vi "15 Puzzle Game (LabVIEW 2021).vi"() -> ()   [LabVIEW 2021]
uses:
  <vilib>/Utility/miscctls.llb/LVPositionTypeDef.ctl
panel:
  out "Moves Number":dbl caption="Elapsed Time (s)" format="%#.1f"
  out "Reset":bool
  out "Status":enum16{"Idle", "Start", "Stop"}(ring)
  out "Elapsed Time (s)":dbl format="%#.1f"
  out "Result":bool
  out "Temp Position":cluster{"Left":dbl, "Top":dbl}
  in  "Stop":bool
  in  "New Game":bool
  out "Empty":cluster{"Left":dbl, "Top":dbl}
  out "Random Array":dbl[](array[numeric])
  in  "Key 15":bool
  in  "Key 14":bool
  in  "Key 13":bool
  in  "Key 12":bool
  in  "Key 11":bool
  in  "Key 10":bool
  in  "Key 9":bool
  in  "Key 8":bool
  in  "Key 7":bool
  in  "Key 6":bool
  in  "Key 5":bool
  in  "Key 4":bool
  in  "Key 3":bool
  in  "Key 2":bool
  in  "Key 1":bool
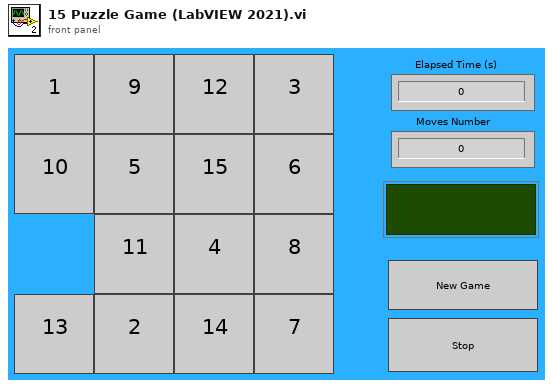
[diagram p1: front panel]
types:
  T1 = typedef "LVPositionTypeDef.ctl" = cluster{"Left":i32, "Top":i32}
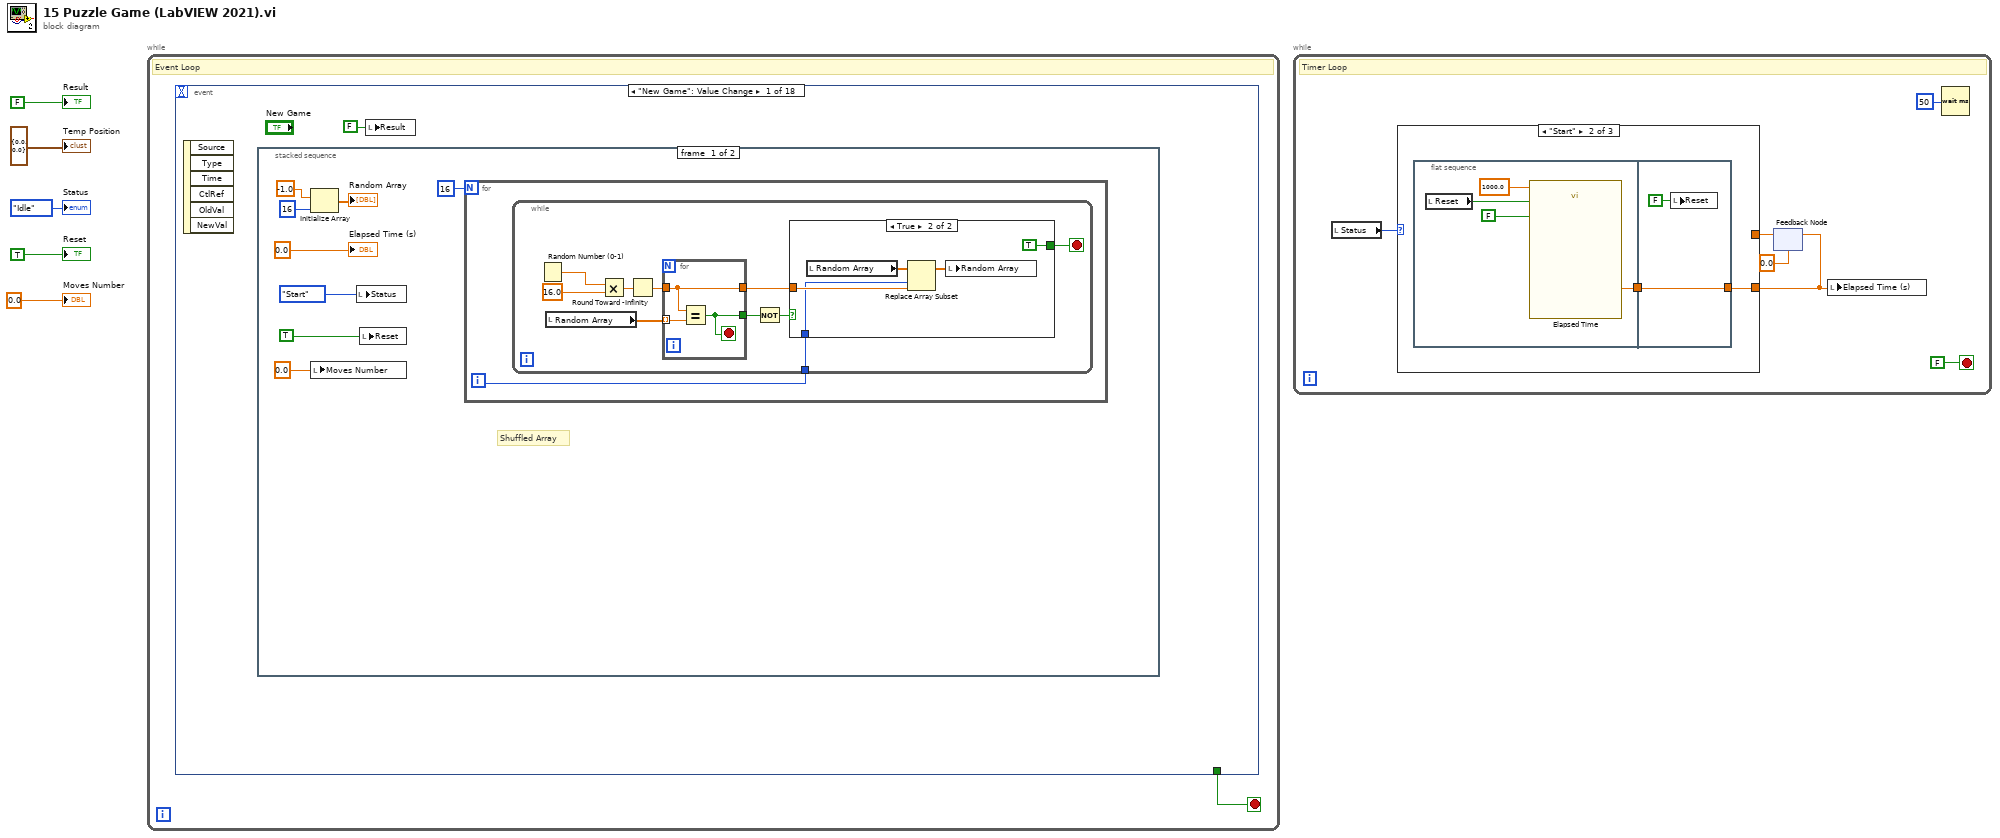
[diagram p0: block diagram]
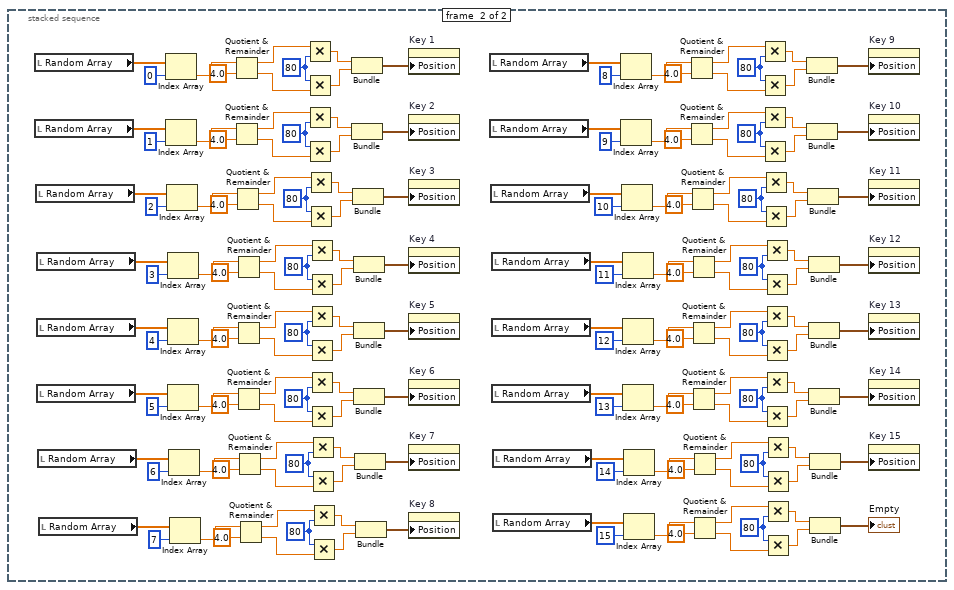
[diagram p5: hidden frame]
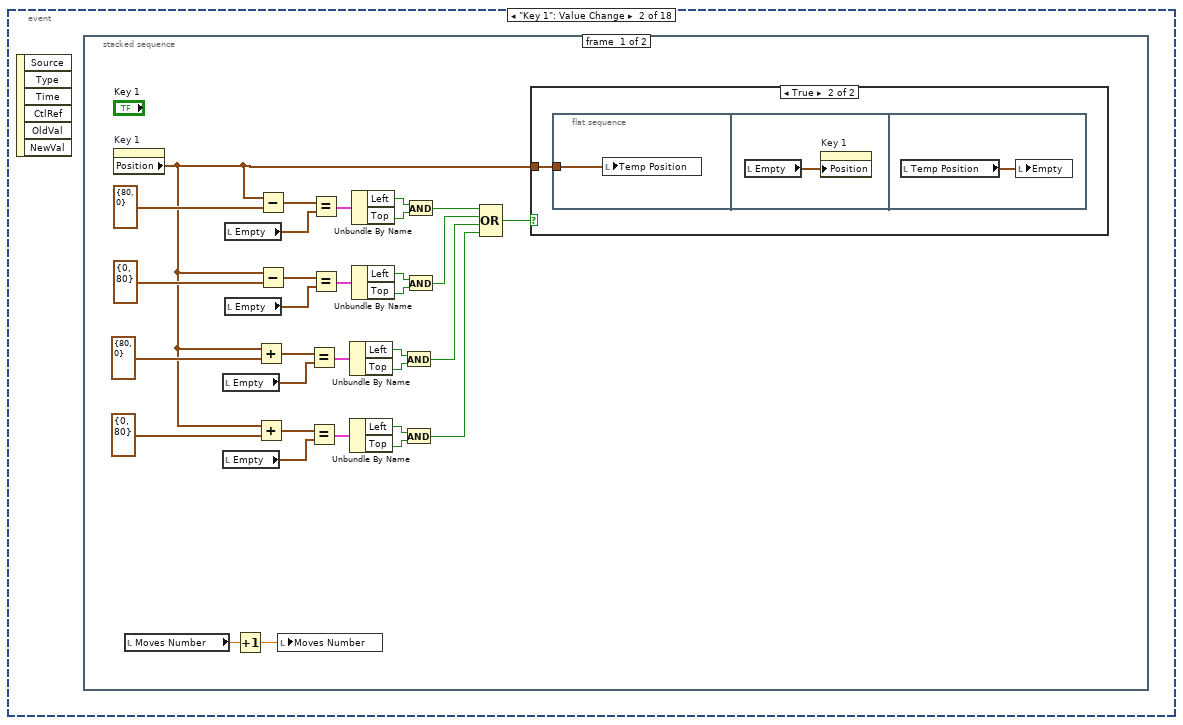
[diagram p6: hidden frame]
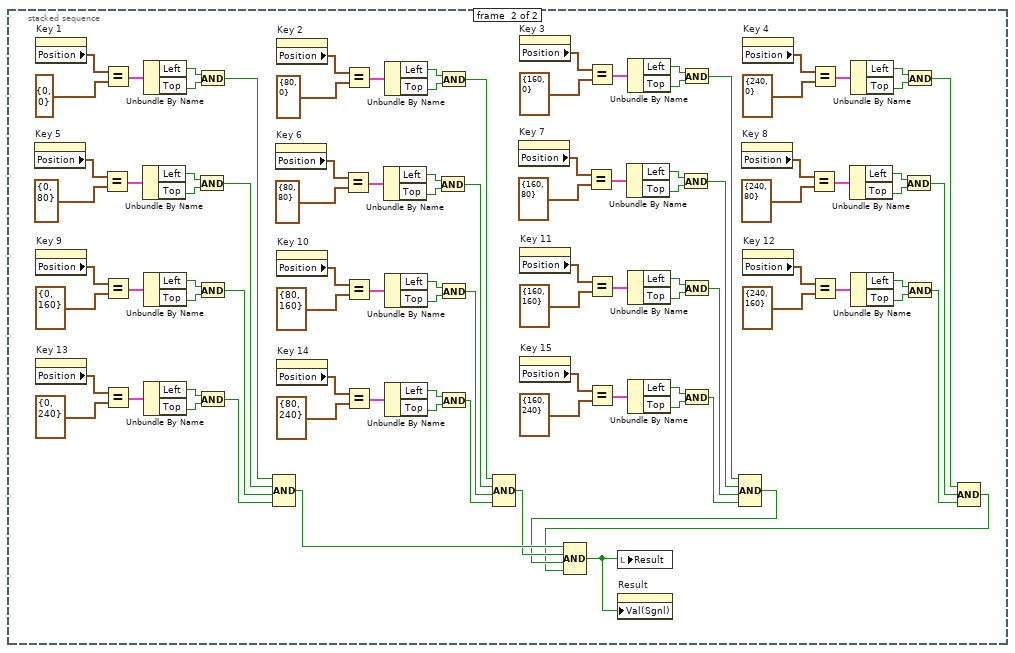
[diagram p8: hidden frame]
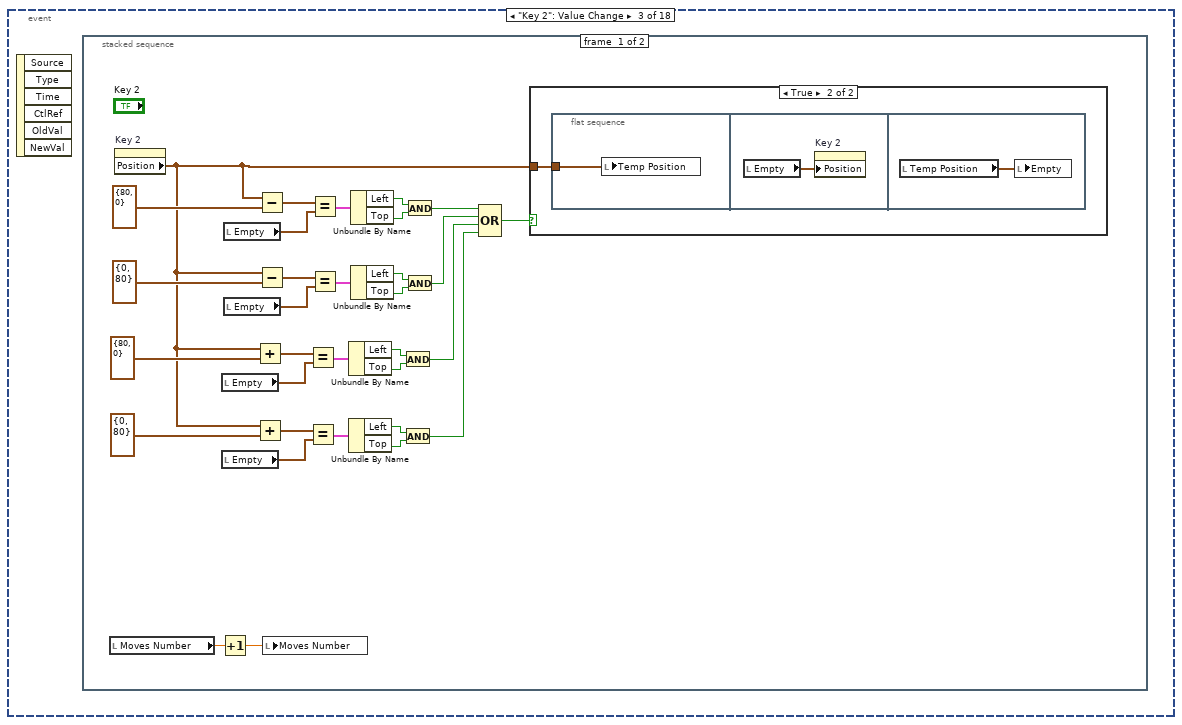
[diagram p9: hidden frame]
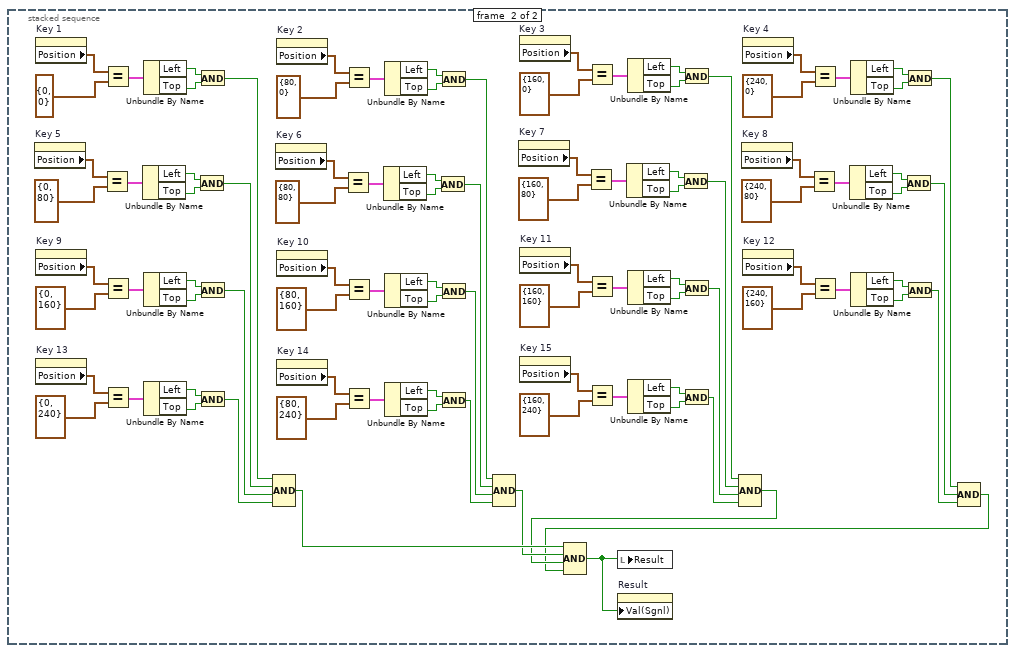
[diagram p11: hidden frame]
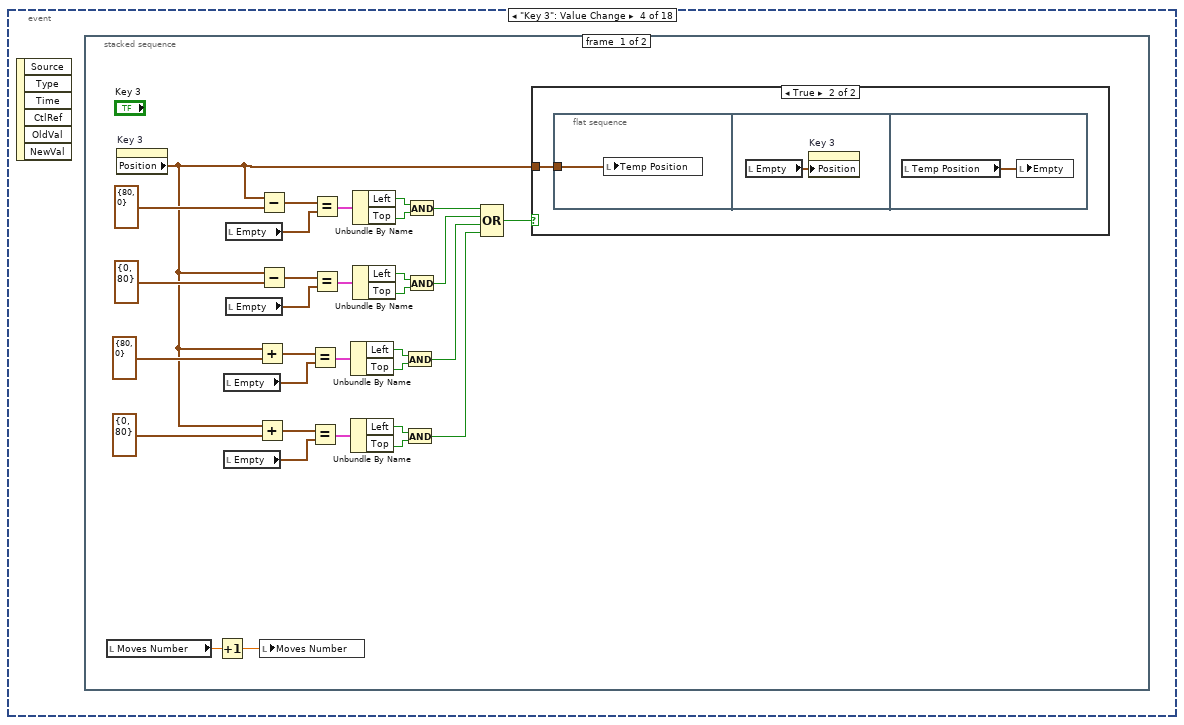
[diagram p12: hidden frame]
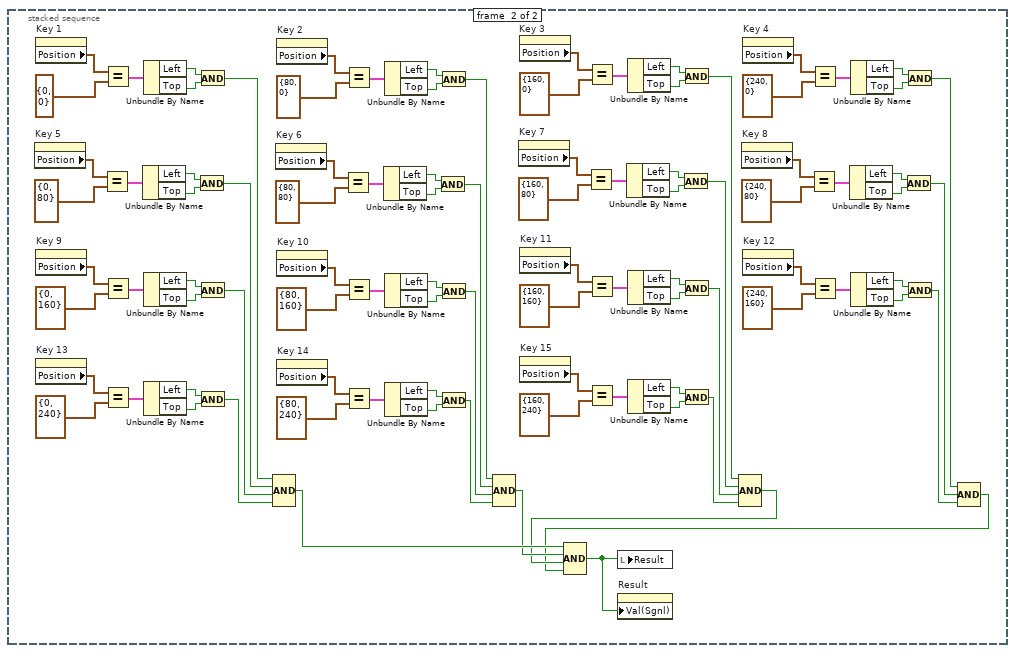
[diagram p14: hidden frame]
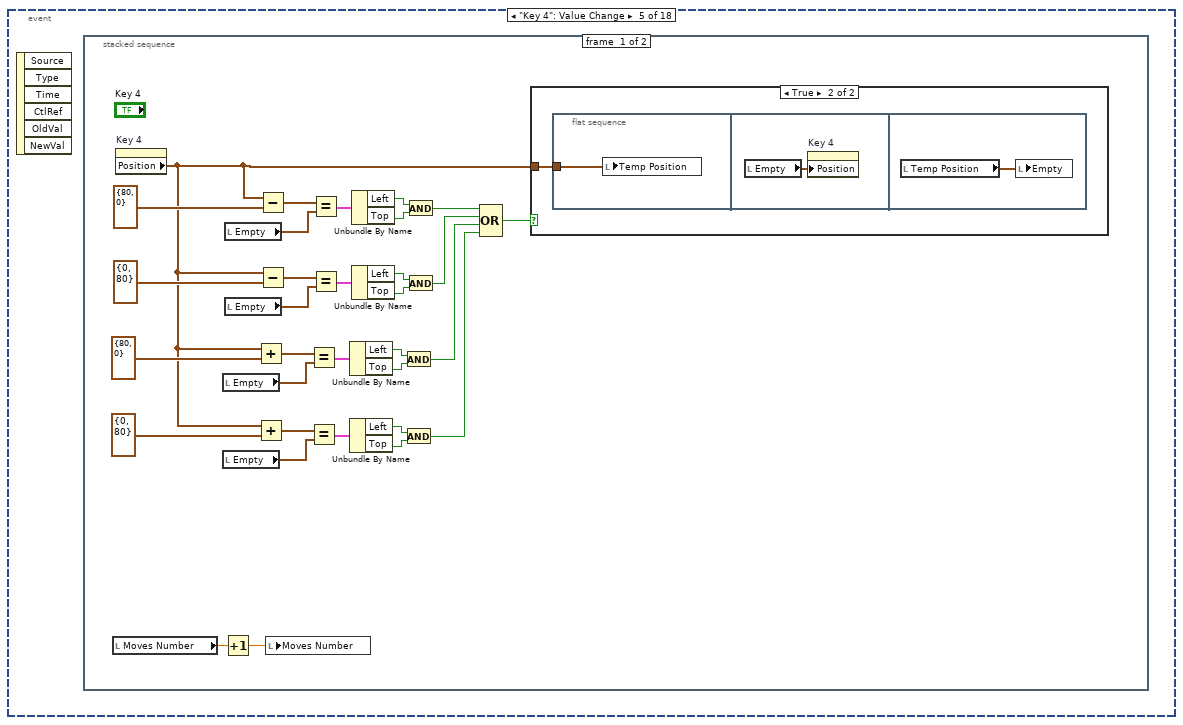
[diagram p15: hidden frame]
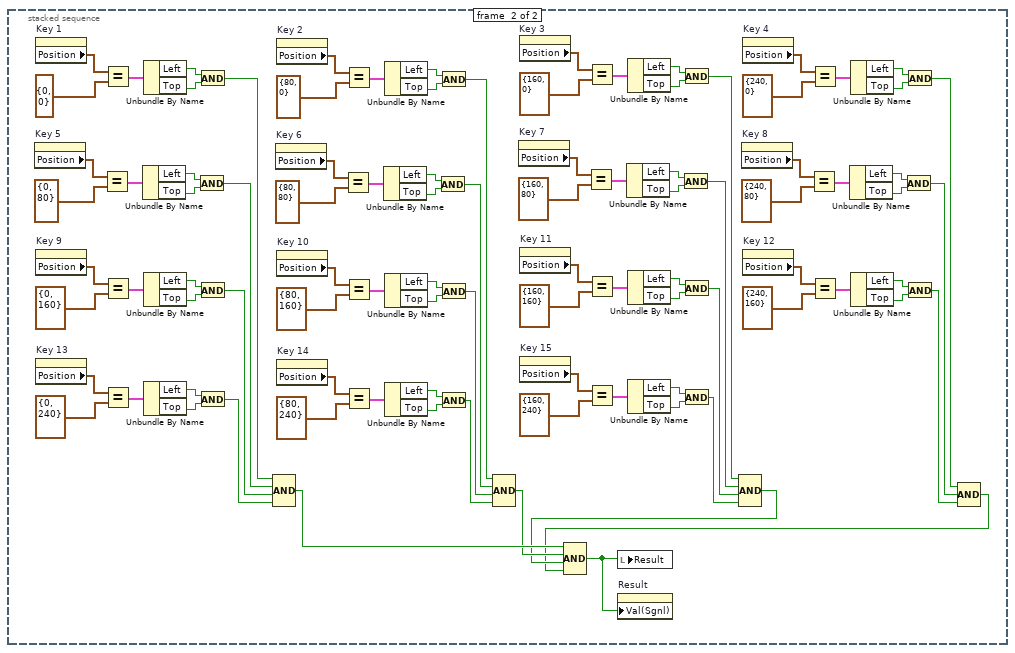
[diagram p17: hidden frame]
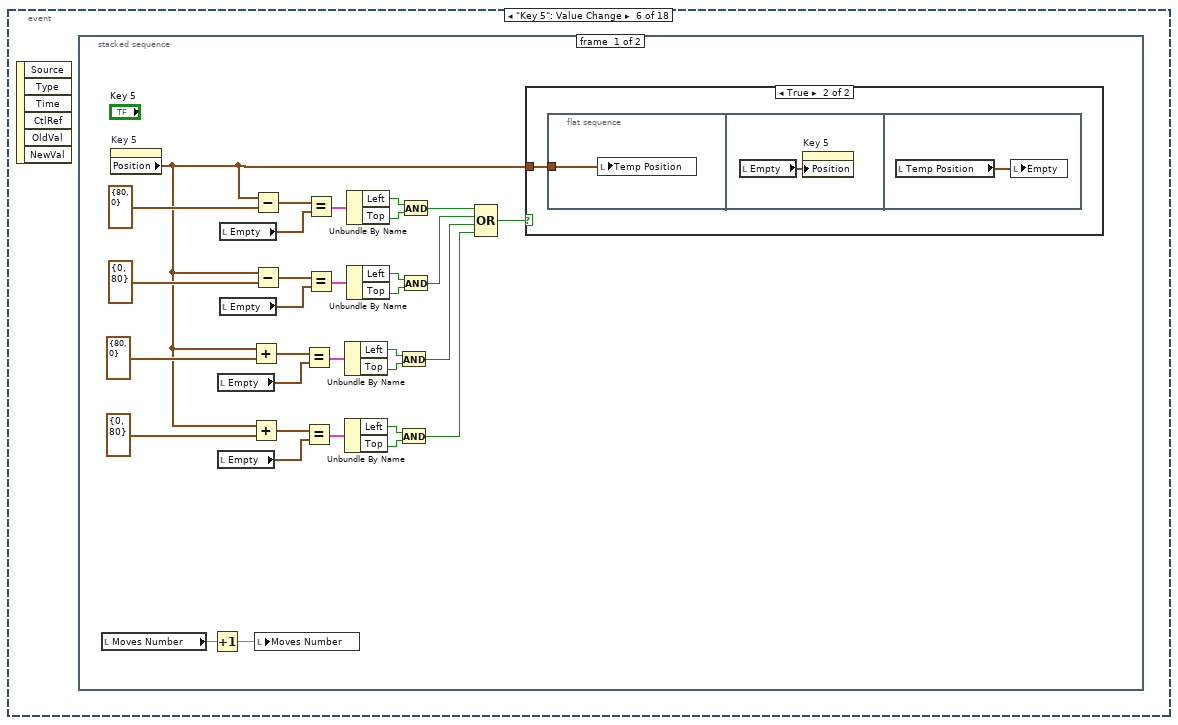
[diagram p18: hidden frame]
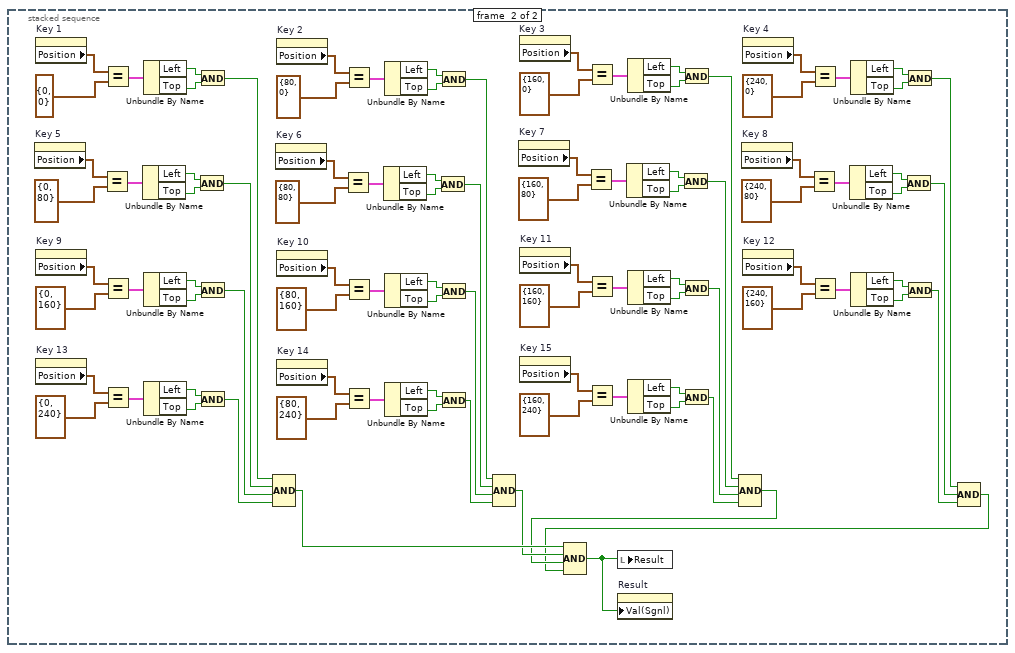
[diagram p20: hidden frame]
diagram:
  n1 = while {
    stop <- w6 stop-if-true
    # "Event Loop"
    n2 = event shown="[0] \"New Game\": Value Change" {
      selector: _ -> [_ _ _ _ _ _ _ _ _ _ _ _ _ _ _ _ _ _]
      dyn-events: _ -> [_ _ _ _ _ _ _ _ _ _ _ _ _ _ _ _ _ _]
      timeout: _ -> [_ _ _ _ _ _ _ _ _ _ _ _ _ _ _ _ _ _]
      tunnel: [_ _ _ _ _ _ _ _ _ _ _ _ _ _ _ _ _ TRUE] -> w6
      event "New Game": Value Change {
        n3 = event-data() -> ()  [unwired: 1 in, 6 out]
        n4 = stacked-sequence {
          frame #0 {
            # "Shuffled Array"
            n5 = Initialize Array(-1.0 ("element"), 16 ("dimension size")) -> (→"Random Array":dbl[])
            n6 = local write "Moves Number"(0.0 ("Moves Number")) -> ()
            n7 = local write "Status"(enum16{"Idle", "Start", "Stop"}."Start" ("Status")) -> ()
            n8 = local write "Reset"(TRUE ("Reset")) -> ()
            n9 = for {
              N: 16 -> [_]
              i -> [w16]
              n10 = while {
                tunnel: w16 -> [w17]
                stop <- w18 stop-if-true
                n11 = Random Number (0-1)() -> (number: 0 to 1=w21:dbl)
                n12 = local read "Random Array"() -> (w26:dbl[])
                n13 = Multiply(x=w21, y=16.0) -> (x*y=w22:dbl)
                n14 = Round Toward -Infinity(1:w22) -> (0:w19:dbl)
                n15 = for {
                  tunnel: w19 -> [w32]
                  tunnel: w26 -> [w34] mode=indexing
                  tunnel: [w33] -> w24
                  tunnel: [w32] -> w23
                  stop <- w33 stop-if-true
                  n16 = Equal?(x=w32, y=w34) -> (x = y?=w33:bool)
                }
                n17 = Not(x=w24) -> (.not. x?=w25:bool)
                n18 = case shown="True" w25 {
                  tunnel: w23 -> [_ w29]
                  tunnel: [_ TRUE] -> w18
                  tunnel: w17 -> [_ w27]
                  frame False {
                  }
                  frame True {
                    n19 = local read "Random Array"() -> (w31:dbl[])
                    n20 = Replace Array Subset(array=w31, new element=w29, index=w27) -> (w30:dbl[])
                    n21 = local write "Random Array"(w30) -> ()
                  }
                }
              }
            }
            "Elapsed Time (s)" <- 0.0 ("Elapsed Time (s)")
          }
          frame #1 {
            w42 = 80
            w88 = 80
            w101 = 80
            w108 = 80
            w78 = 80
            w71 = 80
            w58 = 80
            w51 = 80
            w148 = 80
            w141 = 80
            w128 = 80
            w121 = 80
            w161 = 80
            w168 = 80
            w181 = 80
            w188 = 80
            n22 = local read "Random Array"() -> (w194:dbl[])
            n23 = local read "Random Array"() -> (w175:dbl[])
            n24 = local read "Random Array"() -> (w174:dbl[])
            n25 = local read "Random Array"() -> (w155:dbl[])
            n26 = local read "Random Array"() -> (w115:dbl[])
            n27 = local read "Random Array"() -> (w134:dbl[])
            n28 = local read "Random Array"() -> (w135:dbl[])
            n29 = local read "Random Array"() -> (w154:dbl[])
            n30 = Index Array(array=w194, index=0) -> (element=w192:dbl)
            n31 = Index Array(array=w175, index=1) -> (element=w177:dbl)
            n32 = Index Array(array=w174, index=2) -> (element=w172:dbl)
            n33 = Index Array(array=w155, index=3) -> (element=w157:dbl)
            n34 = Index Array(array=w115, index=4) -> (element=w117:dbl)
            n35 = Index Array(array=w134, index=5) -> (element=w132:dbl)
            n36 = Index Array(array=w135, index=6) -> (element=w137:dbl)
            n37 = Index Array(array=w154, index=7) -> (element=w152:dbl)
            n38 = Quotient & Remainder(x=w192, y=4.0) -> (x-y*floor(x/y)=w190:dbl, floor(x/y)=w189:dbl)
            n39 = Quotient & Remainder(x=w177, y=4.0) -> (x-y*floor(x/y)=w179:dbl, floor(x/y)=w180:dbl)
            n40 = Quotient & Remainder(x=w172, y=4.0) -> (x-y*floor(x/y)=w170:dbl, floor(x/y)=w169:dbl)
            n41 = Quotient & Remainder(x=w157, y=4.0) -> (x-y*floor(x/y)=w159:dbl, floor(x/y)=w160:dbl)
            n42 = Quotient & Remainder(x=w117, y=4.0) -> (x-y*floor(x/y)=w119:dbl, floor(x/y)=w120:dbl)
            n43 = Quotient & Remainder(x=w132, y=4.0) -> (x-y*floor(x/y)=w130:dbl, floor(x/y)=w129:dbl)
            n44 = Quotient & Remainder(x=w137, y=4.0) -> (x-y*floor(x/y)=w139:dbl, floor(x/y)=w140:dbl)
            n45 = Quotient & Remainder(x=w152, y=4.0) -> (x-y*floor(x/y)=w150:dbl, floor(x/y)=w149:dbl)
            n46 = Multiply(x=w190, y=w188) -> (x*y=w187:dbl)
            n47 = Multiply(x=w188, y=w189) -> (x*y=w186:dbl)
            n48 = Multiply(x=w179, y=w181) -> (x*y=w182:dbl)
            n49 = Multiply(x=w181, y=w180) -> (x*y=w183:dbl)
            n50 = Multiply(x=w170, y=w168) -> (x*y=w167:dbl)
            n51 = Multiply(x=w168, y=w169) -> (x*y=w166:dbl)
            n52 = Multiply(x=w159, y=w161) -> (x*y=w162:dbl)
            n53 = Multiply(x=w161, y=w160) -> (x*y=w163:dbl)
            n54 = Multiply(x=w119, y=w121) -> (x*y=w122:dbl)
            n55 = Multiply(x=w121, y=w120) -> (x*y=w123:dbl)
            n56 = Multiply(x=w130, y=w128) -> (x*y=w127:dbl)
            n57 = Multiply(x=w128, y=w129) -> (x*y=w126:dbl)
            n58 = Multiply(x=w139, y=w141) -> (x*y=w142:dbl)
            n59 = Multiply(x=w141, y=w140) -> (x*y=w143:dbl)
            n60 = Multiply(x=w150, y=w148) -> (x*y=w147:dbl)
            n61 = Multiply(x=w148, y=w149) -> (x*y=w146:dbl)
            n62 = Bundle(w187, w186) -> (w185:cluster{dbl, dbl})  [unwired: 1 in]
            n63 = Bundle(w182, w183) -> (w184:cluster{dbl, dbl})  [unwired: 1 in]
            n64 = Bundle(w167, w166) -> (w165:cluster{dbl, dbl})  [unwired: 1 in]
            n65 = Bundle(w162, w163) -> (w164:cluster{dbl, dbl})  [unwired: 1 in]
            n66 = Bundle(w122, w123) -> (w124:cluster{dbl, dbl})  [unwired: 1 in]
            n67 = Bundle(w127, w126) -> (w125:cluster{dbl, dbl})  [unwired: 1 in]
            n68 = Bundle(w142, w143) -> (w144:cluster{dbl, dbl})  [unwired: 1 in]
            n69 = Bundle(w147, w146) -> (w145:cluster{dbl, dbl})  [unwired: 1 in]
            n70 = property on="Key 1" class="Bool"("Position"=w185) -> ()  [unwired: 2 in, 2 out]
            n71 = property on="Key 2" class="Bool"("Position"=w184) -> ()  [unwired: 2 in, 2 out]
            n72 = property on="Key 3" class="Bool"("Position"=w165) -> ()  [unwired: 2 in, 2 out]
            n73 = property on="Key 4" class="Bool"("Position"=w164) -> ()  [unwired: 2 in, 2 out]
            n74 = property on="Key 5" class="Bool"("Position"=w124) -> ()  [unwired: 2 in, 2 out]
            n75 = property on="Key 6" class="Bool"("Position"=w125) -> ()  [unwired: 2 in, 2 out]
            n76 = property on="Key 7" class="Bool"("Position"=w144) -> ()  [unwired: 2 in, 2 out]
            n77 = property on="Key 8" class="Bool"("Position"=w145) -> ()  [unwired: 2 in, 2 out]
            n78 = local read "Random Array"() -> (w45:dbl[])
            n79 = local read "Random Array"() -> (w64:dbl[])
            n80 = local read "Random Array"() -> (w65:dbl[])
            n81 = local read "Random Array"() -> (w84:dbl[])
            n82 = local read "Random Array"() -> (w114:dbl[])
            n83 = local read "Random Array"() -> (w95:dbl[])
            n84 = local read "Random Array"() -> (w94:dbl[])
            n85 = local read "Random Array"() -> (w36:dbl[])
            n86 = Index Array(array=w45, index=8) -> (element=w47:dbl)
            n87 = Index Array(array=w64, index=9) -> (element=w62:dbl)
            n88 = Index Array(array=w65, index=10) -> (element=w67:dbl)
            n89 = Index Array(array=w84, index=11) -> (element=w82:dbl)
            n90 = Index Array(array=w114, index=12) -> (element=w112:dbl)
            n91 = Index Array(array=w95, index=13) -> (element=w97:dbl)
            n92 = Index Array(array=w94, index=14) -> (element=w92:dbl)
            n93 = Index Array(array=w36, index=15) -> (element=w38:dbl)
            n94 = Quotient & Remainder(x=w47, y=4.0) -> (x-y*floor(x/y)=w49:dbl, floor(x/y)=w50:dbl)
            n95 = Quotient & Remainder(x=w62, y=4.0) -> (x-y*floor(x/y)=w60:dbl, floor(x/y)=w59:dbl)
            n96 = Quotient & Remainder(x=w67, y=4.0) -> (x-y*floor(x/y)=w69:dbl, floor(x/y)=w70:dbl)
            n97 = Quotient & Remainder(x=w82, y=4.0) -> (x-y*floor(x/y)=w80:dbl, floor(x/y)=w79:dbl)
            n98 = Quotient & Remainder(x=w112, y=4.0) -> (x-y*floor(x/y)=w110:dbl, floor(x/y)=w109:dbl)
            n99 = Quotient & Remainder(x=w97, y=4.0) -> (x-y*floor(x/y)=w99:dbl, floor(x/y)=w100:dbl)
            n100 = Quotient & Remainder(x=w92, y=4.0) -> (x-y*floor(x/y)=w90:dbl, floor(x/y)=w89:dbl)
            n101 = Quotient & Remainder(x=w38, y=4.0) -> (x-y*floor(x/y)=w40:dbl, floor(x/y)=w41:dbl)
            n102 = Multiply(x=w49, y=w51) -> (x*y=w52:dbl)
            n103 = Multiply(x=w51, y=w50) -> (x*y=w53:dbl)
            n104 = Multiply(x=w60, y=w58) -> (x*y=w57:dbl)
            n105 = Multiply(x=w58, y=w59) -> (x*y=w56:dbl)
            n106 = Multiply(x=w69, y=w71) -> (x*y=w72:dbl)
            n107 = Multiply(x=w71, y=w70) -> (x*y=w73:dbl)
            n108 = Multiply(x=w80, y=w78) -> (x*y=w77:dbl)
            n109 = Multiply(x=w78, y=w79) -> (x*y=w76:dbl)
            n110 = Multiply(x=w110, y=w108) -> (x*y=w107:dbl)
            n111 = Multiply(x=w108, y=w109) -> (x*y=w106:dbl)
            n112 = Multiply(x=w99, y=w101) -> (x*y=w102:dbl)
            n113 = Multiply(x=w101, y=w100) -> (x*y=w103:dbl)
            n114 = Multiply(x=w90, y=w88) -> (x*y=w87:dbl)
            n115 = Multiply(x=w88, y=w89) -> (x*y=w86:dbl)
            n116 = Multiply(x=w40, y=w42) -> (x*y=w43:dbl)
            n117 = Multiply(x=w42, y=w41) -> (x*y=w44:dbl)
            n118 = Bundle(w52, w53) -> (w54:cluster{dbl, dbl})  [unwired: 1 in]
            n119 = Bundle(w57, w56) -> (w55:cluster{dbl, dbl})  [unwired: 1 in]
            n120 = Bundle(w72, w73) -> (w74:cluster{dbl, dbl})  [unwired: 1 in]
            n121 = Bundle(w77, w76) -> (w75:cluster{dbl, dbl})  [unwired: 1 in]
            n122 = Bundle(w107, w106) -> (w105:cluster{dbl, dbl})  [unwired: 1 in]
            n123 = Bundle(w102, w103) -> (w104:cluster{dbl, dbl})  [unwired: 1 in]
            n124 = Bundle(w87, w86) -> (w85:cluster{dbl, dbl})  [unwired: 1 in]
            n125 = Bundle(w43, w44) -> (→"Empty":cluster{dbl, dbl})  [unwired: 1 in]
            n126 = property on="Key 9" class="Bool"("Position"=w54) -> ()  [unwired: 2 in, 2 out]
            n127 = property on="Key 10" class="Bool"("Position"=w55) -> ()  [unwired: 2 in, 2 out]
            n128 = property on="Key 11" class="Bool"("Position"=w74) -> ()  [unwired: 2 in, 2 out]
            n129 = property on="Key 12" class="Bool"("Position"=w75) -> ()  [unwired: 2 in, 2 out]
            n130 = property on="Key 13" class="Bool"("Position"=w105) -> ()  [unwired: 2 in, 2 out]
            n131 = property on="Key 14" class="Bool"("Position"=w104) -> ()  [unwired: 2 in, 2 out]
            n132 = property on="Key 15" class="Bool"("Position"=w85) -> ()  [unwired: 2 in, 2 out]
          }
        }
        n133 = local write "Result"(FALSE ("Result")) -> ()
      }
      event "Key 1": Value Change {
        n134 = event-data() -> ()  [unwired: 1 in, 6 out]
        n135 = stacked-sequence {
          frame #0 {
            n136 = property on="Key 1" class="Bool"() -> ("Position"=w197:T1)  [unwired: 2 in, 2 out]
            n137 = local read "Moves Number"() -> (w195:dbl)
            n138 = local read "Empty"() -> (w205:cluster{"Left":dbl, "Top":dbl})
            n139 = local read "Empty"() -> (w212:cluster{"Left":dbl, "Top":dbl})
            n140 = local read "Empty"() -> (w224:cluster{"Left":dbl, "Top":dbl})
            n141 = local read "Empty"() -> (w217:cluster{"Left":dbl, "Top":dbl})
            n142 = Increment(x=w195) -> (x+1=w196:dbl)
            n143 = Add(x=w197, y=T1 {"Left"=80, "Top"=0} ("Position")) -> (x+y=w204:T1)
            n144 = Add(x=w197, y=T1 {"Left"=0, "Top"=80} ("Position")) -> (x+y=w213:T1)
            n145 = Subtract(x=w197, y=T1 {"Left"=80, "Top"=0} ("Position")) -> (x-y=w225:T1)
            n146 = Subtract(x=w197, y=T1 {"Left"=0, "Top"=80} ("Position")) -> (x-y=w216:T1)
            n147 = local write "Moves Number"(w196) -> ()
            n148 = Equal?(x=w204, y=w205) -> (x = y?=w206:cluster{"Left":bool, "Top":bool})
            n149 = Equal?(x=w213, y=w212) -> (x = y?=w211:cluster{"Left":bool, "Top":bool})
            n150 = Equal?(x=w225, y=w224) -> (x = y?=w223:cluster{"Left":bool, "Top":bool})
            n151 = Equal?(x=w216, y=w217) -> (x = y?=w218:cluster{"Left":bool, "Top":bool})
            n152 = Unbundle By Name(w206) -> ("Left"=w208:bool, "Top"=w207:bool)
            n153 = Unbundle By Name(w211) -> ("Left"=w209:bool, "Top"=w210:bool)
            n154 = Unbundle By Name(w223) -> ("Left"=w221:bool, "Top"=w222:bool)
            n155 = Unbundle By Name(w218) -> ("Left"=w220:bool, "Top"=w219:bool)
            n156 = And(x=w208, y=w207) -> (x .and. y?=w199:bool)
            n157 = And(x=w209, y=w210) -> (x .and. y?=w198:bool)
            n158 = And(x=w221, y=w222) -> (x .and. y?=w201:bool)
            n159 = And(x=w220, y=w219) -> (x .and. y?=w200:bool)
            n160 = Compound Arithmetic op=OR(w201, w200, w199, w198) -> (w202:bool)
            n161 = case shown="True" w202 {
              tunnel: w197 -> [_ w227]
              frame False {
              }
              frame True {
                n162 = flat-sequence {
                  tunnel: w227 -> [w228]
                  frame #0 {
                    n163 = local write "Temp Position"(w228) -> ()
                  }
                  frame #1 {
                    n164 = local read "Empty"() -> (w229:cluster{"Left":dbl, "Top":dbl})
                    n165 = property on="Key 1" class="Bool"("Position"=w229) -> ()  [unwired: 2 in, 2 out]
                  }
                  frame #2 {
                    n166 = local read "Temp Position"() -> (w230:cluster{"Left":dbl, "Top":dbl})
                    n167 = local write "Empty"(w230) -> ()
                  }
                }
              }
            }
          }
          frame #1 {
            n168 = property on="Key 5" class="Bool"() -> ("Position"=w319:T1)  [unwired: 2 in, 2 out]
            n169 = property on="Key 1" class="Bool"() -> ("Position"=w322:T1)  [unwired: 2 in, 2 out]
            n170 = property on="Key 9" class="Bool"() -> ("Position"=w312:T1)  [unwired: 2 in, 2 out]
            n171 = property on="Key 13" class="Bool"() -> ("Position"=w309:T1)  [unwired: 2 in, 2 out]
            n172 = Equal?(x=w319, y=T1 {"Left"=0, "Top"=80} ("Position")) -> (x = y?=w316:cluster{"Left":bool, "Top":bool})
            n173 = Equal?(x=w322, y=T1 {"Left"=0, "Top"=0} ("Position")) -> (x = y?=w325:cluster{"Left":bool, "Top":bool})
            n174 = Equal?(x=w312, y=T1 {"Left"=0, "Top"=160} ("Position")) -> (x = y?=w315:cluster{"Left":bool, "Top":bool})
            n175 = Equal?(x=w309, y=T1 {"Left"=0, "Top"=240} ("Position")) -> (x = y?=w306:cluster{"Left":bool, "Top":bool})
            n176 = Unbundle By Name(w316) -> ("Left"=w318:bool, "Top"=w317:bool)
            n177 = Unbundle By Name(w325) -> ("Left"=w323:bool, "Top"=w324:bool)
            n178 = Unbundle By Name(w315) -> ("Left"=w313:bool, "Top"=w314:bool)
            n179 = Unbundle By Name(w306) -> ("Left"=w308:bool, "Top"=w307:bool)
            n180 = And(x=w318, y=w317) -> (x .and. y?=w249:bool)
            n181 = And(x=w323, y=w324) -> (x .and. y?=w250:bool)
            n182 = And(x=w313, y=w314) -> (x .and. y?=w248:bool)
            n183 = And(x=w308, y=w307) -> (x .and. y?=w247:bool)
            n184 = Compound Arithmetic op=AND(w250, w249, w248, w247) -> (w235:bool)
            n185 = property on="Key 6" class="Bool"() -> ("Position"=w292:T1)  [unwired: 2 in, 2 out]
            n186 = property on="Key 2" class="Bool"() -> ("Position"=w289:T1)  [unwired: 2 in, 2 out]
            n187 = property on="Key 10" class="Bool"() -> ("Position"=w299:T1)  [unwired: 2 in, 2 out]
            n188 = property on="Key 14" class="Bool"() -> ("Position"=w302:T1)  [unwired: 2 in, 2 out]
            n189 = Equal?(x=w292, y=T1 {"Left"=80, "Top"=80} ("Position")) -> (x = y?=w295:cluster{"Left":bool, "Top":bool})
            n190 = Equal?(x=w289, y=T1 {"Left"=80, "Top"=0} ("Position")) -> (x = y?=w286:cluster{"Left":bool, "Top":bool})
            n191 = Equal?(x=w299, y=T1 {"Left"=80, "Top"=160} ("Position")) -> (x = y?=w296:cluster{"Left":bool, "Top":bool})
            n192 = Equal?(x=w302, y=T1 {"Left"=80, "Top"=240} ("Position")) -> (x = y?=w305:cluster{"Left":bool, "Top":bool})
            n193 = Unbundle By Name(w295) -> ("Left"=w293:bool, "Top"=w294:bool)
            n194 = Unbundle By Name(w286) -> ("Left"=w288:bool, "Top"=w287:bool)
            n195 = Unbundle By Name(w296) -> ("Left"=w298:bool, "Top"=w297:bool)
            n196 = Unbundle By Name(w305) -> ("Left"=w303:bool, "Top"=w304:bool)
            n197 = And(x=w293, y=w294) -> (x .and. y?=w245:bool)
            n198 = And(x=w288, y=w287) -> (x .and. y?=w246:bool)
            n199 = And(x=w298, y=w297) -> (x .and. y?=w244:bool)
            n200 = And(x=w303, y=w304) -> (x .and. y?=w243:bool)
            n201 = Compound Arithmetic op=AND(w246, w245, w244, w243) -> (w234:bool)
            n202 = property on="Key 7" class="Bool"() -> ("Position"=w279:T1)  [unwired: 2 in, 2 out]
            n203 = property on="Key 3" class="Bool"() -> ("Position"=w282:T1)  [unwired: 2 in, 2 out]
            n204 = property on="Key 11" class="Bool"() -> ("Position"=w272:T1)  [unwired: 2 in, 2 out]
            n205 = property on="Key 15" class="Bool"() -> ("Position"=w269:T1)  [unwired: 2 in, 2 out]
            n206 = Equal?(x=w279, y=T1 {"Left"=160, "Top"=80} ("Position")) -> (x = y?=w276:cluster{"Left":bool, "Top":bool})
            n207 = Equal?(x=w282, y=T1 {"Left"=160, "Top"=0} ("Position")) -> (x = y?=w285:cluster{"Left":bool, "Top":bool})
            n208 = Equal?(x=w272, y=T1 {"Left"=160, "Top"=160} ("Position")) -> (x = y?=w275:cluster{"Left":bool, "Top":bool})
            n209 = Equal?(x=w269, y=T1 {"Left"=160, "Top"=240} ("Position")) -> (x = y?=w266:cluster{"Left":bool, "Top":bool})
            n210 = Unbundle By Name(w276) -> ("Left"=w278:bool, "Top"=w277:bool)
            n211 = Unbundle By Name(w285) -> ("Left"=w283:bool, "Top"=w284:bool)
            n212 = Unbundle By Name(w275) -> ("Left"=w273:bool, "Top"=w274:bool)
            n213 = Unbundle By Name(w266) -> ("Left"=w268:bool, "Top"=w267:bool)
            n214 = And(x=w278, y=w277) -> (x .and. y?=w241:bool)
            n215 = And(x=w283, y=w284) -> (x .and. y?=w242:bool)
            n216 = And(x=w273, y=w274) -> (x .and. y?=w240:bool)
            n217 = And(x=w268, y=w267) -> (x .and. y?=w239:bool)
            n218 = Compound Arithmetic op=AND(w242, w241, w240, w239) -> (w233:bool)
            n219 = property on="Key 8" class="Bool"() -> ("Position"=w257:T1)  [unwired: 2 in, 2 out]
            n220 = property on="Key 4" class="Bool"() -> ("Position"=w254:T1)  [unwired: 2 in, 2 out]
            n221 = property on="Key 12" class="Bool"() -> ("Position"=w264:T1)  [unwired: 2 in, 2 out]
            n222 = Equal?(x=w257, y=T1 {"Left"=240, "Top"=80} ("Position")) -> (x = y?=w260:cluster{"Left":bool, "Top":bool})
            n223 = Equal?(x=w254, y=T1 {"Left"=240, "Top"=0} ("Position")) -> (x = y?=w251:cluster{"Left":bool, "Top":bool})
            n224 = Equal?(x=w264, y=T1 {"Left"=240, "Top"=160} ("Position")) -> (x = y?=w261:cluster{"Left":bool, "Top":bool})
            n225 = Unbundle By Name(w260) -> ("Left"=w258:bool, "Top"=w259:bool)
            n226 = Unbundle By Name(w251) -> ("Left"=w253:bool, "Top"=w252:bool)
            n227 = Unbundle By Name(w261) -> ("Left"=w263:bool, "Top"=w262:bool)
            n228 = And(x=w258, y=w259) -> (x .and. y?=w237:bool)
            n229 = And(x=w253, y=w252) -> (x .and. y?=w238:bool)
            n230 = And(x=w263, y=w262) -> (x .and. y?=w236:bool)
            n231 = Compound Arithmetic op=AND(w238, w237, w236) -> (w232:bool)
            n232 = Compound Arithmetic op=AND(w235, w234, w233, w232) -> (w231:bool)
            n233 = local write "Result"(w231) -> ()
            n234 = property on="Result" class="Bool (strict)"("Val(Sgnl)"=w231) -> ()  [unwired: 2 in, 2 out]
          }
        }
      }
      event "Key 2": Value Change {
        n235 = event-data() -> ()  [unwired: 1 in, 6 out]
        n236 = stacked-sequence {
          frame #0 {
            n237 = local read "Moves Number"() -> (w326:dbl)
            n238 = property on="Key 2" class="Bool"() -> ("Position"=w328:T1)  [unwired: 2 in, 2 out]
            n239 = Increment(x=w326) -> (x+1=w327:dbl)
            n240 = local read "Empty"() -> (w336:cluster{"Left":dbl, "Top":dbl})
            n241 = local read "Empty"() -> (w343:cluster{"Left":dbl, "Top":dbl})
            n242 = local read "Empty"() -> (w355:cluster{"Left":dbl, "Top":dbl})
            n243 = local read "Empty"() -> (w348:cluster{"Left":dbl, "Top":dbl})
            n244 = Add(x=w328, y=T1 {"Left"=80, "Top"=0} ("Position")) -> (x+y=w335:T1)
            n245 = Add(x=w328, y=T1 {"Left"=0, "Top"=80} ("Position")) -> (x+y=w344:T1)
            n246 = Subtract(x=w328, y=T1 {"Left"=80, "Top"=0} ("Position")) -> (x-y=w356:T1)
            n247 = Subtract(x=w328, y=T1 {"Left"=0, "Top"=80} ("Position")) -> (x-y=w347:T1)
            n248 = local write "Moves Number"(w327) -> ()
            n249 = Equal?(x=w335, y=w336) -> (x = y?=w337:cluster{"Left":bool, "Top":bool})
            n250 = Equal?(x=w344, y=w343) -> (x = y?=w342:cluster{"Left":bool, "Top":bool})
            n251 = Equal?(x=w356, y=w355) -> (x = y?=w354:cluster{"Left":bool, "Top":bool})
            n252 = Equal?(x=w347, y=w348) -> (x = y?=w349:cluster{"Left":bool, "Top":bool})
            n253 = Unbundle By Name(w337) -> ("Left"=w339:bool, "Top"=w338:bool)
            n254 = Unbundle By Name(w342) -> ("Left"=w340:bool, "Top"=w341:bool)
            n255 = Unbundle By Name(w354) -> ("Left"=w352:bool, "Top"=w353:bool)
            n256 = Unbundle By Name(w349) -> ("Left"=w351:bool, "Top"=w350:bool)
            n257 = And(x=w339, y=w338) -> (x .and. y?=w330:bool)
            n258 = And(x=w340, y=w341) -> (x .and. y?=w329:bool)
            n259 = And(x=w352, y=w353) -> (x .and. y?=w332:bool)
            n260 = And(x=w351, y=w350) -> (x .and. y?=w331:bool)
            n261 = Compound Arithmetic op=OR(w332, w331, w330, w329) -> (w333:bool)
            n262 = case shown="True" w333 {
              tunnel: w328 -> [_ w358]
              frame False {
              }
              frame True {
                n263 = flat-sequence {
                  tunnel: w358 -> [w359]
                  frame #0 {
                    n264 = local write "Temp Position"(w359) -> ()
                  }
                  frame #1 {
                    n265 = local read "Empty"() -> (w360:cluster{"Left":dbl, "Top":dbl})
                    n266 = property on="Key 2" class="Bool"("Position"=w360) -> ()  [unwired: 2 in, 2 out]
                  }
                  frame #2 {
                    n267 = local read "Temp Position"() -> (w361:cluster{"Left":dbl, "Top":dbl})
                    n268 = local write "Empty"(w361) -> ()
                  }
                }
              }
            }
          }
          frame #1 {
            n269 = property on="Key 5" class="Bool"() -> ("Position"=w450:T1)  [unwired: 2 in, 2 out]
            n270 = property on="Key 1" class="Bool"() -> ("Position"=w453:T1)  [unwired: 2 in, 2 out]
            n271 = property on="Key 9" class="Bool"() -> ("Position"=w443:T1)  [unwired: 2 in, 2 out]
            n272 = property on="Key 13" class="Bool"() -> ("Position"=w440:T1)  [unwired: 2 in, 2 out]
            n273 = Equal?(x=w450, y=T1 {"Left"=0, "Top"=80} ("Position")) -> (x = y?=w447:cluster{"Left":bool, "Top":bool})
            n274 = Equal?(x=w453, y=T1 {"Left"=0, "Top"=0} ("Position")) -> (x = y?=w456:cluster{"Left":bool, "Top":bool})
            n275 = Equal?(x=w443, y=T1 {"Left"=0, "Top"=160} ("Position")) -> (x = y?=w446:cluster{"Left":bool, "Top":bool})
            n276 = Equal?(x=w440, y=T1 {"Left"=0, "Top"=240} ("Position")) -> (x = y?=w437:cluster{"Left":bool, "Top":bool})
            n277 = Unbundle By Name(w447) -> ("Left"=w449:bool, "Top"=w448:bool)
            n278 = Unbundle By Name(w456) -> ("Left"=w454:bool, "Top"=w455:bool)
            n279 = Unbundle By Name(w446) -> ("Left"=w444:bool, "Top"=w445:bool)
            n280 = Unbundle By Name(w437) -> ("Left"=w439:bool, "Top"=w438:bool)
            n281 = And(x=w449, y=w448) -> (x .and. y?=w380:bool)
            n282 = And(x=w454, y=w455) -> (x .and. y?=w381:bool)
            n283 = And(x=w444, y=w445) -> (x .and. y?=w379:bool)
            n284 = And(x=w439, y=w438) -> (x .and. y?=w378:bool)
            n285 = Compound Arithmetic op=AND(w381, w380, w379, w378) -> (w366:bool)
            n286 = property on="Key 6" class="Bool"() -> ("Position"=w423:T1)  [unwired: 2 in, 2 out]
            n287 = property on="Key 2" class="Bool"() -> ("Position"=w420:T1)  [unwired: 2 in, 2 out]
            n288 = property on="Key 10" class="Bool"() -> ("Position"=w430:T1)  [unwired: 2 in, 2 out]
            n289 = property on="Key 14" class="Bool"() -> ("Position"=w433:T1)  [unwired: 2 in, 2 out]
            n290 = Equal?(x=w423, y=T1 {"Left"=80, "Top"=80} ("Position")) -> (x = y?=w426:cluster{"Left":bool, "Top":bool})
            n291 = Equal?(x=w420, y=T1 {"Left"=80, "Top"=0} ("Position")) -> (x = y?=w417:cluster{"Left":bool, "Top":bool})
            n292 = Equal?(x=w430, y=T1 {"Left"=80, "Top"=160} ("Position")) -> (x = y?=w427:cluster{"Left":bool, "Top":bool})
            n293 = Equal?(x=w433, y=T1 {"Left"=80, "Top"=240} ("Position")) -> (x = y?=w436:cluster{"Left":bool, "Top":bool})
            n294 = Unbundle By Name(w426) -> ("Left"=w424:bool, "Top"=w425:bool)
            n295 = Unbundle By Name(w417) -> ("Left"=w419:bool, "Top"=w418:bool)
            n296 = Unbundle By Name(w427) -> ("Left"=w429:bool, "Top"=w428:bool)
            n297 = Unbundle By Name(w436) -> ("Left"=w434:bool, "Top"=w435:bool)
            n298 = And(x=w424, y=w425) -> (x .and. y?=w376:bool)
            n299 = And(x=w419, y=w418) -> (x .and. y?=w377:bool)
            n300 = And(x=w429, y=w428) -> (x .and. y?=w375:bool)
            n301 = And(x=w434, y=w435) -> (x .and. y?=w374:bool)
            n302 = Compound Arithmetic op=AND(w377, w376, w375, w374) -> (w365:bool)
            n303 = property on="Key 7" class="Bool"() -> ("Position"=w410:T1)  [unwired: 2 in, 2 out]
            n304 = property on="Key 3" class="Bool"() -> ("Position"=w413:T1)  [unwired: 2 in, 2 out]
            n305 = property on="Key 11" class="Bool"() -> ("Position"=w403:T1)  [unwired: 2 in, 2 out]
            n306 = property on="Key 15" class="Bool"() -> ("Position"=w400:T1)  [unwired: 2 in, 2 out]
            n307 = Equal?(x=w410, y=T1 {"Left"=160, "Top"=80} ("Position")) -> (x = y?=w407:cluster{"Left":bool, "Top":bool})
            n308 = Equal?(x=w413, y=T1 {"Left"=160, "Top"=0} ("Position")) -> (x = y?=w416:cluster{"Left":bool, "Top":bool})
            n309 = Equal?(x=w403, y=T1 {"Left"=160, "Top"=160} ("Position")) -> (x = y?=w406:cluster{"Left":bool, "Top":bool})
            n310 = Equal?(x=w400, y=T1 {"Left"=160, "Top"=240} ("Position")) -> (x = y?=w397:cluster{"Left":bool, "Top":bool})
            n311 = Unbundle By Name(w407) -> ("Left"=w409:bool, "Top"=w408:bool)
            n312 = Unbundle By Name(w416) -> ("Left"=w414:bool, "Top"=w415:bool)
            n313 = Unbundle By Name(w406) -> ("Left"=w404:bool, "Top"=w405:bool)
            n314 = Unbundle By Name(w397) -> ("Left"=w399:bool, "Top"=w398:bool)
            n315 = And(x=w409, y=w408) -> (x .and. y?=w372:bool)
            n316 = And(x=w414, y=w415) -> (x .and. y?=w373:bool)
            n317 = And(x=w404, y=w405) -> (x .and. y?=w371:bool)
            n318 = And(x=w399, y=w398) -> (x .and. y?=w370:bool)
            n319 = Compound Arithmetic op=AND(w373, w372, w371, w370) -> (w364:bool)
            n320 = property on="Key 8" class="Bool"() -> ("Position"=w388:T1)  [unwired: 2 in, 2 out]
            n321 = property on="Key 4" class="Bool"() -> ("Position"=w385:T1)  [unwired: 2 in, 2 out]
            n322 = property on="Key 12" class="Bool"() -> ("Position"=w395:T1)  [unwired: 2 in, 2 out]
            n323 = Equal?(x=w388, y=T1 {"Left"=240, "Top"=80} ("Position")) -> (x = y?=w391:cluster{"Left":bool, "Top":bool})
            n324 = Equal?(x=w385, y=T1 {"Left"=240, "Top"=0} ("Position")) -> (x = y?=w382:cluster{"Left":bool, "Top":bool})
            n325 = Equal?(x=w395, y=T1 {"Left"=240, "Top"=160} ("Position")) -> (x = y?=w392:cluster{"Left":bool, "Top":bool})
            n326 = Unbundle By Name(w391) -> ("Left"=w389:bool, "Top"=w390:bool)
            n327 = Unbundle By Name(w382) -> ("Left"=w384:bool, "Top"=w383:bool)
            n328 = Unbundle By Name(w392) -> ("Left"=w394:bool, "Top"=w393:bool)
            n329 = And(x=w389, y=w390) -> (x .and. y?=w368:bool)
            n330 = And(x=w384, y=w383) -> (x .and. y?=w369:bool)
            n331 = And(x=w394, y=w393) -> (x .and. y?=w367:bool)
            n332 = Compound Arithmetic op=AND(w369, w368, w367) -> (w363:bool)
            n333 = Compound Arithmetic op=AND(w366, w365, w364, w363) -> (w362:bool)
            n334 = local write "Result"(w362) -> ()
            n335 = property on="Result" class="Bool (strict)"("Val(Sgnl)"=w362) -> ()  [unwired: 2 in, 2 out]
          }
        }
      }
      event "Key 3": Value Change {
        n336 = event-data() -> ()  [unwired: 1 in, 6 out]
        n337 = stacked-sequence {
          frame #0 {
            n338 = local read "Moves Number"() -> (w457:dbl)
            n339 = property on="Key 3" class="Bool"() -> ("Position"=w459:T1)  [unwired: 2 in, 2 out]
            n340 = Increment(x=w457) -> (x+1=w458:dbl)
            n341 = local read "Empty"() -> (w467:cluster{"Left":dbl, "Top":dbl})
            n342 = local read "Empty"() -> (w474:cluster{"Left":dbl, "Top":dbl})
            n343 = local read "Empty"() -> (w486:cluster{"Left":dbl, "Top":dbl})
            n344 = local read "Empty"() -> (w479:cluster{"Left":dbl, "Top":dbl})
            n345 = Add(x=w459, y=T1 {"Left"=80, "Top"=0} ("Position")) -> (x+y=w466:T1)
            n346 = Add(x=w459, y=T1 {"Left"=0, "Top"=80} ("Position")) -> (x+y=w475:T1)
            n347 = Subtract(x=w459, y=T1 {"Left"=80, "Top"=0} ("Position")) -> (x-y=w487:T1)
            n348 = Subtract(x=w459, y=T1 {"Left"=0, "Top"=80} ("Position")) -> (x-y=w478:T1)
            n349 = local write "Moves Number"(w458) -> ()
            n350 = Equal?(x=w466, y=w467) -> (x = y?=w468:cluster{"Left":bool, "Top":bool})
            n351 = Equal?(x=w475, y=w474) -> (x = y?=w473:cluster{"Left":bool, "Top":bool})
            n352 = Equal?(x=w487, y=w486) -> (x = y?=w485:cluster{"Left":bool, "Top":bool})
            n353 = Equal?(x=w478, y=w479) -> (x = y?=w480:cluster{"Left":bool, "Top":bool})
            n354 = Unbundle By Name(w468) -> ("Left"=w470:bool, "Top"=w469:bool)
            n355 = Unbundle By Name(w473) -> ("Left"=w471:bool, "Top"=w472:bool)
            n356 = Unbundle By Name(w485) -> ("Left"=w483:bool, "Top"=w484:bool)
            n357 = Unbundle By Name(w480) -> ("Left"=w482:bool, "Top"=w481:bool)
            n358 = And(x=w470, y=w469) -> (x .and. y?=w461:bool)
            n359 = And(x=w471, y=w472) -> (x .and. y?=w460:bool)
            n360 = And(x=w483, y=w484) -> (x .and. y?=w463:bool)
            n361 = And(x=w482, y=w481) -> (x .and. y?=w462:bool)
            n362 = Compound Arithmetic op=OR(w463, w462, w461, w460) -> (w464:bool)
            n363 = case shown="True" w464 {
              tunnel: w459 -> [_ w489]
              frame False {
              }
              frame True {
                n364 = flat-sequence {
                  tunnel: w489 -> [w490]
                  frame #0 {
                    n365 = local write "Temp Position"(w490) -> ()
                  }
                  frame #1 {
                    n366 = local read "Empty"() -> (w491:cluster{"Left":dbl, "Top":dbl})
                    n367 = property on="Key 3" class="Bool"("Position"=w491) -> ()  [unwired: 2 in, 2 out]
                  }
                  frame #2 {
                    n368 = local read "Temp Position"() -> (w492:cluster{"Left":dbl, "Top":dbl})
                    n369 = local write "Empty"(w492) -> ()
                  }
                }
              }
            }
          }
          frame #1 {
            n370 = property on="Key 5" class="Bool"() -> ("Position"=w581:T1)  [unwired: 2 in, 2 out]
            n371 = property on="Key 1" class="Bool"() -> ("Position"=w584:T1)  [unwired: 2 in, 2 out]
            n372 = property on="Key 9" class="Bool"() -> ("Position"=w574:T1)  [unwired: 2 in, 2 out]
            n373 = property on="Key 13" class="Bool"() -> ("Position"=w571:T1)  [unwired: 2 in, 2 out]
            n374 = Equal?(x=w581, y=T1 {"Left"=0, "Top"=80} ("Position")) -> (x = y?=w578:cluster{"Left":bool, "Top":bool})
            n375 = Equal?(x=w584, y=T1 {"Left"=0, "Top"=0} ("Position")) -> (x = y?=w587:cluster{"Left":bool, "Top":bool})
            n376 = Equal?(x=w574, y=T1 {"Left"=0, "Top"=160} ("Position")) -> (x = y?=w577:cluster{"Left":bool, "Top":bool})
            n377 = Equal?(x=w571, y=T1 {"Left"=0, "Top"=240} ("Position")) -> (x = y?=w568:cluster{"Left":bool, "Top":bool})
            n378 = Unbundle By Name(w578) -> ("Left"=w580:bool, "Top"=w579:bool)
            n379 = Unbundle By Name(w587) -> ("Left"=w585:bool, "Top"=w586:bool)
            n380 = Unbundle By Name(w577) -> ("Left"=w575:bool, "Top"=w576:bool)
            n381 = Unbundle By Name(w568) -> ("Left"=w570:bool, "Top"=w569:bool)
            n382 = And(x=w580, y=w579) -> (x .and. y?=w511:bool)
            n383 = And(x=w585, y=w586) -> (x .and. y?=w512:bool)
            n384 = And(x=w575, y=w576) -> (x .and. y?=w510:bool)
            n385 = And(x=w570, y=w569) -> (x .and. y?=w509:bool)
            n386 = Compound Arithmetic op=AND(w512, w511, w510, w509) -> (w497:bool)
            n387 = property on="Key 6" class="Bool"() -> ("Position"=w554:T1)  [unwired: 2 in, 2 out]
            n388 = property on="Key 2" class="Bool"() -> ("Position"=w551:T1)  [unwired: 2 in, 2 out]
            n389 = property on="Key 10" class="Bool"() -> ("Position"=w561:T1)  [unwired: 2 in, 2 out]
            n390 = property on="Key 14" class="Bool"() -> ("Position"=w564:T1)  [unwired: 2 in, 2 out]
            n391 = Equal?(x=w554, y=T1 {"Left"=80, "Top"=80} ("Position")) -> (x = y?=w557:cluster{"Left":bool, "Top":bool})
            n392 = Equal?(x=w551, y=T1 {"Left"=80, "Top"=0} ("Position")) -> (x = y?=w548:cluster{"Left":bool, "Top":bool})
            n393 = Equal?(x=w561, y=T1 {"Left"=80, "Top"=160} ("Position")) -> (x = y?=w558:cluster{"Left":bool, "Top":bool})
            n394 = Equal?(x=w564, y=T1 {"Left"=80, "Top"=240} ("Position")) -> (x = y?=w567:cluster{"Left":bool, "Top":bool})
            n395 = Unbundle By Name(w557) -> ("Left"=w555:bool, "Top"=w556:bool)
            n396 = Unbundle By Name(w548) -> ("Left"=w550:bool, "Top"=w549:bool)
            n397 = Unbundle By Name(w558) -> ("Left"=w560:bool, "Top"=w559:bool)
            n398 = Unbundle By Name(w567) -> ("Left"=w565:bool, "Top"=w566:bool)
            n399 = And(x=w555, y=w556) -> (x .and. y?=w507:bool)
            n400 = And(x=w550, y=w549) -> (x .and. y?=w508:bool)
            n401 = And(x=w560, y=w559) -> (x .and. y?=w506:bool)
            n402 = And(x=w565, y=w566) -> (x .and. y?=w505:bool)
            n403 = Compound Arithmetic op=AND(w508, w507, w506, w505) -> (w496:bool)
            n404 = property on="Key 7" class="Bool"() -> ("Position"=w541:T1)  [unwired: 2 in, 2 out]
            n405 = property on="Key 3" class="Bool"() -> ("Position"=w544:T1)  [unwired: 2 in, 2 out]
            n406 = property on="Key 11" class="Bool"() -> ("Position"=w534:T1)  [unwired: 2 in, 2 out]
            n407 = property on="Key 15" class="Bool"() -> ("Position"=w531:T1)  [unwired: 2 in, 2 out]
            n408 = Equal?(x=w541, y=T1 {"Left"=160, "Top"=80} ("Position")) -> (x = y?=w538:cluster{"Left":bool, "Top":bool})
            n409 = Equal?(x=w544, y=T1 {"Left"=160, "Top"=0} ("Position")) -> (x = y?=w547:cluster{"Left":bool, "Top":bool})
            n410 = Equal?(x=w534, y=T1 {"Left"=160, "Top"=160} ("Position")) -> (x = y?=w537:cluster{"Left":bool, "Top":bool})
            n411 = Equal?(x=w531, y=T1 {"Left"=160, "Top"=240} ("Position")) -> (x = y?=w528:cluster{"Left":bool, "Top":bool})
            n412 = Unbundle By Name(w538) -> ("Left"=w540:bool, "Top"=w539:bool)
            n413 = Unbundle By Name(w547) -> ("Left"=w545:bool, "Top"=w546:bool)
            n414 = Unbundle By Name(w537) -> ("Left"=w535:bool, "Top"=w536:bool)
            n415 = Unbundle By Name(w528) -> ("Left"=w530:bool, "Top"=w529:bool)
            n416 = And(x=w540, y=w539) -> (x .and. y?=w503:bool)
            n417 = And(x=w545, y=w546) -> (x .and. y?=w504:bool)
            n418 = And(x=w535, y=w536) -> (x .and. y?=w502:bool)
            n419 = And(x=w530, y=w529) -> (x .and. y?=w501:bool)
            n420 = Compound Arithmetic op=AND(w504, w503, w502, w501) -> (w495:bool)
            n421 = property on="Key 8" class="Bool"() -> ("Position"=w519:T1)  [unwired: 2 in, 2 out]
            n422 = property on="Key 4" class="Bool"() -> ("Position"=w516:T1)  [unwired: 2 in, 2 out]
            n423 = property on="Key 12" class="Bool"() -> ("Position"=w526:T1)  [unwired: 2 in, 2 out]
            n424 = Equal?(x=w519, y=T1 {"Left"=240, "Top"=80} ("Position")) -> (x = y?=w522:cluster{"Left":bool, "Top":bool})
            n425 = Equal?(x=w516, y=T1 {"Left"=240, "Top"=0} ("Position")) -> (x = y?=w513:cluster{"Left":bool, "Top":bool})
            n426 = Equal?(x=w526, y=T1 {"Left"=240, "Top"=160} ("Position")) -> (x = y?=w523:cluster{"Left":bool, "Top":bool})
            n427 = Unbundle By Name(w522) -> ("Left"=w520:bool, "Top"=w521:bool)
            n428 = Unbundle By Name(w513) -> ("Left"=w515:bool, "Top"=w514:bool)
            n429 = Unbundle By Name(w523) -> ("Left"=w525:bool, "Top"=w524:bool)
            n430 = And(x=w520, y=w521) -> (x .and. y?=w499:bool)
            n431 = And(x=w515, y=w514) -> (x .and. y?=w500:bool)
            n432 = And(x=w525, y=w524) -> (x .and. y?=w498:bool)
            n433 = Compound Arithmetic op=AND(w500, w499, w498) -> (w494:bool)
            n434 = Compound Arithmetic op=AND(w497, w496, w495, w494) -> (w493:bool)
            n435 = local write "Result"(w493) -> ()
            n436 = property on="Result" class="Bool (strict)"("Val(Sgnl)"=w493) -> ()  [unwired: 2 in, 2 out]
          }
        }
      }
      event "Key 4": Value Change {
        n437 = event-data() -> ()  [unwired: 1 in, 6 out]
        n438 = stacked-sequence {
          frame #0 {
            n439 = local read "Moves Number"() -> (w588:dbl)
            n440 = property on="Key 4" class="Bool"() -> ("Position"=w590:T1)  [unwired: 2 in, 2 out]
            n441 = local read "Empty"() -> (w598:cluster{"Left":dbl, "Top":dbl})
            n442 = local read "Empty"() -> (w605:cluster{"Left":dbl, "Top":dbl})
            n443 = Increment(x=w588) -> (x+1=w589:dbl)
            n444 = local read "Empty"() -> (w617:cluster{"Left":dbl, "Top":dbl})
            n445 = local read "Empty"() -> (w610:cluster{"Left":dbl, "Top":dbl})
            n446 = Add(x=w590, y=T1 {"Left"=80, "Top"=0} ("Position")) -> (x+y=w597:T1)
            n447 = Add(x=w590, y=T1 {"Left"=0, "Top"=80} ("Position")) -> (x+y=w606:T1)
            n448 = Subtract(x=w590, y=T1 {"Left"=80, "Top"=0} ("Position")) -> (x-y=w618:T1)
            n449 = Subtract(x=w590, y=T1 {"Left"=0, "Top"=80} ("Position")) -> (x-y=w609:T1)
            n450 = local write "Moves Number"(w589) -> ()
            n451 = Equal?(x=w597, y=w598) -> (x = y?=w599:cluster{"Left":bool, "Top":bool})
            n452 = Equal?(x=w606, y=w605) -> (x = y?=w604:cluster{"Left":bool, "Top":bool})
            n453 = Equal?(x=w618, y=w617) -> (x = y?=w616:cluster{"Left":bool, "Top":bool})
            n454 = Equal?(x=w609, y=w610) -> (x = y?=w611:cluster{"Left":bool, "Top":bool})
            n455 = Unbundle By Name(w599) -> ("Left"=w601:bool, "Top"=w600:bool)
            n456 = Unbundle By Name(w604) -> ("Left"=w602:bool, "Top"=w603:bool)
            n457 = Unbundle By Name(w616) -> ("Left"=w614:bool, "Top"=w615:bool)
            n458 = Unbundle By Name(w611) -> ("Left"=w613:bool, "Top"=w612:bool)
            n459 = And(x=w601, y=w600) -> (x .and. y?=w592:bool)
            n460 = And(x=w602, y=w603) -> (x .and. y?=w591:bool)
            n461 = And(x=w614, y=w615) -> (x .and. y?=w594:bool)
            n462 = And(x=w613, y=w612) -> (x .and. y?=w593:bool)
            n463 = Compound Arithmetic op=OR(w594, w593, w592, w591) -> (w595:bool)
            n464 = case shown="True" w595 {
              tunnel: w590 -> [_ w620]
              frame False {
              }
              frame True {
                n465 = flat-sequence {
                  tunnel: w620 -> [w621]
                  frame #0 {
                    n466 = local write "Temp Position"(w621) -> ()
                  }
                  frame #1 {
                    n467 = local read "Empty"() -> (w622:cluster{"Left":dbl, "Top":dbl})
                    n468 = property on="Key 4" class="Bool"("Position"=w622) -> ()  [unwired: 2 in, 2 out]
                  }
                  frame #2 {
                    n469 = local read "Temp Position"() -> (w623:cluster{"Left":dbl, "Top":dbl})
                    n470 = local write "Empty"(w623) -> ()
                  }
                }
              }
            }
          }
          frame #1 {
            n471 = property on="Key 5" class="Bool"() -> ("Position"=w712:T1)  [unwired: 2 in, 2 out]
            n472 = property on="Key 1" class="Bool"() -> ("Position"=w715:T1)  [unwired: 2 in, 2 out]
            n473 = property on="Key 9" class="Bool"() -> ("Position"=w705:T1)  [unwired: 2 in, 2 out]
            n474 = property on="Key 13" class="Bool"() -> ("Position"=w702:T1)  [unwired: 2 in, 2 out]
            n475 = Equal?(x=w712, y=T1 {"Left"=0, "Top"=80} ("Position")) -> (x = y?=w709:cluster{"Left":bool, "Top":bool})
            n476 = Equal?(x=w715, y=T1 {"Left"=0, "Top"=0} ("Position")) -> (x = y?=w718:cluster{"Left":bool, "Top":bool})
            n477 = Equal?(x=w705, y=T1 {"Left"=0, "Top"=160} ("Position")) -> (x = y?=w708:cluster{"Left":bool, "Top":bool})
            n478 = Equal?(x=w702, y=T1 {"Left"=0, "Top"=240} ("Position")) -> (x = y?=w699:cluster{"Left":bool, "Top":bool})
            n479 = Unbundle By Name(w709) -> ("Left"=w711:bool, "Top"=w710:bool)
            n480 = Unbundle By Name(w718) -> ("Left"=w716:bool, "Top"=w717:bool)
            n481 = Unbundle By Name(w708) -> ("Left"=w706:bool, "Top"=w707:bool)
            n482 = Unbundle By Name(w699) -> ("Left"=w701:bool, "Top"=w700:bool)
            n483 = And(x=w711, y=w710) -> (x .and. y?=w642:bool)
            n484 = And(x=w716, y=w717) -> (x .and. y?=w643:bool)
            n485 = And(x=w706, y=w707) -> (x .and. y?=w641:bool)
            n486 = And(x=w701, y=w700) -> (x .and. y?=w640:bool)
            n487 = Compound Arithmetic op=AND(w643, w642, w641, w640) -> (w628:bool)
            n488 = property on="Key 6" class="Bool"() -> ("Position"=w685:T1)  [unwired: 2 in, 2 out]
            n489 = property on="Key 2" class="Bool"() -> ("Position"=w682:T1)  [unwired: 2 in, 2 out]
            n490 = property on="Key 10" class="Bool"() -> ("Position"=w692:T1)  [unwired: 2 in, 2 out]
            n491 = property on="Key 14" class="Bool"() -> ("Position"=w695:T1)  [unwired: 2 in, 2 out]
            n492 = Equal?(x=w685, y=T1 {"Left"=80, "Top"=80} ("Position")) -> (x = y?=w688:cluster{"Left":bool, "Top":bool})
            n493 = Equal?(x=w682, y=T1 {"Left"=80, "Top"=0} ("Position")) -> (x = y?=w679:cluster{"Left":bool, "Top":bool})
            n494 = Equal?(x=w692, y=T1 {"Left"=80, "Top"=160} ("Position")) -> (x = y?=w689:cluster{"Left":bool, "Top":bool})
            n495 = Equal?(x=w695, y=T1 {"Left"=80, "Top"=240} ("Position")) -> (x = y?=w698:cluster{"Left":bool, "Top":bool})
            n496 = Unbundle By Name(w688) -> ("Left"=w686:bool, "Top"=w687:bool)
            n497 = Unbundle By Name(w679) -> ("Left"=w681:bool, "Top"=w680:bool)
            n498 = Unbundle By Name(w689) -> ("Left"=w691:bool, "Top"=w690:bool)
            n499 = Unbundle By Name(w698) -> ("Left"=w696:bool, "Top"=w697:bool)
            n500 = And(x=w686, y=w687) -> (x .and. y?=w638:bool)
            n501 = And(x=w681, y=w680) -> (x .and. y?=w639:bool)
            n502 = And(x=w691, y=w690) -> (x .and. y?=w637:bool)
            n503 = And(x=w696, y=w697) -> (x .and. y?=w636:bool)
            n504 = Compound Arithmetic op=AND(w639, w638, w637, w636) -> (w627:bool)
            n505 = property on="Key 7" class="Bool"() -> ("Position"=w672:T1)  [unwired: 2 in, 2 out]
            n506 = property on="Key 3" class="Bool"() -> ("Position"=w675:T1)  [unwired: 2 in, 2 out]
            n507 = property on="Key 11" class="Bool"() -> ("Position"=w665:T1)  [unwired: 2 in, 2 out]
            n508 = property on="Key 15" class="Bool"() -> ("Position"=w662:T1)  [unwired: 2 in, 2 out]
            n509 = Equal?(x=w672, y=T1 {"Left"=160, "Top"=80} ("Position")) -> (x = y?=w669:cluster{"Left":bool, "Top":bool})
            n510 = Equal?(x=w675, y=T1 {"Left"=160, "Top"=0} ("Position")) -> (x = y?=w678:cluster{"Left":bool, "Top":bool})
            n511 = Equal?(x=w665, y=T1 {"Left"=160, "Top"=160} ("Position")) -> (x = y?=w668:cluster{"Left":bool, "Top":bool})
            n512 = Equal?(x=w662, y=T1 {"Left"=160, "Top"=240} ("Position")) -> (x = y?=w659:cluster{"Left":bool, "Top":bool})
            n513 = Unbundle By Name(w669) -> ("Left"=w671:bool, "Top"=w670:bool)
            n514 = Unbundle By Name(w678) -> ("Left"=w676:bool, "Top"=w677:bool)
            n515 = Unbundle By Name(w668) -> ("Left"=w666:bool, "Top"=w667:bool)
            n516 = Unbundle By Name(w659) -> ("Left"=w661:bool, "Top"=w660:bool)
            n517 = And(x=w671, y=w670) -> (x .and. y?=w634:bool)
            n518 = And(x=w676, y=w677) -> (x .and. y?=w635:bool)
            n519 = And(x=w666, y=w667) -> (x .and. y?=w633:bool)
            n520 = And(x=w661, y=w660) -> (x .and. y?=w632:bool)
            n521 = Compound Arithmetic op=AND(w635, w634, w633, w632) -> (w626:bool)
            n522 = property on="Key 8" class="Bool"() -> ("Position"=w650:T1)  [unwired: 2 in, 2 out]
            n523 = property on="Key 4" class="Bool"() -> ("Position"=w647:T1)  [unwired: 2 in, 2 out]
            n524 = property on="Key 12" class="Bool"() -> ("Position"=w657:T1)  [unwired: 2 in, 2 out]
            n525 = Equal?(x=w650, y=T1 {"Left"=240, "Top"=80} ("Position")) -> (x = y?=w653:cluster{"Left":bool, "Top":bool})
            n526 = Equal?(x=w647, y=T1 {"Left"=240, "Top"=0} ("Position")) -> (x = y?=w644:cluster{"Left":bool, "Top":bool})
            n527 = Equal?(x=w657, y=T1 {"Left"=240, "Top"=160} ("Position")) -> (x = y?=w654:cluster{"Left":bool, "Top":bool})
            n528 = Unbundle By Name(w653) -> ("Left"=w651:bool, "Top"=w652:bool)
            n529 = Unbundle By Name(w644) -> ("Left"=w646:bool, "Top"=w645:bool)
            n530 = Unbundle By Name(w654) -> ("Left"=w656:bool, "Top"=w655:bool)
            n531 = And(x=w651, y=w652) -> (x .and. y?=w630:bool)
            n532 = And(x=w646, y=w645) -> (x .and. y?=w631:bool)
            n533 = And(x=w656, y=w655) -> (x .and. y?=w629:bool)
            n534 = Compound Arithmetic op=AND(w631, w630, w629) -> (w625:bool)
            n535 = Compound Arithmetic op=AND(w628, w627, w626, w625) -> (w624:bool)
            n536 = local write "Result"(w624) -> ()
            n537 = property on="Result" class="Bool (strict)"("Val(Sgnl)"=w624) -> ()  [unwired: 2 in, 2 out]
          }
        }
      }
      event "Key 5": Value Change {
        n538 = event-data() -> ()  [unwired: 1 in, 6 out]
        n539 = stacked-sequence {
          frame #0 {
            n540 = local read "Moves Number"() -> (w719:dbl)
            n541 = property on="Key 5" class="Bool"() -> ("Position"=w721:T1)  [unwired: 2 in, 2 out]
            n542 = Increment(x=w719) -> (x+1=w720:dbl)
            n543 = local read "Empty"() -> (w729:cluster{"Left":dbl, "Top":dbl})
            n544 = local read "Empty"() -> (w736:cluster{"Left":dbl, "Top":dbl})
            n545 = local read "Empty"() -> (w748:cluster{"Left":dbl, "Top":dbl})
            n546 = local read "Empty"() -> (w741:cluster{"Left":dbl, "Top":dbl})
            n547 = Add(x=w721, y=T1 {"Left"=80, "Top"=0} ("Position")) -> (x+y=w728:T1)
            n548 = Add(x=w721, y=T1 {"Left"=0, "Top"=80} ("Position")) -> (x+y=w737:T1)
            n549 = Subtract(x=w721, y=T1 {"Left"=80, "Top"=0} ("Position")) -> (x-y=w749:T1)
            n550 = Subtract(x=w721, y=T1 {"Left"=0, "Top"=80} ("Position")) -> (x-y=w740:T1)
            n551 = local write "Moves Number"(w720) -> ()
            n552 = Equal?(x=w728, y=w729) -> (x = y?=w730:cluster{"Left":bool, "Top":bool})
            n553 = Equal?(x=w737, y=w736) -> (x = y?=w735:cluster{"Left":bool, "Top":bool})
            n554 = Equal?(x=w749, y=w748) -> (x = y?=w747:cluster{"Left":bool, "Top":bool})
            n555 = Equal?(x=w740, y=w741) -> (x = y?=w742:cluster{"Left":bool, "Top":bool})
            n556 = Unbundle By Name(w730) -> ("Left"=w732:bool, "Top"=w731:bool)
            n557 = Unbundle By Name(w735) -> ("Left"=w733:bool, "Top"=w734:bool)
            n558 = Unbundle By Name(w747) -> ("Left"=w745:bool, "Top"=w746:bool)
            n559 = Unbundle By Name(w742) -> ("Left"=w744:bool, "Top"=w743:bool)
            n560 = And(x=w732, y=w731) -> (x .and. y?=w723:bool)
            n561 = And(x=w733, y=w734) -> (x .and. y?=w722:bool)
            n562 = And(x=w745, y=w746) -> (x .and. y?=w725:bool)
            n563 = And(x=w744, y=w743) -> (x .and. y?=w724:bool)
            n564 = Compound Arithmetic op=OR(w725, w724, w723, w722) -> (w726:bool)
            n565 = case shown="True" w726 {
              tunnel: w721 -> [_ w751]
              frame False {
              }
              frame True {
                n566 = flat-sequence {
                  tunnel: w751 -> [w752]
                  frame #0 {
                    n567 = local write "Temp Position"(w752) -> ()
                  }
                  frame #1 {
                    n568 = local read "Empty"() -> (w753:cluster{"Left":dbl, "Top":dbl})
                    n569 = property on="Key 5" class="Bool"("Position"=w753) -> ()  [unwired: 2 in, 2 out]
                  }
                  frame #2 {
                    n570 = local read "Temp Position"() -> (w754:cluster{"Left":dbl, "Top":dbl})
                    n571 = local write "Empty"(w754) -> ()
                  }
                }
              }
            }
          }
          frame #1 {
            n572 = property on="Key 5" class="Bool"() -> ("Position"=w843:T1)  [unwired: 2 in, 2 out]
            n573 = property on="Key 1" class="Bool"() -> ("Position"=w846:T1)  [unwired: 2 in, 2 out]
            n574 = property on="Key 9" class="Bool"() -> ("Position"=w836:T1)  [unwired: 2 in, 2 out]
            n575 = property on="Key 13" class="Bool"() -> ("Position"=w833:T1)  [unwired: 2 in, 2 out]
            n576 = Equal?(x=w843, y=T1 {"Left"=0, "Top"=80} ("Position")) -> (x = y?=w840:cluster{"Left":bool, "Top":bool})
            n577 = Equal?(x=w846, y=T1 {"Left"=0, "Top"=0} ("Position")) -> (x = y?=w849:cluster{"Left":bool, "Top":bool})
            n578 = Equal?(x=w836, y=T1 {"Left"=0, "Top"=160} ("Position")) -> (x = y?=w839:cluster{"Left":bool, "Top":bool})
            n579 = Equal?(x=w833, y=T1 {"Left"=0, "Top"=240} ("Position")) -> (x = y?=w830:cluster{"Left":bool, "Top":bool})
            n580 = Unbundle By Name(w840) -> ("Left"=w842:bool, "Top"=w841:bool)
            n581 = Unbundle By Name(w849) -> ("Left"=w847:bool, "Top"=w848:bool)
            n582 = Unbundle By Name(w839) -> ("Left"=w837:bool, "Top"=w838:bool)
            n583 = Unbundle By Name(w830) -> ("Left"=w832:bool, "Top"=w831:bool)
            n584 = And(x=w842, y=w841) -> (x .and. y?=w773:bool)
            n585 = And(x=w847, y=w848) -> (x .and. y?=w774:bool)
            n586 = And(x=w837, y=w838) -> (x .and. y?=w772:bool)
            n587 = And(x=w832, y=w831) -> (x .and. y?=w771:bool)
            n588 = Compound Arithmetic op=AND(w774, w773, w772, w771) -> (w759:bool)
            n589 = property on="Key 6" class="Bool"() -> ("Position"=w816:T1)  [unwired: 2 in, 2 out]
            n590 = property on="Key 2" class="Bool"() -> ("Position"=w813:T1)  [unwired: 2 in, 2 out]
            n591 = property on="Key 10" class="Bool"() -> ("Position"=w823:T1)  [unwired: 2 in, 2 out]
            n592 = property on="Key 14" class="Bool"() -> ("Position"=w826:T1)  [unwired: 2 in, 2 out]
            n593 = Equal?(x=w816, y=T1 {"Left"=80, "Top"=80} ("Position")) -> (x = y?=w819:cluster{"Left":bool, "Top":bool})
            n594 = Equal?(x=w813, y=T1 {"Left"=80, "Top"=0} ("Position")) -> (x = y?=w810:cluster{"Left":bool, "Top":bool})
            n595 = Equal?(x=w823, y=T1 {"Left"=80, "Top"=160} ("Position")) -> (x = y?=w820:cluster{"Left":bool, "Top":bool})
            n596 = Equal?(x=w826, y=T1 {"Left"=80, "Top"=240} ("Position")) -> (x = y?=w829:cluster{"Left":bool, "Top":bool})
            n597 = Unbundle By Name(w819) -> ("Left"=w817:bool, "Top"=w818:bool)
            n598 = Unbundle By Name(w810) -> ("Left"=w812:bool, "Top"=w811:bool)
            n599 = Unbundle By Name(w820) -> ("Left"=w822:bool, "Top"=w821:bool)
            n600 = Unbundle By Name(w829) -> ("Left"=w827:bool, "Top"=w828:bool)
            n601 = And(x=w817, y=w818) -> (x .and. y?=w769:bool)
            n602 = And(x=w812, y=w811) -> (x .and. y?=w770:bool)
            n603 = And(x=w822, y=w821) -> (x .and. y?=w768:bool)
            n604 = And(x=w827, y=w828) -> (x .and. y?=w767:bool)
            n605 = Compound Arithmetic op=AND(w770, w769, w768, w767) -> (w758:bool)
            n606 = property on="Key 7" class="Bool"() -> ("Position"=w803:T1)  [unwired: 2 in, 2 out]
            n607 = property on="Key 3" class="Bool"() -> ("Position"=w806:T1)  [unwired: 2 in, 2 out]
            n608 = property on="Key 11" class="Bool"() -> ("Position"=w796:T1)  [unwired: 2 in, 2 out]
            n609 = property on="Key 15" class="Bool"() -> ("Position"=w793:T1)  [unwired: 2 in, 2 out]
            n610 = Equal?(x=w803, y=T1 {"Left"=160, "Top"=80} ("Position")) -> (x = y?=w800:cluster{"Left":bool, "Top":bool})
            n611 = Equal?(x=w806, y=T1 {"Left"=160, "Top"=0} ("Position")) -> (x = y?=w809:cluster{"Left":bool, "Top":bool})
            n612 = Equal?(x=w796, y=T1 {"Left"=160, "Top"=160} ("Position")) -> (x = y?=w799:cluster{"Left":bool, "Top":bool})
            n613 = Equal?(x=w793, y=T1 {"Left"=160, "Top"=240} ("Position")) -> (x = y?=w790:cluster{"Left":bool, "Top":bool})
            n614 = Unbundle By Name(w800) -> ("Left"=w802:bool, "Top"=w801:bool)
            n615 = Unbundle By Name(w809) -> ("Left"=w807:bool, "Top"=w808:bool)
            n616 = Unbundle By Name(w799) -> ("Left"=w797:bool, "Top"=w798:bool)
            n617 = Unbundle By Name(w790) -> ("Left"=w792:bool, "Top"=w791:bool)
            n618 = And(x=w802, y=w801) -> (x .and. y?=w765:bool)
            n619 = And(x=w807, y=w808) -> (x .and. y?=w766:bool)
            n620 = And(x=w797, y=w798) -> (x .and. y?=w764:bool)
            n621 = And(x=w792, y=w791) -> (x .and. y?=w763:bool)
            n622 = Compound Arithmetic op=AND(w766, w765, w764, w763) -> (w757:bool)
            n623 = property on="Key 8" class="Bool"() -> ("Position"=w781:T1)  [unwired: 2 in, 2 out]
            n624 = property on="Key 4" class="Bool"() -> ("Position"=w778:T1)  [unwired: 2 in, 2 out]
            n625 = property on="Key 12" class="Bool"() -> ("Position"=w788:T1)  [unwired: 2 in, 2 out]
            n626 = Equal?(x=w781, y=T1 {"Left"=240, "Top"=80} ("Position")) -> (x = y?=w784:cluster{"Left":bool, "Top":bool})
            n627 = Equal?(x=w778, y=T1 {"Left"=240, "Top"=0} ("Position")) -> (x = y?=w775:cluster{"Left":bool, "Top":bool})
            n628 = Equal?(x=w788, y=T1 {"Left"=240, "Top"=160} ("Position")) -> (x = y?=w785:cluster{"Left":bool, "Top":bool})
            n629 = Unbundle By Name(w784) -> ("Left"=w782:bool, "Top"=w783:bool)
            n630 = Unbundle By Name(w775) -> ("Left"=w777:bool, "Top"=w776:bool)
            n631 = Unbundle By Name(w785) -> ("Left"=w787:bool, "Top"=w786:bool)
            n632 = And(x=w782, y=w783) -> (x .and. y?=w761:bool)
            n633 = And(x=w777, y=w776) -> (x .and. y?=w762:bool)
            n634 = And(x=w787, y=w786) -> (x .and. y?=w760:bool)
            n635 = Compound Arithmetic op=AND(w762, w761, w760) -> (w756:bool)
            n636 = Compound Arithmetic op=AND(w759, w758, w757, w756) -> (w755:bool)
            n637 = local write "Result"(w755) -> ()
            n638 = property on="Result" class="Bool (strict)"("Val(Sgnl)"=w755) -> ()  [unwired: 2 in, 2 out]
          }
        }
      }
      event "Key 6": Value Change {
        n639 = event-data() -> ()  [unwired: 1 in, 6 out]
        n640 = stacked-sequence {
          frame #0 {
            n641 = property on="Key 6" class="Bool"() -> ("Position"=w852:T1)  [unwired: 2 in, 2 out]
            n642 = local read "Moves Number"() -> (w850:dbl)
            n643 = local read "Empty"() -> (w860:cluster{"Left":dbl, "Top":dbl})
            n644 = local read "Empty"() -> (w867:cluster{"Left":dbl, "Top":dbl})
            n645 = local read "Empty"() -> (w879:cluster{"Left":dbl, "Top":dbl})
            n646 = local read "Empty"() -> (w872:cluster{"Left":dbl, "Top":dbl})
            n647 = Increment(x=w850) -> (x+1=w851:dbl)
            n648 = Add(x=w852, y=T1 {"Left"=80, "Top"=0} ("Position")) -> (x+y=w859:T1)
            n649 = Add(x=w852, y=T1 {"Left"=0, "Top"=80} ("Position")) -> (x+y=w868:T1)
            n650 = Subtract(x=w852, y=T1 {"Left"=80, "Top"=0} ("Position")) -> (x-y=w880:T1)
            n651 = Subtract(x=w852, y=T1 {"Left"=0, "Top"=80} ("Position")) -> (x-y=w871:T1)
            n652 = local write "Moves Number"(w851) -> ()
            n653 = Equal?(x=w859, y=w860) -> (x = y?=w861:cluster{"Left":bool, "Top":bool})
            n654 = Equal?(x=w868, y=w867) -> (x = y?=w866:cluster{"Left":bool, "Top":bool})
            n655 = Equal?(x=w880, y=w879) -> (x = y?=w878:cluster{"Left":bool, "Top":bool})
            n656 = Equal?(x=w871, y=w872) -> (x = y?=w873:cluster{"Left":bool, "Top":bool})
            n657 = Unbundle By Name(w861) -> ("Left"=w863:bool, "Top"=w862:bool)
            n658 = Unbundle By Name(w866) -> ("Left"=w864:bool, "Top"=w865:bool)
            n659 = Unbundle By Name(w878) -> ("Left"=w876:bool, "Top"=w877:bool)
            n660 = Unbundle By Name(w873) -> ("Left"=w875:bool, "Top"=w874:bool)
            n661 = And(x=w863, y=w862) -> (x .and. y?=w854:bool)
            n662 = And(x=w864, y=w865) -> (x .and. y?=w853:bool)
            n663 = And(x=w876, y=w877) -> (x .and. y?=w856:bool)
            n664 = And(x=w875, y=w874) -> (x .and. y?=w855:bool)
            n665 = Compound Arithmetic op=OR(w856, w855, w854, w853) -> (w857:bool)
            n666 = case shown="True" w857 {
              tunnel: w852 -> [_ w882]
              frame False {
              }
              frame True {
                n667 = flat-sequence {
                  tunnel: w882 -> [w883]
                  frame #0 {
                    n668 = local write "Temp Position"(w883) -> ()
                  }
                  frame #1 {
                    n669 = local read "Empty"() -> (w884:cluster{"Left":dbl, "Top":dbl})
                    n670 = property on="Key 6" class="Bool"("Position"=w884) -> ()  [unwired: 2 in, 2 out]
                  }
                  frame #2 {
                    n671 = local read "Temp Position"() -> (w885:cluster{"Left":dbl, "Top":dbl})
                    n672 = local write "Empty"(w885) -> ()
                  }
                }
              }
            }
          }
          frame #1 {
            n673 = property on="Key 5" class="Bool"() -> ("Position"=w974:T1)  [unwired: 2 in, 2 out]
            n674 = property on="Key 1" class="Bool"() -> ("Position"=w977:T1)  [unwired: 2 in, 2 out]
            n675 = property on="Key 9" class="Bool"() -> ("Position"=w967:T1)  [unwired: 2 in, 2 out]
            n676 = property on="Key 13" class="Bool"() -> ("Position"=w964:T1)  [unwired: 2 in, 2 out]
            n677 = Equal?(x=w974, y=T1 {"Left"=0, "Top"=80} ("Position")) -> (x = y?=w971:cluster{"Left":bool, "Top":bool})
            n678 = Equal?(x=w977, y=T1 {"Left"=0, "Top"=0} ("Position")) -> (x = y?=w980:cluster{"Left":bool, "Top":bool})
            n679 = Equal?(x=w967, y=T1 {"Left"=0, "Top"=160} ("Position")) -> (x = y?=w970:cluster{"Left":bool, "Top":bool})
            n680 = Equal?(x=w964, y=T1 {"Left"=0, "Top"=240} ("Position")) -> (x = y?=w961:cluster{"Left":bool, "Top":bool})
            n681 = Unbundle By Name(w971) -> ("Left"=w973:bool, "Top"=w972:bool)
            n682 = Unbundle By Name(w980) -> ("Left"=w978:bool, "Top"=w979:bool)
            n683 = Unbundle By Name(w970) -> ("Left"=w968:bool, "Top"=w969:bool)
            n684 = Unbundle By Name(w961) -> ("Left"=w963:bool, "Top"=w962:bool)
            n685 = And(x=w973, y=w972) -> (x .and. y?=w904:bool)
            n686 = And(x=w978, y=w979) -> (x .and. y?=w905:bool)
            n687 = And(x=w968, y=w969) -> (x .and. y?=w903:bool)
            n688 = And(x=w963, y=w962) -> (x .and. y?=w902:bool)
            n689 = Compound Arithmetic op=AND(w905, w904, w903, w902) -> (w890:bool)
            n690 = property on="Key 6" class="Bool"() -> ("Position"=w947:T1)  [unwired: 2 in, 2 out]
            n691 = property on="Key 2" class="Bool"() -> ("Position"=w944:T1)  [unwired: 2 in, 2 out]
            n692 = property on="Key 10" class="Bool"() -> ("Position"=w954:T1)  [unwired: 2 in, 2 out]
            n693 = property on="Key 14" class="Bool"() -> ("Position"=w957:T1)  [unwired: 2 in, 2 out]
            n694 = Equal?(x=w947, y=T1 {"Left"=80, "Top"=80} ("Position")) -> (x = y?=w950:cluster{"Left":bool, "Top":bool})
            n695 = Equal?(x=w944, y=T1 {"Left"=80, "Top"=0} ("Position")) -> (x = y?=w941:cluster{"Left":bool, "Top":bool})
            n696 = Equal?(x=w954, y=T1 {"Left"=80, "Top"=160} ("Position")) -> (x = y?=w951:cluster{"Left":bool, "Top":bool})
            n697 = Equal?(x=w957, y=T1 {"Left"=80, "Top"=240} ("Position")) -> (x = y?=w960:cluster{"Left":bool, "Top":bool})
            n698 = Unbundle By Name(w950) -> ("Left"=w948:bool, "Top"=w949:bool)
            n699 = Unbundle By Name(w941) -> ("Left"=w943:bool, "Top"=w942:bool)
            n700 = Unbundle By Name(w951) -> ("Left"=w953:bool, "Top"=w952:bool)
            n701 = Unbundle By Name(w960) -> ("Left"=w958:bool, "Top"=w959:bool)
            n702 = And(x=w948, y=w949) -> (x .and. y?=w900:bool)
            n703 = And(x=w943, y=w942) -> (x .and. y?=w901:bool)
            n704 = And(x=w953, y=w952) -> (x .and. y?=w899:bool)
            n705 = And(x=w958, y=w959) -> (x .and. y?=w898:bool)
            n706 = Compound Arithmetic op=AND(w901, w900, w899, w898) -> (w889:bool)
            n707 = property on="Key 7" class="Bool"() -> ("Position"=w934:T1)  [unwired: 2 in, 2 out]
            n708 = property on="Key 3" class="Bool"() -> ("Position"=w937:T1)  [unwired: 2 in, 2 out]
            n709 = property on="Key 11" class="Bool"() -> ("Position"=w927:T1)  [unwired: 2 in, 2 out]
            n710 = property on="Key 15" class="Bool"() -> ("Position"=w924:T1)  [unwired: 2 in, 2 out]
            n711 = Equal?(x=w934, y=T1 {"Left"=160, "Top"=80} ("Position")) -> (x = y?=w931:cluster{"Left":bool, "Top":bool})
            n712 = Equal?(x=w937, y=T1 {"Left"=160, "Top"=0} ("Position")) -> (x = y?=w940:cluster{"Left":bool, "Top":bool})
            n713 = Equal?(x=w927, y=T1 {"Left"=160, "Top"=160} ("Position")) -> (x = y?=w930:cluster{"Left":bool, "Top":bool})
            n714 = Equal?(x=w924, y=T1 {"Left"=160, "Top"=240} ("Position")) -> (x = y?=w921:cluster{"Left":bool, "Top":bool})
            n715 = Unbundle By Name(w931) -> ("Left"=w933:bool, "Top"=w932:bool)
            n716 = Unbundle By Name(w940) -> ("Left"=w938:bool, "Top"=w939:bool)
            n717 = Unbundle By Name(w930) -> ("Left"=w928:bool, "Top"=w929:bool)
            n718 = Unbundle By Name(w921) -> ("Left"=w923:bool, "Top"=w922:bool)
            n719 = And(x=w933, y=w932) -> (x .and. y?=w896:bool)
            n720 = And(x=w938, y=w939) -> (x .and. y?=w897:bool)
            n721 = And(x=w928, y=w929) -> (x .and. y?=w895:bool)
            n722 = And(x=w923, y=w922) -> (x .and. y?=w894:bool)
            n723 = Compound Arithmetic op=AND(w897, w896, w895, w894) -> (w888:bool)
            n724 = property on="Key 8" class="Bool"() -> ("Position"=w912:T1)  [unwired: 2 in, 2 out]
            n725 = property on="Key 4" class="Bool"() -> ("Position"=w909:T1)  [unwired: 2 in, 2 out]
            n726 = property on="Key 12" class="Bool"() -> ("Position"=w919:T1)  [unwired: 2 in, 2 out]
            n727 = Equal?(x=w912, y=T1 {"Left"=240, "Top"=80} ("Position")) -> (x = y?=w915:cluster{"Left":bool, "Top":bool})
            n728 = Equal?(x=w909, y=T1 {"Left"=240, "Top"=0} ("Position")) -> (x = y?=w906:cluster{"Left":bool, "Top":bool})
            n729 = Equal?(x=w919, y=T1 {"Left"=240, "Top"=160} ("Position")) -> (x = y?=w916:cluster{"Left":bool, "Top":bool})
            n730 = Unbundle By Name(w915) -> ("Left"=w913:bool, "Top"=w914:bool)
            n731 = Unbundle By Name(w906) -> ("Left"=w908:bool, "Top"=w907:bool)
            n732 = Unbundle By Name(w916) -> ("Left"=w918:bool, "Top"=w917:bool)
            n733 = And(x=w913, y=w914) -> (x .and. y?=w892:bool)
            n734 = And(x=w908, y=w907) -> (x .and. y?=w893:bool)
            n735 = And(x=w918, y=w917) -> (x .and. y?=w891:bool)
            n736 = Compound Arithmetic op=AND(w893, w892, w891) -> (w887:bool)
            n737 = Compound Arithmetic op=AND(w890, w889, w888, w887) -> (w886:bool)
            n738 = local write "Result"(w886) -> ()
            n739 = property on="Result" class="Bool (strict)"("Val(Sgnl)"=w886) -> ()  [unwired: 2 in, 2 out]
          }
        }
      }
      event "Key 7": Value Change {
        n740 = event-data() -> ()  [unwired: 1 in, 6 out]
        n741 = stacked-sequence {
          frame #0 {
            n742 = local read "Moves Number"() -> (w981:dbl)
            n743 = property on="Key 7" class="Bool"() -> ("Position"=w983:T1)  [unwired: 2 in, 2 out]
            n744 = Increment(x=w981) -> (x+1=w982:dbl)
            n745 = local read "Empty"() -> (w991:cluster{"Left":dbl, "Top":dbl})
            n746 = local read "Empty"() -> (w998:cluster{"Left":dbl, "Top":dbl})
            n747 = local read "Empty"() -> (w1010:cluster{"Left":dbl, "Top":dbl})
            n748 = local read "Empty"() -> (w1003:cluster{"Left":dbl, "Top":dbl})
            n749 = Add(x=w983, y=T1 {"Left"=80, "Top"=0} ("Position")) -> (x+y=w990:T1)
            n750 = Add(x=w983, y=T1 {"Left"=0, "Top"=80} ("Position")) -> (x+y=w999:T1)
            n751 = Subtract(x=w983, y=T1 {"Left"=80, "Top"=0} ("Position")) -> (x-y=w1011:T1)
            n752 = Subtract(x=w983, y=T1 {"Left"=0, "Top"=80} ("Position")) -> (x-y=w1002:T1)
            n753 = local write "Moves Number"(w982) -> ()
            n754 = Equal?(x=w990, y=w991) -> (x = y?=w992:cluster{"Left":bool, "Top":bool})
            n755 = Equal?(x=w999, y=w998) -> (x = y?=w997:cluster{"Left":bool, "Top":bool})
            n756 = Equal?(x=w1011, y=w1010) -> (x = y?=w1009:cluster{"Left":bool, "Top":bool})
            n757 = Equal?(x=w1002, y=w1003) -> (x = y?=w1004:cluster{"Left":bool, "Top":bool})
            n758 = Unbundle By Name(w992) -> ("Left"=w994:bool, "Top"=w993:bool)
            n759 = Unbundle By Name(w997) -> ("Left"=w995:bool, "Top"=w996:bool)
            n760 = Unbundle By Name(w1009) -> ("Left"=w1007:bool, "Top"=w1008:bool)
            n761 = Unbundle By Name(w1004) -> ("Left"=w1006:bool, "Top"=w1005:bool)
            n762 = And(x=w994, y=w993) -> (x .and. y?=w985:bool)
            n763 = And(x=w995, y=w996) -> (x .and. y?=w984:bool)
            n764 = And(x=w1007, y=w1008) -> (x .and. y?=w987:bool)
            n765 = And(x=w1006, y=w1005) -> (x .and. y?=w986:bool)
            n766 = Compound Arithmetic op=OR(w987, w986, w985, w984) -> (w988:bool)
            n767 = case shown="True" w988 {
              tunnel: w983 -> [_ w1013]
              frame False {
              }
              frame True {
                n768 = flat-sequence {
                  tunnel: w1013 -> [w1014]
                  frame #0 {
                    n769 = local write "Temp Position"(w1014) -> ()
                  }
                  frame #1 {
                    n770 = local read "Empty"() -> (w1015:cluster{"Left":dbl, "Top":dbl})
                    n771 = property on="Key 7" class="Bool"("Position"=w1015) -> ()  [unwired: 2 in, 2 out]
                  }
                  frame #2 {
                    n772 = local read "Temp Position"() -> (w1016:cluster{"Left":dbl, "Top":dbl})
                    n773 = local write "Empty"(w1016) -> ()
                  }
                }
              }
            }
          }
          frame #1 {
            n774 = property on="Key 5" class="Bool"() -> ("Position"=w1105:T1)  [unwired: 2 in, 2 out]
            n775 = property on="Key 1" class="Bool"() -> ("Position"=w1108:T1)  [unwired: 2 in, 2 out]
            n776 = property on="Key 9" class="Bool"() -> ("Position"=w1098:T1)  [unwired: 2 in, 2 out]
            n777 = property on="Key 13" class="Bool"() -> ("Position"=w1095:T1)  [unwired: 2 in, 2 out]
            n778 = Equal?(x=w1105, y=T1 {"Left"=0, "Top"=80} ("Position")) -> (x = y?=w1102:cluster{"Left":bool, "Top":bool})
            n779 = Equal?(x=w1108, y=T1 {"Left"=0, "Top"=0} ("Position")) -> (x = y?=w1111:cluster{"Left":bool, "Top":bool})
            n780 = Equal?(x=w1098, y=T1 {"Left"=0, "Top"=160} ("Position")) -> (x = y?=w1101:cluster{"Left":bool, "Top":bool})
            n781 = Equal?(x=w1095, y=T1 {"Left"=0, "Top"=240} ("Position")) -> (x = y?=w1092:cluster{"Left":bool, "Top":bool})
            n782 = Unbundle By Name(w1102) -> ("Left"=w1104:bool, "Top"=w1103:bool)
            n783 = Unbundle By Name(w1111) -> ("Left"=w1109:bool, "Top"=w1110:bool)
            n784 = Unbundle By Name(w1101) -> ("Left"=w1099:bool, "Top"=w1100:bool)
            n785 = Unbundle By Name(w1092) -> ("Left"=w1094:bool, "Top"=w1093:bool)
            n786 = And(x=w1104, y=w1103) -> (x .and. y?=w1035:bool)
            n787 = And(x=w1109, y=w1110) -> (x .and. y?=w1036:bool)
            n788 = And(x=w1099, y=w1100) -> (x .and. y?=w1034:bool)
            n789 = And(x=w1094, y=w1093) -> (x .and. y?=w1033:bool)
            n790 = Compound Arithmetic op=AND(w1036, w1035, w1034, w1033) -> (w1021:bool)
            n791 = property on="Key 6" class="Bool"() -> ("Position"=w1078:T1)  [unwired: 2 in, 2 out]
            n792 = property on="Key 2" class="Bool"() -> ("Position"=w1075:T1)  [unwired: 2 in, 2 out]
            n793 = property on="Key 10" class="Bool"() -> ("Position"=w1085:T1)  [unwired: 2 in, 2 out]
            n794 = property on="Key 14" class="Bool"() -> ("Position"=w1088:T1)  [unwired: 2 in, 2 out]
            n795 = Equal?(x=w1078, y=T1 {"Left"=80, "Top"=80} ("Position")) -> (x = y?=w1081:cluster{"Left":bool, "Top":bool})
            n796 = Equal?(x=w1075, y=T1 {"Left"=80, "Top"=0} ("Position")) -> (x = y?=w1072:cluster{"Left":bool, "Top":bool})
            n797 = Equal?(x=w1085, y=T1 {"Left"=80, "Top"=160} ("Position")) -> (x = y?=w1082:cluster{"Left":bool, "Top":bool})
            n798 = Equal?(x=w1088, y=T1 {"Left"=80, "Top"=240} ("Position")) -> (x = y?=w1091:cluster{"Left":bool, "Top":bool})
            n799 = Unbundle By Name(w1081) -> ("Left"=w1079:bool, "Top"=w1080:bool)
            n800 = Unbundle By Name(w1072) -> ("Left"=w1074:bool, "Top"=w1073:bool)
            n801 = Unbundle By Name(w1082) -> ("Left"=w1084:bool, "Top"=w1083:bool)
            n802 = Unbundle By Name(w1091) -> ("Left"=w1089:bool, "Top"=w1090:bool)
            n803 = And(x=w1079, y=w1080) -> (x .and. y?=w1031:bool)
            n804 = And(x=w1074, y=w1073) -> (x .and. y?=w1032:bool)
            n805 = And(x=w1084, y=w1083) -> (x .and. y?=w1030:bool)
            n806 = And(x=w1089, y=w1090) -> (x .and. y?=w1029:bool)
            n807 = Compound Arithmetic op=AND(w1032, w1031, w1030, w1029) -> (w1020:bool)
            n808 = property on="Key 7" class="Bool"() -> ("Position"=w1065:T1)  [unwired: 2 in, 2 out]
            n809 = property on="Key 3" class="Bool"() -> ("Position"=w1068:T1)  [unwired: 2 in, 2 out]
            n810 = property on="Key 11" class="Bool"() -> ("Position"=w1058:T1)  [unwired: 2 in, 2 out]
            n811 = property on="Key 15" class="Bool"() -> ("Position"=w1055:T1)  [unwired: 2 in, 2 out]
            n812 = Equal?(x=w1065, y=T1 {"Left"=160, "Top"=80} ("Position")) -> (x = y?=w1062:cluster{"Left":bool, "Top":bool})
            n813 = Equal?(x=w1068, y=T1 {"Left"=160, "Top"=0} ("Position")) -> (x = y?=w1071:cluster{"Left":bool, "Top":bool})
            n814 = Equal?(x=w1058, y=T1 {"Left"=160, "Top"=160} ("Position")) -> (x = y?=w1061:cluster{"Left":bool, "Top":bool})
            n815 = Equal?(x=w1055, y=T1 {"Left"=160, "Top"=240} ("Position")) -> (x = y?=w1052:cluster{"Left":bool, "Top":bool})
            n816 = Unbundle By Name(w1062) -> ("Left"=w1064:bool, "Top"=w1063:bool)
            n817 = Unbundle By Name(w1071) -> ("Left"=w1069:bool, "Top"=w1070:bool)
            n818 = Unbundle By Name(w1061) -> ("Left"=w1059:bool, "Top"=w1060:bool)
            n819 = Unbundle By Name(w1052) -> ("Left"=w1054:bool, "Top"=w1053:bool)
            n820 = And(x=w1064, y=w1063) -> (x .and. y?=w1027:bool)
            n821 = And(x=w1069, y=w1070) -> (x .and. y?=w1028:bool)
            n822 = And(x=w1059, y=w1060) -> (x .and. y?=w1026:bool)
            n823 = And(x=w1054, y=w1053) -> (x .and. y?=w1025:bool)
            n824 = Compound Arithmetic op=AND(w1028, w1027, w1026, w1025) -> (w1019:bool)
            n825 = property on="Key 8" class="Bool"() -> ("Position"=w1043:T1)  [unwired: 2 in, 2 out]
            n826 = property on="Key 4" class="Bool"() -> ("Position"=w1040:T1)  [unwired: 2 in, 2 out]
            n827 = property on="Key 12" class="Bool"() -> ("Position"=w1050:T1)  [unwired: 2 in, 2 out]
            n828 = Equal?(x=w1043, y=T1 {"Left"=240, "Top"=80} ("Position")) -> (x = y?=w1046:cluster{"Left":bool, "Top":bool})
            n829 = Equal?(x=w1040, y=T1 {"Left"=240, "Top"=0} ("Position")) -> (x = y?=w1037:cluster{"Left":bool, "Top":bool})
            n830 = Equal?(x=w1050, y=T1 {"Left"=240, "Top"=160} ("Position")) -> (x = y?=w1047:cluster{"Left":bool, "Top":bool})
            n831 = Unbundle By Name(w1046) -> ("Left"=w1044:bool, "Top"=w1045:bool)
            n832 = Unbundle By Name(w1037) -> ("Left"=w1039:bool, "Top"=w1038:bool)
            n833 = Unbundle By Name(w1047) -> ("Left"=w1049:bool, "Top"=w1048:bool)
            n834 = And(x=w1044, y=w1045) -> (x .and. y?=w1023:bool)
            n835 = And(x=w1039, y=w1038) -> (x .and. y?=w1024:bool)
            n836 = And(x=w1049, y=w1048) -> (x .and. y?=w1022:bool)
            n837 = Compound Arithmetic op=AND(w1024, w1023, w1022) -> (w1018:bool)
            n838 = Compound Arithmetic op=AND(w1021, w1020, w1019, w1018) -> (w1017:bool)
            n839 = local write "Result"(w1017) -> ()
            n840 = property on="Result" class="Bool (strict)"("Val(Sgnl)"=w1017) -> ()  [unwired: 2 in, 2 out]
          }
        }
      }
      event "Key 8": Value Change {
        n841 = event-data() -> ()  [unwired: 1 in, 6 out]
        n842 = stacked-sequence {
          frame #0 {
            n843 = local read "Moves Number"() -> (w1112:dbl)
            n844 = property on="Key 8" class="Bool"() -> ("Position"=w1114:T1)  [unwired: 2 in, 2 out]
            n845 = Increment(x=w1112) -> (x+1=w1113:dbl)
            n846 = local read "Empty"() -> (w1122:cluster{"Left":dbl, "Top":dbl})
            n847 = local read "Empty"() -> (w1129:cluster{"Left":dbl, "Top":dbl})
            n848 = local read "Empty"() -> (w1141:cluster{"Left":dbl, "Top":dbl})
            n849 = local read "Empty"() -> (w1134:cluster{"Left":dbl, "Top":dbl})
            n850 = Add(x=w1114, y=T1 {"Left"=80, "Top"=0} ("Position")) -> (x+y=w1121:T1)
            n851 = Add(x=w1114, y=T1 {"Left"=0, "Top"=80} ("Position")) -> (x+y=w1130:T1)
            n852 = Subtract(x=w1114, y=T1 {"Left"=80, "Top"=0} ("Position")) -> (x-y=w1142:T1)
            n853 = Subtract(x=w1114, y=T1 {"Left"=0, "Top"=80} ("Position")) -> (x-y=w1133:T1)
            n854 = local write "Moves Number"(w1113) -> ()
            n855 = Equal?(x=w1121, y=w1122) -> (x = y?=w1123:cluster{"Left":bool, "Top":bool})
            n856 = Equal?(x=w1130, y=w1129) -> (x = y?=w1128:cluster{"Left":bool, "Top":bool})
            n857 = Equal?(x=w1142, y=w1141) -> (x = y?=w1140:cluster{"Left":bool, "Top":bool})
            n858 = Equal?(x=w1133, y=w1134) -> (x = y?=w1135:cluster{"Left":bool, "Top":bool})
            n859 = Unbundle By Name(w1123) -> ("Left"=w1125:bool, "Top"=w1124:bool)
            n860 = Unbundle By Name(w1128) -> ("Left"=w1126:bool, "Top"=w1127:bool)
            n861 = Unbundle By Name(w1140) -> ("Left"=w1138:bool, "Top"=w1139:bool)
            n862 = Unbundle By Name(w1135) -> ("Left"=w1137:bool, "Top"=w1136:bool)
            n863 = And(x=w1125, y=w1124) -> (x .and. y?=w1116:bool)
            n864 = And(x=w1126, y=w1127) -> (x .and. y?=w1115:bool)
            n865 = And(x=w1138, y=w1139) -> (x .and. y?=w1118:bool)
            n866 = And(x=w1137, y=w1136) -> (x .and. y?=w1117:bool)
            n867 = Compound Arithmetic op=OR(w1118, w1117, w1116, w1115) -> (w1119:bool)
            n868 = case shown="True" w1119 {
              tunnel: w1114 -> [_ w1144]
              frame False {
              }
              frame True {
                n869 = flat-sequence {
                  tunnel: w1144 -> [w1145]
                  frame #0 {
                    n870 = local write "Temp Position"(w1145) -> ()
                  }
                  frame #1 {
                    n871 = local read "Empty"() -> (w1146:cluster{"Left":dbl, "Top":dbl})
                    n872 = property on="Key 8" class="Bool"("Position"=w1146) -> ()  [unwired: 2 in, 2 out]
                  }
                  frame #2 {
                    n873 = local read "Temp Position"() -> (w1147:cluster{"Left":dbl, "Top":dbl})
                    n874 = local write "Empty"(w1147) -> ()
                  }
                }
              }
            }
          }
          frame #1 {
            n875 = property on="Key 5" class="Bool"() -> ("Position"=w1236:T1)  [unwired: 2 in, 2 out]
            n876 = property on="Key 1" class="Bool"() -> ("Position"=w1239:T1)  [unwired: 2 in, 2 out]
            n877 = property on="Key 9" class="Bool"() -> ("Position"=w1229:T1)  [unwired: 2 in, 2 out]
            n878 = property on="Key 13" class="Bool"() -> ("Position"=w1226:T1)  [unwired: 2 in, 2 out]
            n879 = Equal?(x=w1236, y=T1 {"Left"=0, "Top"=80} ("Position")) -> (x = y?=w1233:cluster{"Left":bool, "Top":bool})
            n880 = Equal?(x=w1239, y=T1 {"Left"=0, "Top"=0} ("Position")) -> (x = y?=w1242:cluster{"Left":bool, "Top":bool})
            n881 = Equal?(x=w1229, y=T1 {"Left"=0, "Top"=160} ("Position")) -> (x = y?=w1232:cluster{"Left":bool, "Top":bool})
            n882 = Equal?(x=w1226, y=T1 {"Left"=0, "Top"=240} ("Position")) -> (x = y?=w1223:cluster{"Left":bool, "Top":bool})
            n883 = Unbundle By Name(w1233) -> ("Left"=w1235:bool, "Top"=w1234:bool)
            n884 = Unbundle By Name(w1242) -> ("Left"=w1240:bool, "Top"=w1241:bool)
            n885 = Unbundle By Name(w1232) -> ("Left"=w1230:bool, "Top"=w1231:bool)
            n886 = Unbundle By Name(w1223) -> ("Left"=w1225:bool, "Top"=w1224:bool)
            n887 = And(x=w1235, y=w1234) -> (x .and. y?=w1166:bool)
            n888 = And(x=w1240, y=w1241) -> (x .and. y?=w1167:bool)
            n889 = And(x=w1230, y=w1231) -> (x .and. y?=w1165:bool)
            n890 = And(x=w1225, y=w1224) -> (x .and. y?=w1164:bool)
            n891 = Compound Arithmetic op=AND(w1167, w1166, w1165, w1164) -> (w1152:bool)
            n892 = property on="Key 6" class="Bool"() -> ("Position"=w1209:T1)  [unwired: 2 in, 2 out]
            n893 = property on="Key 2" class="Bool"() -> ("Position"=w1206:T1)  [unwired: 2 in, 2 out]
            n894 = property on="Key 10" class="Bool"() -> ("Position"=w1216:T1)  [unwired: 2 in, 2 out]
            n895 = property on="Key 14" class="Bool"() -> ("Position"=w1219:T1)  [unwired: 2 in, 2 out]
            n896 = Equal?(x=w1209, y=T1 {"Left"=80, "Top"=80} ("Position")) -> (x = y?=w1212:cluster{"Left":bool, "Top":bool})
            n897 = Equal?(x=w1206, y=T1 {"Left"=80, "Top"=0} ("Position")) -> (x = y?=w1203:cluster{"Left":bool, "Top":bool})
            n898 = Equal?(x=w1216, y=T1 {"Left"=80, "Top"=160} ("Position")) -> (x = y?=w1213:cluster{"Left":bool, "Top":bool})
            n899 = Equal?(x=w1219, y=T1 {"Left"=80, "Top"=240} ("Position")) -> (x = y?=w1222:cluster{"Left":bool, "Top":bool})
            n900 = Unbundle By Name(w1212) -> ("Left"=w1210:bool, "Top"=w1211:bool)
            n901 = Unbundle By Name(w1203) -> ("Left"=w1205:bool, "Top"=w1204:bool)
            n902 = Unbundle By Name(w1213) -> ("Left"=w1215:bool, "Top"=w1214:bool)
            n903 = Unbundle By Name(w1222) -> ("Left"=w1220:bool, "Top"=w1221:bool)
            n904 = And(x=w1210, y=w1211) -> (x .and. y?=w1162:bool)
            n905 = And(x=w1205, y=w1204) -> (x .and. y?=w1163:bool)
            n906 = And(x=w1215, y=w1214) -> (x .and. y?=w1161:bool)
            n907 = And(x=w1220, y=w1221) -> (x .and. y?=w1160:bool)
            n908 = Compound Arithmetic op=AND(w1163, w1162, w1161, w1160) -> (w1151:bool)
            n909 = property on="Key 7" class="Bool"() -> ("Position"=w1196:T1)  [unwired: 2 in, 2 out]
            n910 = property on="Key 3" class="Bool"() -> ("Position"=w1199:T1)  [unwired: 2 in, 2 out]
            n911 = property on="Key 11" class="Bool"() -> ("Position"=w1189:T1)  [unwired: 2 in, 2 out]
            n912 = property on="Key 15" class="Bool"() -> ("Position"=w1186:T1)  [unwired: 2 in, 2 out]
            n913 = Equal?(x=w1196, y=T1 {"Left"=160, "Top"=80} ("Position")) -> (x = y?=w1193:cluster{"Left":bool, "Top":bool})
            n914 = Equal?(x=w1199, y=T1 {"Left"=160, "Top"=0} ("Position")) -> (x = y?=w1202:cluster{"Left":bool, "Top":bool})
            n915 = Equal?(x=w1189, y=T1 {"Left"=160, "Top"=160} ("Position")) -> (x = y?=w1192:cluster{"Left":bool, "Top":bool})
            n916 = Equal?(x=w1186, y=T1 {"Left"=160, "Top"=240} ("Position")) -> (x = y?=w1183:cluster{"Left":bool, "Top":bool})
            n917 = Unbundle By Name(w1193) -> ("Left"=w1195:bool, "Top"=w1194:bool)
            n918 = Unbundle By Name(w1202) -> ("Left"=w1200:bool, "Top"=w1201:bool)
            n919 = Unbundle By Name(w1192) -> ("Left"=w1190:bool, "Top"=w1191:bool)
            n920 = Unbundle By Name(w1183) -> ("Left"=w1185:bool, "Top"=w1184:bool)
            n921 = And(x=w1195, y=w1194) -> (x .and. y?=w1158:bool)
            n922 = And(x=w1200, y=w1201) -> (x .and. y?=w1159:bool)
            n923 = And(x=w1190, y=w1191) -> (x .and. y?=w1157:bool)
            n924 = And(x=w1185, y=w1184) -> (x .and. y?=w1156:bool)
            n925 = Compound Arithmetic op=AND(w1159, w1158, w1157, w1156) -> (w1150:bool)
            n926 = property on="Key 8" class="Bool"() -> ("Position"=w1174:T1)  [unwired: 2 in, 2 out]
            n927 = property on="Key 4" class="Bool"() -> ("Position"=w1171:T1)  [unwired: 2 in, 2 out]
            n928 = property on="Key 12" class="Bool"() -> ("Position"=w1181:T1)  [unwired: 2 in, 2 out]
            n929 = Equal?(x=w1174, y=T1 {"Left"=240, "Top"=80} ("Position")) -> (x = y?=w1177:cluster{"Left":bool, "Top":bool})
            n930 = Equal?(x=w1171, y=T1 {"Left"=240, "Top"=0} ("Position")) -> (x = y?=w1168:cluster{"Left":bool, "Top":bool})
            n931 = Equal?(x=w1181, y=T1 {"Left"=240, "Top"=160} ("Position")) -> (x = y?=w1178:cluster{"Left":bool, "Top":bool})
            n932 = Unbundle By Name(w1177) -> ("Left"=w1175:bool, "Top"=w1176:bool)
            n933 = Unbundle By Name(w1168) -> ("Left"=w1170:bool, "Top"=w1169:bool)
            n934 = Unbundle By Name(w1178) -> ("Left"=w1180:bool, "Top"=w1179:bool)
            n935 = And(x=w1175, y=w1176) -> (x .and. y?=w1154:bool)
            n936 = And(x=w1170, y=w1169) -> (x .and. y?=w1155:bool)
            n937 = And(x=w1180, y=w1179) -> (x .and. y?=w1153:bool)
            n938 = Compound Arithmetic op=AND(w1155, w1154, w1153) -> (w1149:bool)
            n939 = Compound Arithmetic op=AND(w1152, w1151, w1150, w1149) -> (w1148:bool)
            n940 = local write "Result"(w1148) -> ()
            n941 = property on="Result" class="Bool (strict)"("Val(Sgnl)"=w1148) -> ()  [unwired: 2 in, 2 out]
          }
        }
      }
      event "Key 9": Value Change {
        n942 = event-data() -> ()  [unwired: 1 in, 6 out]
        n943 = stacked-sequence {
          frame #0 {
            n944 = local read "Moves Number"() -> (w1243:dbl)
            n945 = property on="Key 9" class="Bool"() -> ("Position"=w1245:T1)  [unwired: 2 in, 2 out]
            n946 = Increment(x=w1243) -> (x+1=w1244:dbl)
            n947 = local read "Empty"() -> (w1253:cluster{"Left":dbl, "Top":dbl})
            n948 = local read "Empty"() -> (w1260:cluster{"Left":dbl, "Top":dbl})
            n949 = local read "Empty"() -> (w1272:cluster{"Left":dbl, "Top":dbl})
            n950 = local read "Empty"() -> (w1265:cluster{"Left":dbl, "Top":dbl})
            n951 = Add(x=w1245, y=T1 {"Left"=80, "Top"=0} ("Position")) -> (x+y=w1252:T1)
            n952 = Add(x=w1245, y=T1 {"Left"=0, "Top"=80} ("Position")) -> (x+y=w1261:T1)
            n953 = Subtract(x=w1245, y=T1 {"Left"=80, "Top"=0} ("Position")) -> (x-y=w1273:T1)
            n954 = Subtract(x=w1245, y=T1 {"Left"=0, "Top"=80} ("Position")) -> (x-y=w1264:T1)
            n955 = local write "Moves Number"(w1244) -> ()
            n956 = Equal?(x=w1252, y=w1253) -> (x = y?=w1254:cluster{"Left":bool, "Top":bool})
            n957 = Equal?(x=w1261, y=w1260) -> (x = y?=w1259:cluster{"Left":bool, "Top":bool})
            n958 = Equal?(x=w1273, y=w1272) -> (x = y?=w1271:cluster{"Left":bool, "Top":bool})
            n959 = Equal?(x=w1264, y=w1265) -> (x = y?=w1266:cluster{"Left":bool, "Top":bool})
            n960 = Unbundle By Name(w1254) -> ("Left"=w1256:bool, "Top"=w1255:bool)
            n961 = Unbundle By Name(w1259) -> ("Left"=w1257:bool, "Top"=w1258:bool)
            n962 = Unbundle By Name(w1271) -> ("Left"=w1269:bool, "Top"=w1270:bool)
            n963 = Unbundle By Name(w1266) -> ("Left"=w1268:bool, "Top"=w1267:bool)
            n964 = And(x=w1256, y=w1255) -> (x .and. y?=w1247:bool)
            n965 = And(x=w1257, y=w1258) -> (x .and. y?=w1246:bool)
            n966 = And(x=w1269, y=w1270) -> (x .and. y?=w1249:bool)
            n967 = And(x=w1268, y=w1267) -> (x .and. y?=w1248:bool)
            n968 = Compound Arithmetic op=OR(w1249, w1248, w1247, w1246) -> (w1250:bool)
            n969 = case shown="True" w1250 {
              tunnel: w1245 -> [_ w1275]
              frame False {
              }
              frame True {
                n970 = flat-sequence {
                  tunnel: w1275 -> [w1276]
                  frame #0 {
                    n971 = local write "Temp Position"(w1276) -> ()
                  }
                  frame #1 {
                    n972 = local read "Empty"() -> (w1277:cluster{"Left":dbl, "Top":dbl})
                    n973 = property on="Key 9" class="Bool"("Position"=w1277) -> ()  [unwired: 2 in, 2 out]
                  }
                  frame #2 {
                    n974 = local read "Temp Position"() -> (w1278:cluster{"Left":dbl, "Top":dbl})
                    n975 = local write "Empty"(w1278) -> ()
                  }
                }
              }
            }
          }
          frame #1 {
            n976 = property on="Key 5" class="Bool"() -> ("Position"=w1367:T1)  [unwired: 2 in, 2 out]
            n977 = property on="Key 1" class="Bool"() -> ("Position"=w1370:T1)  [unwired: 2 in, 2 out]
            n978 = property on="Key 9" class="Bool"() -> ("Position"=w1360:T1)  [unwired: 2 in, 2 out]
            n979 = property on="Key 13" class="Bool"() -> ("Position"=w1357:T1)  [unwired: 2 in, 2 out]
            n980 = Equal?(x=w1367, y=T1 {"Left"=0, "Top"=80} ("Position")) -> (x = y?=w1364:cluster{"Left":bool, "Top":bool})
            n981 = Equal?(x=w1370, y=T1 {"Left"=0, "Top"=0} ("Position")) -> (x = y?=w1373:cluster{"Left":bool, "Top":bool})
            n982 = Equal?(x=w1360, y=T1 {"Left"=0, "Top"=160} ("Position")) -> (x = y?=w1363:cluster{"Left":bool, "Top":bool})
            n983 = Equal?(x=w1357, y=T1 {"Left"=0, "Top"=240} ("Position")) -> (x = y?=w1354:cluster{"Left":bool, "Top":bool})
            n984 = Unbundle By Name(w1364) -> ("Left"=w1366:bool, "Top"=w1365:bool)
            n985 = Unbundle By Name(w1373) -> ("Left"=w1371:bool, "Top"=w1372:bool)
            n986 = Unbundle By Name(w1363) -> ("Left"=w1361:bool, "Top"=w1362:bool)
            n987 = Unbundle By Name(w1354) -> ("Left"=w1356:bool, "Top"=w1355:bool)
            n988 = And(x=w1366, y=w1365) -> (x .and. y?=w1297:bool)
            n989 = And(x=w1371, y=w1372) -> (x .and. y?=w1298:bool)
            n990 = And(x=w1361, y=w1362) -> (x .and. y?=w1296:bool)
            n991 = And(x=w1356, y=w1355) -> (x .and. y?=w1295:bool)
            n992 = Compound Arithmetic op=AND(w1298, w1297, w1296, w1295) -> (w1283:bool)
            n993 = property on="Key 6" class="Bool"() -> ("Position"=w1340:T1)  [unwired: 2 in, 2 out]
            n994 = property on="Key 2" class="Bool"() -> ("Position"=w1337:T1)  [unwired: 2 in, 2 out]
            n995 = property on="Key 10" class="Bool"() -> ("Position"=w1347:T1)  [unwired: 2 in, 2 out]
            n996 = property on="Key 14" class="Bool"() -> ("Position"=w1350:T1)  [unwired: 2 in, 2 out]
            n997 = Equal?(x=w1340, y=T1 {"Left"=80, "Top"=80} ("Position")) -> (x = y?=w1343:cluster{"Left":bool, "Top":bool})
            n998 = Equal?(x=w1337, y=T1 {"Left"=80, "Top"=0} ("Position")) -> (x = y?=w1334:cluster{"Left":bool, "Top":bool})
            n999 = Equal?(x=w1347, y=T1 {"Left"=80, "Top"=160} ("Position")) -> (x = y?=w1344:cluster{"Left":bool, "Top":bool})
            n1000 = Equal?(x=w1350, y=T1 {"Left"=80, "Top"=240} ("Position")) -> (x = y?=w1353:cluster{"Left":bool, "Top":bool})
            n1001 = Unbundle By Name(w1343) -> ("Left"=w1341:bool, "Top"=w1342:bool)
            n1002 = Unbundle By Name(w1334) -> ("Left"=w1336:bool, "Top"=w1335:bool)
            n1003 = Unbundle By Name(w1344) -> ("Left"=w1346:bool, "Top"=w1345:bool)
            n1004 = Unbundle By Name(w1353) -> ("Left"=w1351:bool, "Top"=w1352:bool)
            n1005 = And(x=w1341, y=w1342) -> (x .and. y?=w1293:bool)
            n1006 = And(x=w1336, y=w1335) -> (x .and. y?=w1294:bool)
            n1007 = And(x=w1346, y=w1345) -> (x .and. y?=w1292:bool)
            n1008 = And(x=w1351, y=w1352) -> (x .and. y?=w1291:bool)
            n1009 = Compound Arithmetic op=AND(w1294, w1293, w1292, w1291) -> (w1282:bool)
            n1010 = property on="Key 7" class="Bool"() -> ("Position"=w1327:T1)  [unwired: 2 in, 2 out]
            n1011 = property on="Key 3" class="Bool"() -> ("Position"=w1330:T1)  [unwired: 2 in, 2 out]
            n1012 = property on="Key 11" class="Bool"() -> ("Position"=w1320:T1)  [unwired: 2 in, 2 out]
            n1013 = property on="Key 15" class="Bool"() -> ("Position"=w1317:T1)  [unwired: 2 in, 2 out]
            n1014 = Equal?(x=w1327, y=T1 {"Left"=160, "Top"=80} ("Position")) -> (x = y?=w1324:cluster{"Left":bool, "Top":bool})
            n1015 = Equal?(x=w1330, y=T1 {"Left"=160, "Top"=0} ("Position")) -> (x = y?=w1333:cluster{"Left":bool, "Top":bool})
            n1016 = Equal?(x=w1320, y=T1 {"Left"=160, "Top"=160} ("Position")) -> (x = y?=w1323:cluster{"Left":bool, "Top":bool})
            n1017 = Equal?(x=w1317, y=T1 {"Left"=160, "Top"=240} ("Position")) -> (x = y?=w1314:cluster{"Left":bool, "Top":bool})
            n1018 = Unbundle By Name(w1324) -> ("Left"=w1326:bool, "Top"=w1325:bool)
            n1019 = Unbundle By Name(w1333) -> ("Left"=w1331:bool, "Top"=w1332:bool)
            n1020 = Unbundle By Name(w1323) -> ("Left"=w1321:bool, "Top"=w1322:bool)
            n1021 = Unbundle By Name(w1314) -> ("Left"=w1316:bool, "Top"=w1315:bool)
            n1022 = And(x=w1326, y=w1325) -> (x .and. y?=w1289:bool)
            n1023 = And(x=w1331, y=w1332) -> (x .and. y?=w1290:bool)
            n1024 = And(x=w1321, y=w1322) -> (x .and. y?=w1288:bool)
            n1025 = And(x=w1316, y=w1315) -> (x .and. y?=w1287:bool)
            n1026 = Compound Arithmetic op=AND(w1290, w1289, w1288, w1287) -> (w1281:bool)
            n1027 = property on="Key 8" class="Bool"() -> ("Position"=w1305:T1)  [unwired: 2 in, 2 out]
            n1028 = property on="Key 4" class="Bool"() -> ("Position"=w1302:T1)  [unwired: 2 in, 2 out]
            n1029 = property on="Key 12" class="Bool"() -> ("Position"=w1312:T1)  [unwired: 2 in, 2 out]
            n1030 = Equal?(x=w1305, y=T1 {"Left"=240, "Top"=80} ("Position")) -> (x = y?=w1308:cluster{"Left":bool, "Top":bool})
            n1031 = Equal?(x=w1302, y=T1 {"Left"=240, "Top"=0} ("Position")) -> (x = y?=w1299:cluster{"Left":bool, "Top":bool})
            n1032 = Equal?(x=w1312, y=T1 {"Left"=240, "Top"=160} ("Position")) -> (x = y?=w1309:cluster{"Left":bool, "Top":bool})
            n1033 = Unbundle By Name(w1308) -> ("Left"=w1306:bool, "Top"=w1307:bool)
            n1034 = Unbundle By Name(w1299) -> ("Left"=w1301:bool, "Top"=w1300:bool)
            n1035 = Unbundle By Name(w1309) -> ("Left"=w1311:bool, "Top"=w1310:bool)
            n1036 = And(x=w1306, y=w1307) -> (x .and. y?=w1285:bool)
            n1037 = And(x=w1301, y=w1300) -> (x .and. y?=w1286:bool)
            n1038 = And(x=w1311, y=w1310) -> (x .and. y?=w1284:bool)
            n1039 = Compound Arithmetic op=AND(w1286, w1285, w1284) -> (w1280:bool)
            n1040 = Compound Arithmetic op=AND(w1283, w1282, w1281, w1280) -> (w1279:bool)
            n1041 = local write "Result"(w1279) -> ()
            n1042 = property on="Result" class="Bool (strict)"("Val(Sgnl)"=w1279) -> ()  [unwired: 2 in, 2 out]
          }
        }
      }
      event "Key 10": Value Change {
        n1043 = event-data() -> ()  [unwired: 1 in, 6 out]
        n1044 = stacked-sequence {
          frame #0 {
            n1045 = local read "Moves Number"() -> (w1374:dbl)
            n1046 = property on="Key 10" class="Bool"() -> ("Position"=w1376:T1)  [unwired: 2 in, 2 out]
            n1047 = Increment(x=w1374) -> (x+1=w1375:dbl)
            n1048 = local read "Empty"() -> (w1384:cluster{"Left":dbl, "Top":dbl})
            n1049 = local read "Empty"() -> (w1391:cluster{"Left":dbl, "Top":dbl})
            n1050 = local read "Empty"() -> (w1403:cluster{"Left":dbl, "Top":dbl})
            n1051 = local read "Empty"() -> (w1396:cluster{"Left":dbl, "Top":dbl})
            n1052 = Add(x=w1376, y=T1 {"Left"=80, "Top"=0} ("Position")) -> (x+y=w1383:T1)
            n1053 = Add(x=w1376, y=T1 {"Left"=0, "Top"=80} ("Position")) -> (x+y=w1392:T1)
            n1054 = Subtract(x=w1376, y=T1 {"Left"=80, "Top"=0} ("Position")) -> (x-y=w1404:T1)
            n1055 = Subtract(x=w1376, y=T1 {"Left"=0, "Top"=80} ("Position")) -> (x-y=w1395:T1)
            n1056 = local write "Moves Number"(w1375) -> ()
            n1057 = Equal?(x=w1383, y=w1384) -> (x = y?=w1385:cluster{"Left":bool, "Top":bool})
            n1058 = Equal?(x=w1392, y=w1391) -> (x = y?=w1390:cluster{"Left":bool, "Top":bool})
            n1059 = Equal?(x=w1404, y=w1403) -> (x = y?=w1402:cluster{"Left":bool, "Top":bool})
            n1060 = Equal?(x=w1395, y=w1396) -> (x = y?=w1397:cluster{"Left":bool, "Top":bool})
            n1061 = Unbundle By Name(w1385) -> ("Left"=w1387:bool, "Top"=w1386:bool)
            n1062 = Unbundle By Name(w1390) -> ("Left"=w1388:bool, "Top"=w1389:bool)
            n1063 = Unbundle By Name(w1402) -> ("Left"=w1400:bool, "Top"=w1401:bool)
            n1064 = Unbundle By Name(w1397) -> ("Left"=w1399:bool, "Top"=w1398:bool)
            n1065 = And(x=w1387, y=w1386) -> (x .and. y?=w1378:bool)
            n1066 = And(x=w1388, y=w1389) -> (x .and. y?=w1377:bool)
            n1067 = And(x=w1400, y=w1401) -> (x .and. y?=w1380:bool)
            n1068 = And(x=w1399, y=w1398) -> (x .and. y?=w1379:bool)
            n1069 = Compound Arithmetic op=OR(w1380, w1379, w1378, w1377) -> (w1381:bool)
            n1070 = case shown="True" w1381 {
              tunnel: w1376 -> [_ w1406]
              frame False {
              }
              frame True {
                n1071 = flat-sequence {
                  tunnel: w1406 -> [w1407]
                  frame #0 {
                    n1072 = local write "Temp Position"(w1407) -> ()
                  }
                  frame #1 {
                    n1073 = local read "Empty"() -> (w1408:cluster{"Left":dbl, "Top":dbl})
                    n1074 = property on="Key 10" class="Bool"("Position"=w1408) -> ()  [unwired: 2 in, 2 out]
                  }
                  frame #2 {
                    n1075 = local read "Temp Position"() -> (w1409:cluster{"Left":dbl, "Top":dbl})
                    n1076 = local write "Empty"(w1409) -> ()
                  }
                }
              }
            }
          }
          frame #1 {
            n1077 = property on="Key 5" class="Bool"() -> ("Position"=w1498:T1)  [unwired: 2 in, 2 out]
            n1078 = property on="Key 1" class="Bool"() -> ("Position"=w1501:T1)  [unwired: 2 in, 2 out]
            n1079 = property on="Key 9" class="Bool"() -> ("Position"=w1491:T1)  [unwired: 2 in, 2 out]
            n1080 = property on="Key 13" class="Bool"() -> ("Position"=w1488:T1)  [unwired: 2 in, 2 out]
            n1081 = Equal?(x=w1498, y=T1 {"Left"=0, "Top"=80} ("Position")) -> (x = y?=w1495:cluster{"Left":bool, "Top":bool})
            n1082 = Equal?(x=w1501, y=T1 {"Left"=0, "Top"=0} ("Position")) -> (x = y?=w1504:cluster{"Left":bool, "Top":bool})
            n1083 = Equal?(x=w1491, y=T1 {"Left"=0, "Top"=160} ("Position")) -> (x = y?=w1494:cluster{"Left":bool, "Top":bool})
            n1084 = Equal?(x=w1488, y=T1 {"Left"=0, "Top"=240} ("Position")) -> (x = y?=w1485:cluster{"Left":bool, "Top":bool})
            n1085 = Unbundle By Name(w1495) -> ("Left"=w1497:bool, "Top"=w1496:bool)
            n1086 = Unbundle By Name(w1504) -> ("Left"=w1502:bool, "Top"=w1503:bool)
            n1087 = Unbundle By Name(w1494) -> ("Left"=w1492:bool, "Top"=w1493:bool)
            n1088 = Unbundle By Name(w1485) -> ("Left"=w1487:bool, "Top"=w1486:bool)
            n1089 = And(x=w1497, y=w1496) -> (x .and. y?=w1428:bool)
            n1090 = And(x=w1502, y=w1503) -> (x .and. y?=w1429:bool)
            n1091 = And(x=w1492, y=w1493) -> (x .and. y?=w1427:bool)
            n1092 = And(x=w1487, y=w1486) -> (x .and. y?=w1426:bool)
            n1093 = Compound Arithmetic op=AND(w1429, w1428, w1427, w1426) -> (w1414:bool)
            n1094 = property on="Key 6" class="Bool"() -> ("Position"=w1471:T1)  [unwired: 2 in, 2 out]
            n1095 = property on="Key 2" class="Bool"() -> ("Position"=w1468:T1)  [unwired: 2 in, 2 out]
            n1096 = property on="Key 10" class="Bool"() -> ("Position"=w1478:T1)  [unwired: 2 in, 2 out]
            n1097 = property on="Key 14" class="Bool"() -> ("Position"=w1481:T1)  [unwired: 2 in, 2 out]
            n1098 = Equal?(x=w1471, y=T1 {"Left"=80, "Top"=80} ("Position")) -> (x = y?=w1474:cluster{"Left":bool, "Top":bool})
            n1099 = Equal?(x=w1468, y=T1 {"Left"=80, "Top"=0} ("Position")) -> (x = y?=w1465:cluster{"Left":bool, "Top":bool})
            n1100 = Equal?(x=w1478, y=T1 {"Left"=80, "Top"=160} ("Position")) -> (x = y?=w1475:cluster{"Left":bool, "Top":bool})
            n1101 = Equal?(x=w1481, y=T1 {"Left"=80, "Top"=240} ("Position")) -> (x = y?=w1484:cluster{"Left":bool, "Top":bool})
            n1102 = Unbundle By Name(w1474) -> ("Left"=w1472:bool, "Top"=w1473:bool)
            n1103 = Unbundle By Name(w1465) -> ("Left"=w1467:bool, "Top"=w1466:bool)
            n1104 = Unbundle By Name(w1475) -> ("Left"=w1477:bool, "Top"=w1476:bool)
            n1105 = Unbundle By Name(w1484) -> ("Left"=w1482:bool, "Top"=w1483:bool)
            n1106 = And(x=w1472, y=w1473) -> (x .and. y?=w1424:bool)
            n1107 = And(x=w1467, y=w1466) -> (x .and. y?=w1425:bool)
            n1108 = And(x=w1477, y=w1476) -> (x .and. y?=w1423:bool)
            n1109 = And(x=w1482, y=w1483) -> (x .and. y?=w1422:bool)
            n1110 = Compound Arithmetic op=AND(w1425, w1424, w1423, w1422) -> (w1413:bool)
            n1111 = property on="Key 7" class="Bool"() -> ("Position"=w1458:T1)  [unwired: 2 in, 2 out]
            n1112 = property on="Key 3" class="Bool"() -> ("Position"=w1461:T1)  [unwired: 2 in, 2 out]
            n1113 = property on="Key 11" class="Bool"() -> ("Position"=w1451:T1)  [unwired: 2 in, 2 out]
            n1114 = property on="Key 15" class="Bool"() -> ("Position"=w1448:T1)  [unwired: 2 in, 2 out]
            n1115 = Equal?(x=w1458, y=T1 {"Left"=160, "Top"=80} ("Position")) -> (x = y?=w1455:cluster{"Left":bool, "Top":bool})
            n1116 = Equal?(x=w1461, y=T1 {"Left"=160, "Top"=0} ("Position")) -> (x = y?=w1464:cluster{"Left":bool, "Top":bool})
            n1117 = Equal?(x=w1451, y=T1 {"Left"=160, "Top"=160} ("Position")) -> (x = y?=w1454:cluster{"Left":bool, "Top":bool})
            n1118 = Equal?(x=w1448, y=T1 {"Left"=160, "Top"=240} ("Position")) -> (x = y?=w1445:cluster{"Left":bool, "Top":bool})
            n1119 = Unbundle By Name(w1455) -> ("Left"=w1457:bool, "Top"=w1456:bool)
            n1120 = Unbundle By Name(w1464) -> ("Left"=w1462:bool, "Top"=w1463:bool)
            n1121 = Unbundle By Name(w1454) -> ("Left"=w1452:bool, "Top"=w1453:bool)
            n1122 = Unbundle By Name(w1445) -> ("Left"=w1447:bool, "Top"=w1446:bool)
            n1123 = And(x=w1457, y=w1456) -> (x .and. y?=w1420:bool)
            n1124 = And(x=w1462, y=w1463) -> (x .and. y?=w1421:bool)
            n1125 = And(x=w1452, y=w1453) -> (x .and. y?=w1419:bool)
            n1126 = And(x=w1447, y=w1446) -> (x .and. y?=w1418:bool)
            n1127 = Compound Arithmetic op=AND(w1421, w1420, w1419, w1418) -> (w1412:bool)
            n1128 = property on="Key 8" class="Bool"() -> ("Position"=w1436:T1)  [unwired: 2 in, 2 out]
            n1129 = property on="Key 4" class="Bool"() -> ("Position"=w1433:T1)  [unwired: 2 in, 2 out]
            n1130 = property on="Key 12" class="Bool"() -> ("Position"=w1443:T1)  [unwired: 2 in, 2 out]
            n1131 = Equal?(x=w1436, y=T1 {"Left"=240, "Top"=80} ("Position")) -> (x = y?=w1439:cluster{"Left":bool, "Top":bool})
            n1132 = Equal?(x=w1433, y=T1 {"Left"=240, "Top"=0} ("Position")) -> (x = y?=w1430:cluster{"Left":bool, "Top":bool})
            n1133 = Equal?(x=w1443, y=T1 {"Left"=240, "Top"=160} ("Position")) -> (x = y?=w1440:cluster{"Left":bool, "Top":bool})
            n1134 = Unbundle By Name(w1439) -> ("Left"=w1437:bool, "Top"=w1438:bool)
            n1135 = Unbundle By Name(w1430) -> ("Left"=w1432:bool, "Top"=w1431:bool)
            n1136 = Unbundle By Name(w1440) -> ("Left"=w1442:bool, "Top"=w1441:bool)
            n1137 = And(x=w1437, y=w1438) -> (x .and. y?=w1416:bool)
            n1138 = And(x=w1432, y=w1431) -> (x .and. y?=w1417:bool)
            n1139 = And(x=w1442, y=w1441) -> (x .and. y?=w1415:bool)
            n1140 = Compound Arithmetic op=AND(w1417, w1416, w1415) -> (w1411:bool)
            n1141 = Compound Arithmetic op=AND(w1414, w1413, w1412, w1411) -> (w1410:bool)
            n1142 = local write "Result"(w1410) -> ()
            n1143 = property on="Result" class="Bool (strict)"("Val(Sgnl)"=w1410) -> ()  [unwired: 2 in, 2 out]
          }
        }
      }
      event "Key 11": Value Change {
        n1144 = event-data() -> ()  [unwired: 1 in, 6 out]
        n1145 = stacked-sequence {
          frame #0 {
            n1146 = local read "Moves Number"() -> (w1505:dbl)
            n1147 = property on="Key 11" class="Bool"() -> ("Position"=w1507:T1)  [unwired: 2 in, 2 out]
            n1148 = Increment(x=w1505) -> (x+1=w1506:dbl)
            n1149 = local read "Empty"() -> (w1515:cluster{"Left":dbl, "Top":dbl})
            n1150 = local read "Empty"() -> (w1522:cluster{"Left":dbl, "Top":dbl})
            n1151 = local read "Empty"() -> (w1534:cluster{"Left":dbl, "Top":dbl})
            n1152 = local read "Empty"() -> (w1527:cluster{"Left":dbl, "Top":dbl})
            n1153 = Add(x=w1507, y=T1 {"Left"=80, "Top"=0} ("Position")) -> (x+y=w1514:T1)
            n1154 = Add(x=w1507, y=T1 {"Left"=0, "Top"=80} ("Position")) -> (x+y=w1523:T1)
            n1155 = Subtract(x=w1507, y=T1 {"Left"=80, "Top"=0} ("Position")) -> (x-y=w1535:T1)
            n1156 = Subtract(x=w1507, y=T1 {"Left"=0, "Top"=80} ("Position")) -> (x-y=w1526:T1)
            n1157 = local write "Moves Number"(w1506) -> ()
            n1158 = Equal?(x=w1514, y=w1515) -> (x = y?=w1516:cluster{"Left":bool, "Top":bool})
            n1159 = Equal?(x=w1523, y=w1522) -> (x = y?=w1521:cluster{"Left":bool, "Top":bool})
            n1160 = Equal?(x=w1535, y=w1534) -> (x = y?=w1533:cluster{"Left":bool, "Top":bool})
            n1161 = Equal?(x=w1526, y=w1527) -> (x = y?=w1528:cluster{"Left":bool, "Top":bool})
            n1162 = Unbundle By Name(w1516) -> ("Left"=w1518:bool, "Top"=w1517:bool)
            n1163 = Unbundle By Name(w1521) -> ("Left"=w1519:bool, "Top"=w1520:bool)
            n1164 = Unbundle By Name(w1533) -> ("Left"=w1531:bool, "Top"=w1532:bool)
            n1165 = Unbundle By Name(w1528) -> ("Left"=w1530:bool, "Top"=w1529:bool)
            n1166 = And(x=w1518, y=w1517) -> (x .and. y?=w1509:bool)
            n1167 = And(x=w1519, y=w1520) -> (x .and. y?=w1508:bool)
            n1168 = And(x=w1531, y=w1532) -> (x .and. y?=w1511:bool)
            n1169 = And(x=w1530, y=w1529) -> (x .and. y?=w1510:bool)
            n1170 = Compound Arithmetic op=OR(w1511, w1510, w1509, w1508) -> (w1512:bool)
            n1171 = case shown="True" w1512 {
              tunnel: w1507 -> [_ w1537]
              frame False {
              }
              frame True {
                n1172 = flat-sequence {
                  tunnel: w1537 -> [w1538]
                  frame #0 {
                    n1173 = local write "Temp Position"(w1538) -> ()
                  }
                  frame #1 {
                    n1174 = local read "Empty"() -> (w1539:cluster{"Left":dbl, "Top":dbl})
                    n1175 = property on="Key 11" class="Bool"("Position"=w1539) -> ()  [unwired: 2 in, 2 out]
                  }
                  frame #2 {
                    n1176 = local read "Temp Position"() -> (w1540:cluster{"Left":dbl, "Top":dbl})
                    n1177 = local write "Empty"(w1540) -> ()
                  }
                }
              }
            }
          }
          frame #1 {
            n1178 = property on="Key 5" class="Bool"() -> ("Position"=w1629:T1)  [unwired: 2 in, 2 out]
            n1179 = property on="Key 1" class="Bool"() -> ("Position"=w1632:T1)  [unwired: 2 in, 2 out]
            n1180 = property on="Key 9" class="Bool"() -> ("Position"=w1622:T1)  [unwired: 2 in, 2 out]
            n1181 = property on="Key 13" class="Bool"() -> ("Position"=w1619:T1)  [unwired: 2 in, 2 out]
            n1182 = Equal?(x=w1629, y=T1 {"Left"=0, "Top"=80} ("Position")) -> (x = y?=w1626:cluster{"Left":bool, "Top":bool})
            n1183 = Equal?(x=w1632, y=T1 {"Left"=0, "Top"=0} ("Position")) -> (x = y?=w1635:cluster{"Left":bool, "Top":bool})
            n1184 = Equal?(x=w1622, y=T1 {"Left"=0, "Top"=160} ("Position")) -> (x = y?=w1625:cluster{"Left":bool, "Top":bool})
            n1185 = Equal?(x=w1619, y=T1 {"Left"=0, "Top"=240} ("Position")) -> (x = y?=w1616:cluster{"Left":bool, "Top":bool})
            n1186 = Unbundle By Name(w1626) -> ("Left"=w1628:bool, "Top"=w1627:bool)
            n1187 = Unbundle By Name(w1635) -> ("Left"=w1633:bool, "Top"=w1634:bool)
            n1188 = Unbundle By Name(w1625) -> ("Left"=w1623:bool, "Top"=w1624:bool)
            n1189 = Unbundle By Name(w1616) -> ("Left"=w1618:bool, "Top"=w1617:bool)
            n1190 = And(x=w1628, y=w1627) -> (x .and. y?=w1559:bool)
            n1191 = And(x=w1633, y=w1634) -> (x .and. y?=w1560:bool)
            n1192 = And(x=w1623, y=w1624) -> (x .and. y?=w1558:bool)
            n1193 = And(x=w1618, y=w1617) -> (x .and. y?=w1557:bool)
            n1194 = Compound Arithmetic op=AND(w1560, w1559, w1558, w1557) -> (w1545:bool)
            n1195 = property on="Key 6" class="Bool"() -> ("Position"=w1602:T1)  [unwired: 2 in, 2 out]
            n1196 = property on="Key 2" class="Bool"() -> ("Position"=w1599:T1)  [unwired: 2 in, 2 out]
            n1197 = property on="Key 10" class="Bool"() -> ("Position"=w1609:T1)  [unwired: 2 in, 2 out]
            n1198 = property on="Key 14" class="Bool"() -> ("Position"=w1612:T1)  [unwired: 2 in, 2 out]
            n1199 = Equal?(x=w1602, y=T1 {"Left"=80, "Top"=80} ("Position")) -> (x = y?=w1605:cluster{"Left":bool, "Top":bool})
            n1200 = Equal?(x=w1599, y=T1 {"Left"=80, "Top"=0} ("Position")) -> (x = y?=w1596:cluster{"Left":bool, "Top":bool})
            n1201 = Equal?(x=w1609, y=T1 {"Left"=80, "Top"=160} ("Position")) -> (x = y?=w1606:cluster{"Left":bool, "Top":bool})
            n1202 = Equal?(x=w1612, y=T1 {"Left"=80, "Top"=240} ("Position")) -> (x = y?=w1615:cluster{"Left":bool, "Top":bool})
            n1203 = Unbundle By Name(w1605) -> ("Left"=w1603:bool, "Top"=w1604:bool)
            n1204 = Unbundle By Name(w1596) -> ("Left"=w1598:bool, "Top"=w1597:bool)
            n1205 = Unbundle By Name(w1606) -> ("Left"=w1608:bool, "Top"=w1607:bool)
            n1206 = Unbundle By Name(w1615) -> ("Left"=w1613:bool, "Top"=w1614:bool)
            n1207 = And(x=w1603, y=w1604) -> (x .and. y?=w1555:bool)
            n1208 = And(x=w1598, y=w1597) -> (x .and. y?=w1556:bool)
            n1209 = And(x=w1608, y=w1607) -> (x .and. y?=w1554:bool)
            n1210 = And(x=w1613, y=w1614) -> (x .and. y?=w1553:bool)
            n1211 = Compound Arithmetic op=AND(w1556, w1555, w1554, w1553) -> (w1544:bool)
            n1212 = property on="Key 7" class="Bool"() -> ("Position"=w1589:T1)  [unwired: 2 in, 2 out]
            n1213 = property on="Key 3" class="Bool"() -> ("Position"=w1592:T1)  [unwired: 2 in, 2 out]
            n1214 = property on="Key 11" class="Bool"() -> ("Position"=w1582:T1)  [unwired: 2 in, 2 out]
            n1215 = property on="Key 15" class="Bool"() -> ("Position"=w1579:T1)  [unwired: 2 in, 2 out]
            n1216 = Equal?(x=w1589, y=T1 {"Left"=160, "Top"=80} ("Position")) -> (x = y?=w1586:cluster{"Left":bool, "Top":bool})
            n1217 = Equal?(x=w1592, y=T1 {"Left"=160, "Top"=0} ("Position")) -> (x = y?=w1595:cluster{"Left":bool, "Top":bool})
            n1218 = Equal?(x=w1582, y=T1 {"Left"=160, "Top"=160} ("Position")) -> (x = y?=w1585:cluster{"Left":bool, "Top":bool})
            n1219 = Equal?(x=w1579, y=T1 {"Left"=160, "Top"=240} ("Position")) -> (x = y?=w1576:cluster{"Left":bool, "Top":bool})
            n1220 = Unbundle By Name(w1586) -> ("Left"=w1588:bool, "Top"=w1587:bool)
            n1221 = Unbundle By Name(w1595) -> ("Left"=w1593:bool, "Top"=w1594:bool)
            n1222 = Unbundle By Name(w1585) -> ("Left"=w1583:bool, "Top"=w1584:bool)
            n1223 = Unbundle By Name(w1576) -> ("Left"=w1578:bool, "Top"=w1577:bool)
            n1224 = And(x=w1588, y=w1587) -> (x .and. y?=w1551:bool)
            n1225 = And(x=w1593, y=w1594) -> (x .and. y?=w1552:bool)
            n1226 = And(x=w1583, y=w1584) -> (x .and. y?=w1550:bool)
            n1227 = And(x=w1578, y=w1577) -> (x .and. y?=w1549:bool)
            n1228 = Compound Arithmetic op=AND(w1552, w1551, w1550, w1549) -> (w1543:bool)
            n1229 = property on="Key 8" class="Bool"() -> ("Position"=w1567:T1)  [unwired: 2 in, 2 out]
            n1230 = property on="Key 4" class="Bool"() -> ("Position"=w1564:T1)  [unwired: 2 in, 2 out]
            n1231 = property on="Key 12" class="Bool"() -> ("Position"=w1574:T1)  [unwired: 2 in, 2 out]
            n1232 = Equal?(x=w1567, y=T1 {"Left"=240, "Top"=80} ("Position")) -> (x = y?=w1570:cluster{"Left":bool, "Top":bool})
            n1233 = Equal?(x=w1564, y=T1 {"Left"=240, "Top"=0} ("Position")) -> (x = y?=w1561:cluster{"Left":bool, "Top":bool})
            n1234 = Equal?(x=w1574, y=T1 {"Left"=240, "Top"=160} ("Position")) -> (x = y?=w1571:cluster{"Left":bool, "Top":bool})
            n1235 = Unbundle By Name(w1570) -> ("Left"=w1568:bool, "Top"=w1569:bool)
            n1236 = Unbundle By Name(w1561) -> ("Left"=w1563:bool, "Top"=w1562:bool)
            n1237 = Unbundle By Name(w1571) -> ("Left"=w1573:bool, "Top"=w1572:bool)
            n1238 = And(x=w1568, y=w1569) -> (x .and. y?=w1547:bool)
            n1239 = And(x=w1563, y=w1562) -> (x .and. y?=w1548:bool)
            n1240 = And(x=w1573, y=w1572) -> (x .and. y?=w1546:bool)
            n1241 = Compound Arithmetic op=AND(w1548, w1547, w1546) -> (w1542:bool)
            n1242 = Compound Arithmetic op=AND(w1545, w1544, w1543, w1542) -> (w1541:bool)
            n1243 = local write "Result"(w1541) -> ()
            n1244 = property on="Result" class="Bool (strict)"("Val(Sgnl)"=w1541) -> ()  [unwired: 2 in, 2 out]
          }
        }
      }
      event "Key 12": Value Change {
        n1245 = event-data() -> ()  [unwired: 1 in, 6 out]
        n1246 = stacked-sequence {
          frame #0 {
            n1247 = local read "Moves Number"() -> (w1636:dbl)
            n1248 = property on="Key 12" class="Bool"() -> ("Position"=w1638:T1)  [unwired: 2 in, 2 out]
            n1249 = Increment(x=w1636) -> (x+1=w1637:dbl)
            n1250 = local read "Empty"() -> (w1646:cluster{"Left":dbl, "Top":dbl})
            n1251 = local read "Empty"() -> (w1653:cluster{"Left":dbl, "Top":dbl})
            n1252 = local read "Empty"() -> (w1665:cluster{"Left":dbl, "Top":dbl})
            n1253 = local read "Empty"() -> (w1658:cluster{"Left":dbl, "Top":dbl})
            n1254 = Add(x=w1638, y=T1 {"Left"=80, "Top"=0} ("Position")) -> (x+y=w1645:T1)
            n1255 = Add(x=w1638, y=T1 {"Left"=0, "Top"=80} ("Position")) -> (x+y=w1654:T1)
            n1256 = Subtract(x=w1638, y=T1 {"Left"=80, "Top"=0} ("Position")) -> (x-y=w1666:T1)
            n1257 = Subtract(x=w1638, y=T1 {"Left"=0, "Top"=80} ("Position")) -> (x-y=w1657:T1)
            n1258 = local write "Moves Number"(w1637) -> ()
            n1259 = Equal?(x=w1645, y=w1646) -> (x = y?=w1647:cluster{"Left":bool, "Top":bool})
            n1260 = Equal?(x=w1654, y=w1653) -> (x = y?=w1652:cluster{"Left":bool, "Top":bool})
            n1261 = Equal?(x=w1666, y=w1665) -> (x = y?=w1664:cluster{"Left":bool, "Top":bool})
            n1262 = Equal?(x=w1657, y=w1658) -> (x = y?=w1659:cluster{"Left":bool, "Top":bool})
            n1263 = Unbundle By Name(w1647) -> ("Left"=w1649:bool, "Top"=w1648:bool)
            n1264 = Unbundle By Name(w1652) -> ("Left"=w1650:bool, "Top"=w1651:bool)
            n1265 = Unbundle By Name(w1664) -> ("Left"=w1662:bool, "Top"=w1663:bool)
            n1266 = Unbundle By Name(w1659) -> ("Left"=w1661:bool, "Top"=w1660:bool)
            n1267 = And(x=w1649, y=w1648) -> (x .and. y?=w1640:bool)
            n1268 = And(x=w1650, y=w1651) -> (x .and. y?=w1639:bool)
            n1269 = And(x=w1662, y=w1663) -> (x .and. y?=w1642:bool)
            n1270 = And(x=w1661, y=w1660) -> (x .and. y?=w1641:bool)
            n1271 = Compound Arithmetic op=OR(w1642, w1641, w1640, w1639) -> (w1643:bool)
            n1272 = case shown="True" w1643 {
              tunnel: w1638 -> [_ w1668]
              frame False {
              }
              frame True {
                n1273 = flat-sequence {
                  tunnel: w1668 -> [w1669]
                  frame #0 {
                    n1274 = local write "Temp Position"(w1669) -> ()
                  }
                  frame #1 {
                    n1275 = local read "Empty"() -> (w1670:cluster{"Left":dbl, "Top":dbl})
                    n1276 = property on="Key 12" class="Bool"("Position"=w1670) -> ()  [unwired: 2 in, 2 out]
                  }
                  frame #2 {
                    n1277 = local read "Temp Position"() -> (w1671:cluster{"Left":dbl, "Top":dbl})
                    n1278 = local write "Empty"(w1671) -> ()
                  }
                }
              }
            }
          }
          frame #1 {
            n1279 = property on="Key 5" class="Bool"() -> ("Position"=w1760:T1)  [unwired: 2 in, 2 out]
            n1280 = property on="Key 1" class="Bool"() -> ("Position"=w1763:T1)  [unwired: 2 in, 2 out]
            n1281 = property on="Key 9" class="Bool"() -> ("Position"=w1753:T1)  [unwired: 2 in, 2 out]
            n1282 = property on="Key 13" class="Bool"() -> ("Position"=w1750:T1)  [unwired: 2 in, 2 out]
            n1283 = Equal?(x=w1760, y=T1 {"Left"=0, "Top"=80} ("Position")) -> (x = y?=w1757:cluster{"Left":bool, "Top":bool})
            n1284 = Equal?(x=w1763, y=T1 {"Left"=0, "Top"=0} ("Position")) -> (x = y?=w1766:cluster{"Left":bool, "Top":bool})
            n1285 = Equal?(x=w1753, y=T1 {"Left"=0, "Top"=160} ("Position")) -> (x = y?=w1756:cluster{"Left":bool, "Top":bool})
            n1286 = Equal?(x=w1750, y=T1 {"Left"=0, "Top"=240} ("Position")) -> (x = y?=w1747:cluster{"Left":bool, "Top":bool})
            n1287 = Unbundle By Name(w1757) -> ("Left"=w1759:bool, "Top"=w1758:bool)
            n1288 = Unbundle By Name(w1766) -> ("Left"=w1764:bool, "Top"=w1765:bool)
            n1289 = Unbundle By Name(w1756) -> ("Left"=w1754:bool, "Top"=w1755:bool)
            n1290 = Unbundle By Name(w1747) -> ("Left"=w1749:bool, "Top"=w1748:bool)
            n1291 = And(x=w1759, y=w1758) -> (x .and. y?=w1690:bool)
            n1292 = And(x=w1764, y=w1765) -> (x .and. y?=w1691:bool)
            n1293 = And(x=w1754, y=w1755) -> (x .and. y?=w1689:bool)
            n1294 = And(x=w1749, y=w1748) -> (x .and. y?=w1688:bool)
            n1295 = Compound Arithmetic op=AND(w1691, w1690, w1689, w1688) -> (w1676:bool)
            n1296 = property on="Key 6" class="Bool"() -> ("Position"=w1733:T1)  [unwired: 2 in, 2 out]
            n1297 = property on="Key 2" class="Bool"() -> ("Position"=w1730:T1)  [unwired: 2 in, 2 out]
            n1298 = property on="Key 10" class="Bool"() -> ("Position"=w1740:T1)  [unwired: 2 in, 2 out]
            n1299 = property on="Key 14" class="Bool"() -> ("Position"=w1743:T1)  [unwired: 2 in, 2 out]
            n1300 = Equal?(x=w1733, y=T1 {"Left"=80, "Top"=80} ("Position")) -> (x = y?=w1736:cluster{"Left":bool, "Top":bool})
            n1301 = Equal?(x=w1730, y=T1 {"Left"=80, "Top"=0} ("Position")) -> (x = y?=w1727:cluster{"Left":bool, "Top":bool})
            n1302 = Equal?(x=w1740, y=T1 {"Left"=80, "Top"=160} ("Position")) -> (x = y?=w1737:cluster{"Left":bool, "Top":bool})
            n1303 = Equal?(x=w1743, y=T1 {"Left"=80, "Top"=240} ("Position")) -> (x = y?=w1746:cluster{"Left":bool, "Top":bool})
            n1304 = Unbundle By Name(w1736) -> ("Left"=w1734:bool, "Top"=w1735:bool)
            n1305 = Unbundle By Name(w1727) -> ("Left"=w1729:bool, "Top"=w1728:bool)
            n1306 = Unbundle By Name(w1737) -> ("Left"=w1739:bool, "Top"=w1738:bool)
            n1307 = Unbundle By Name(w1746) -> ("Left"=w1744:bool, "Top"=w1745:bool)
            n1308 = And(x=w1734, y=w1735) -> (x .and. y?=w1686:bool)
            n1309 = And(x=w1729, y=w1728) -> (x .and. y?=w1687:bool)
            n1310 = And(x=w1739, y=w1738) -> (x .and. y?=w1685:bool)
            n1311 = And(x=w1744, y=w1745) -> (x .and. y?=w1684:bool)
            n1312 = Compound Arithmetic op=AND(w1687, w1686, w1685, w1684) -> (w1675:bool)
            n1313 = property on="Key 7" class="Bool"() -> ("Position"=w1720:T1)  [unwired: 2 in, 2 out]
            n1314 = property on="Key 3" class="Bool"() -> ("Position"=w1723:T1)  [unwired: 2 in, 2 out]
            n1315 = property on="Key 11" class="Bool"() -> ("Position"=w1713:T1)  [unwired: 2 in, 2 out]
            n1316 = property on="Key 15" class="Bool"() -> ("Position"=w1710:T1)  [unwired: 2 in, 2 out]
            n1317 = Equal?(x=w1720, y=T1 {"Left"=160, "Top"=80} ("Position")) -> (x = y?=w1717:cluster{"Left":bool, "Top":bool})
            n1318 = Equal?(x=w1723, y=T1 {"Left"=160, "Top"=0} ("Position")) -> (x = y?=w1726:cluster{"Left":bool, "Top":bool})
            n1319 = Equal?(x=w1713, y=T1 {"Left"=160, "Top"=160} ("Position")) -> (x = y?=w1716:cluster{"Left":bool, "Top":bool})
            n1320 = Equal?(x=w1710, y=T1 {"Left"=160, "Top"=240} ("Position")) -> (x = y?=w1707:cluster{"Left":bool, "Top":bool})
            n1321 = Unbundle By Name(w1717) -> ("Left"=w1719:bool, "Top"=w1718:bool)
            n1322 = Unbundle By Name(w1726) -> ("Left"=w1724:bool, "Top"=w1725:bool)
            n1323 = Unbundle By Name(w1716) -> ("Left"=w1714:bool, "Top"=w1715:bool)
            n1324 = Unbundle By Name(w1707) -> ("Left"=w1709:bool, "Top"=w1708:bool)
            n1325 = And(x=w1719, y=w1718) -> (x .and. y?=w1682:bool)
            n1326 = And(x=w1724, y=w1725) -> (x .and. y?=w1683:bool)
            n1327 = And(x=w1714, y=w1715) -> (x .and. y?=w1681:bool)
            n1328 = And(x=w1709, y=w1708) -> (x .and. y?=w1680:bool)
            n1329 = Compound Arithmetic op=AND(w1683, w1682, w1681, w1680) -> (w1674:bool)
            n1330 = property on="Key 8" class="Bool"() -> ("Position"=w1698:T1)  [unwired: 2 in, 2 out]
            n1331 = property on="Key 4" class="Bool"() -> ("Position"=w1695:T1)  [unwired: 2 in, 2 out]
            n1332 = property on="Key 12" class="Bool"() -> ("Position"=w1705:T1)  [unwired: 2 in, 2 out]
            n1333 = Equal?(x=w1698, y=T1 {"Left"=240, "Top"=80} ("Position")) -> (x = y?=w1701:cluster{"Left":bool, "Top":bool})
            n1334 = Equal?(x=w1695, y=T1 {"Left"=240, "Top"=0} ("Position")) -> (x = y?=w1692:cluster{"Left":bool, "Top":bool})
            n1335 = Equal?(x=w1705, y=T1 {"Left"=240, "Top"=160} ("Position")) -> (x = y?=w1702:cluster{"Left":bool, "Top":bool})
            n1336 = Unbundle By Name(w1701) -> ("Left"=w1699:bool, "Top"=w1700:bool)
            n1337 = Unbundle By Name(w1692) -> ("Left"=w1694:bool, "Top"=w1693:bool)
            n1338 = Unbundle By Name(w1702) -> ("Left"=w1704:bool, "Top"=w1703:bool)
            n1339 = And(x=w1699, y=w1700) -> (x .and. y?=w1678:bool)
            n1340 = And(x=w1694, y=w1693) -> (x .and. y?=w1679:bool)
            n1341 = And(x=w1704, y=w1703) -> (x .and. y?=w1677:bool)
            n1342 = Compound Arithmetic op=AND(w1679, w1678, w1677) -> (w1673:bool)
            n1343 = Compound Arithmetic op=AND(w1676, w1675, w1674, w1673) -> (w1672:bool)
            n1344 = local write "Result"(w1672) -> ()
            n1345 = property on="Result" class="Bool (strict)"("Val(Sgnl)"=w1672) -> ()  [unwired: 2 in, 2 out]
          }
        }
      }
      event "Key 13": Value Change {
        n1346 = event-data() -> ()  [unwired: 1 in, 6 out]
        n1347 = stacked-sequence {
          frame #0 {
            n1348 = local read "Moves Number"() -> (w1767:dbl)
            n1349 = property on="Key 13" class="Bool"() -> ("Position"=w1769:T1)  [unwired: 2 in, 2 out]
            n1350 = Increment(x=w1767) -> (x+1=w1768:dbl)
            n1351 = local read "Empty"() -> (w1777:cluster{"Left":dbl, "Top":dbl})
            n1352 = local read "Empty"() -> (w1784:cluster{"Left":dbl, "Top":dbl})
            n1353 = local read "Empty"() -> (w1796:cluster{"Left":dbl, "Top":dbl})
            n1354 = local read "Empty"() -> (w1789:cluster{"Left":dbl, "Top":dbl})
            n1355 = Add(x=w1769, y=T1 {"Left"=80, "Top"=0} ("Position")) -> (x+y=w1776:T1)
            n1356 = Add(x=w1769, y=T1 {"Left"=0, "Top"=80} ("Position")) -> (x+y=w1785:T1)
            n1357 = Subtract(x=w1769, y=T1 {"Left"=80, "Top"=0} ("Position")) -> (x-y=w1797:T1)
            n1358 = Subtract(x=w1769, y=T1 {"Left"=0, "Top"=80} ("Position")) -> (x-y=w1788:T1)
            n1359 = local write "Moves Number"(w1768) -> ()
            n1360 = Equal?(x=w1776, y=w1777) -> (x = y?=w1778:cluster{"Left":bool, "Top":bool})
            n1361 = Equal?(x=w1785, y=w1784) -> (x = y?=w1783:cluster{"Left":bool, "Top":bool})
            n1362 = Equal?(x=w1797, y=w1796) -> (x = y?=w1795:cluster{"Left":bool, "Top":bool})
            n1363 = Equal?(x=w1788, y=w1789) -> (x = y?=w1790:cluster{"Left":bool, "Top":bool})
            n1364 = Unbundle By Name(w1778) -> ("Left"=w1780:bool, "Top"=w1779:bool)
            n1365 = Unbundle By Name(w1783) -> ("Left"=w1781:bool, "Top"=w1782:bool)
            n1366 = Unbundle By Name(w1795) -> ("Left"=w1793:bool, "Top"=w1794:bool)
            n1367 = Unbundle By Name(w1790) -> ("Left"=w1792:bool, "Top"=w1791:bool)
            n1368 = And(x=w1780, y=w1779) -> (x .and. y?=w1771:bool)
            n1369 = And(x=w1781, y=w1782) -> (x .and. y?=w1770:bool)
            n1370 = And(x=w1793, y=w1794) -> (x .and. y?=w1773:bool)
            n1371 = And(x=w1792, y=w1791) -> (x .and. y?=w1772:bool)
            n1372 = Compound Arithmetic op=OR(w1773, w1772, w1771, w1770) -> (w1774:bool)
            n1373 = case shown="True" w1774 {
              tunnel: w1769 -> [_ w1799]
              frame False {
              }
              frame True {
                n1374 = flat-sequence {
                  tunnel: w1799 -> [w1800]
                  frame #0 {
                    n1375 = local write "Temp Position"(w1800) -> ()
                  }
                  frame #1 {
                    n1376 = local read "Empty"() -> (w1801:cluster{"Left":dbl, "Top":dbl})
                    n1377 = property on="Key 13" class="Bool"("Position"=w1801) -> ()  [unwired: 2 in, 2 out]
                  }
                  frame #2 {
                    n1378 = local read "Temp Position"() -> (w1802:cluster{"Left":dbl, "Top":dbl})
                    n1379 = local write "Empty"(w1802) -> ()
                  }
                }
              }
            }
          }
          frame #1 {
            n1380 = property on="Key 5" class="Bool"() -> ("Position"=w1891:T1)  [unwired: 2 in, 2 out]
            n1381 = property on="Key 1" class="Bool"() -> ("Position"=w1894:T1)  [unwired: 2 in, 2 out]
            n1382 = property on="Key 9" class="Bool"() -> ("Position"=w1884:T1)  [unwired: 2 in, 2 out]
            n1383 = property on="Key 13" class="Bool"() -> ("Position"=w1881:T1)  [unwired: 2 in, 2 out]
            n1384 = Equal?(x=w1891, y=T1 {"Left"=0, "Top"=80} ("Position")) -> (x = y?=w1888:cluster{"Left":bool, "Top":bool})
            n1385 = Equal?(x=w1894, y=T1 {"Left"=0, "Top"=0} ("Position")) -> (x = y?=w1897:cluster{"Left":bool, "Top":bool})
            n1386 = Equal?(x=w1884, y=T1 {"Left"=0, "Top"=160} ("Position")) -> (x = y?=w1887:cluster{"Left":bool, "Top":bool})
            n1387 = Equal?(x=w1881, y=T1 {"Left"=0, "Top"=240} ("Position")) -> (x = y?=w1878:cluster{"Left":bool, "Top":bool})
            n1388 = Unbundle By Name(w1888) -> ("Left"=w1890:bool, "Top"=w1889:bool)
            n1389 = Unbundle By Name(w1897) -> ("Left"=w1895:bool, "Top"=w1896:bool)
            n1390 = Unbundle By Name(w1887) -> ("Left"=w1885:bool, "Top"=w1886:bool)
            n1391 = Unbundle By Name(w1878) -> ("Left"=w1880:bool, "Top"=w1879:bool)
            n1392 = And(x=w1890, y=w1889) -> (x .and. y?=w1821:bool)
            n1393 = And(x=w1895, y=w1896) -> (x .and. y?=w1822:bool)
            n1394 = And(x=w1885, y=w1886) -> (x .and. y?=w1820:bool)
            n1395 = And(x=w1880, y=w1879) -> (x .and. y?=w1819:bool)
            n1396 = Compound Arithmetic op=AND(w1822, w1821, w1820, w1819) -> (w1807:bool)
            n1397 = property on="Key 6" class="Bool"() -> ("Position"=w1864:T1)  [unwired: 2 in, 2 out]
            n1398 = property on="Key 2" class="Bool"() -> ("Position"=w1861:T1)  [unwired: 2 in, 2 out]
            n1399 = property on="Key 10" class="Bool"() -> ("Position"=w1871:T1)  [unwired: 2 in, 2 out]
            n1400 = property on="Key 14" class="Bool"() -> ("Position"=w1874:T1)  [unwired: 2 in, 2 out]
            n1401 = Equal?(x=w1864, y=T1 {"Left"=80, "Top"=80} ("Position")) -> (x = y?=w1867:cluster{"Left":bool, "Top":bool})
            n1402 = Equal?(x=w1861, y=T1 {"Left"=80, "Top"=0} ("Position")) -> (x = y?=w1858:cluster{"Left":bool, "Top":bool})
            n1403 = Equal?(x=w1871, y=T1 {"Left"=80, "Top"=160} ("Position")) -> (x = y?=w1868:cluster{"Left":bool, "Top":bool})
            n1404 = Equal?(x=w1874, y=T1 {"Left"=80, "Top"=240} ("Position")) -> (x = y?=w1877:cluster{"Left":bool, "Top":bool})
            n1405 = Unbundle By Name(w1867) -> ("Left"=w1865:bool, "Top"=w1866:bool)
            n1406 = Unbundle By Name(w1858) -> ("Left"=w1860:bool, "Top"=w1859:bool)
            n1407 = Unbundle By Name(w1868) -> ("Left"=w1870:bool, "Top"=w1869:bool)
            n1408 = Unbundle By Name(w1877) -> ("Left"=w1875:bool, "Top"=w1876:bool)
            n1409 = And(x=w1865, y=w1866) -> (x .and. y?=w1817:bool)
            n1410 = And(x=w1860, y=w1859) -> (x .and. y?=w1818:bool)
            n1411 = And(x=w1870, y=w1869) -> (x .and. y?=w1816:bool)
            n1412 = And(x=w1875, y=w1876) -> (x .and. y?=w1815:bool)
            n1413 = Compound Arithmetic op=AND(w1818, w1817, w1816, w1815) -> (w1806:bool)
            n1414 = property on="Key 7" class="Bool"() -> ("Position"=w1851:T1)  [unwired: 2 in, 2 out]
            n1415 = property on="Key 3" class="Bool"() -> ("Position"=w1854:T1)  [unwired: 2 in, 2 out]
            n1416 = property on="Key 11" class="Bool"() -> ("Position"=w1844:T1)  [unwired: 2 in, 2 out]
            n1417 = property on="Key 15" class="Bool"() -> ("Position"=w1841:T1)  [unwired: 2 in, 2 out]
            n1418 = Equal?(x=w1851, y=T1 {"Left"=160, "Top"=80} ("Position")) -> (x = y?=w1848:cluster{"Left":bool, "Top":bool})
            n1419 = Equal?(x=w1854, y=T1 {"Left"=160, "Top"=0} ("Position")) -> (x = y?=w1857:cluster{"Left":bool, "Top":bool})
            n1420 = Equal?(x=w1844, y=T1 {"Left"=160, "Top"=160} ("Position")) -> (x = y?=w1847:cluster{"Left":bool, "Top":bool})
            n1421 = Equal?(x=w1841, y=T1 {"Left"=160, "Top"=240} ("Position")) -> (x = y?=w1838:cluster{"Left":bool, "Top":bool})
            n1422 = Unbundle By Name(w1848) -> ("Left"=w1850:bool, "Top"=w1849:bool)
            n1423 = Unbundle By Name(w1857) -> ("Left"=w1855:bool, "Top"=w1856:bool)
            n1424 = Unbundle By Name(w1847) -> ("Left"=w1845:bool, "Top"=w1846:bool)
            n1425 = Unbundle By Name(w1838) -> ("Left"=w1840:bool, "Top"=w1839:bool)
            n1426 = And(x=w1850, y=w1849) -> (x .and. y?=w1813:bool)
            n1427 = And(x=w1855, y=w1856) -> (x .and. y?=w1814:bool)
            n1428 = And(x=w1845, y=w1846) -> (x .and. y?=w1812:bool)
            n1429 = And(x=w1840, y=w1839) -> (x .and. y?=w1811:bool)
            n1430 = Compound Arithmetic op=AND(w1814, w1813, w1812, w1811) -> (w1805:bool)
            n1431 = property on="Key 8" class="Bool"() -> ("Position"=w1829:T1)  [unwired: 2 in, 2 out]
            n1432 = property on="Key 4" class="Bool"() -> ("Position"=w1826:T1)  [unwired: 2 in, 2 out]
            n1433 = property on="Key 12" class="Bool"() -> ("Position"=w1836:T1)  [unwired: 2 in, 2 out]
            n1434 = Equal?(x=w1829, y=T1 {"Left"=240, "Top"=80} ("Position")) -> (x = y?=w1832:cluster{"Left":bool, "Top":bool})
            n1435 = Equal?(x=w1826, y=T1 {"Left"=240, "Top"=0} ("Position")) -> (x = y?=w1823:cluster{"Left":bool, "Top":bool})
            n1436 = Equal?(x=w1836, y=T1 {"Left"=240, "Top"=160} ("Position")) -> (x = y?=w1833:cluster{"Left":bool, "Top":bool})
            n1437 = Unbundle By Name(w1832) -> ("Left"=w1830:bool, "Top"=w1831:bool)
            n1438 = Unbundle By Name(w1823) -> ("Left"=w1825:bool, "Top"=w1824:bool)
            n1439 = Unbundle By Name(w1833) -> ("Left"=w1835:bool, "Top"=w1834:bool)
            n1440 = And(x=w1830, y=w1831) -> (x .and. y?=w1809:bool)
            n1441 = And(x=w1825, y=w1824) -> (x .and. y?=w1810:bool)
            n1442 = And(x=w1835, y=w1834) -> (x .and. y?=w1808:bool)
            n1443 = Compound Arithmetic op=AND(w1810, w1809, w1808) -> (w1804:bool)
            n1444 = Compound Arithmetic op=AND(w1807, w1806, w1805, w1804) -> (w1803:bool)
            n1445 = local write "Result"(w1803) -> ()
            n1446 = property on="Result" class="Bool (strict)"("Val(Sgnl)"=w1803) -> ()  [unwired: 2 in, 2 out]
          }
        }
      }
      event "Key 14": Value Change {
        n1447 = event-data() -> ()  [unwired: 1 in, 6 out]
        n1448 = stacked-sequence {
          frame #0 {
            n1449 = local read "Moves Number"() -> (w1898:dbl)
            n1450 = property on="Key 14" class="Bool"() -> ("Position"=w1900:T1)  [unwired: 2 in, 2 out]
            n1451 = Increment(x=w1898) -> (x+1=w1899:dbl)
            n1452 = local read "Empty"() -> (w1908:cluster{"Left":dbl, "Top":dbl})
            n1453 = local read "Empty"() -> (w1915:cluster{"Left":dbl, "Top":dbl})
            n1454 = local read "Empty"() -> (w1927:cluster{"Left":dbl, "Top":dbl})
            n1455 = local read "Empty"() -> (w1920:cluster{"Left":dbl, "Top":dbl})
            n1456 = Add(x=w1900, y=T1 {"Left"=80, "Top"=0} ("Position")) -> (x+y=w1907:T1)
            n1457 = Add(x=w1900, y=T1 {"Left"=0, "Top"=80} ("Position")) -> (x+y=w1916:T1)
            n1458 = Subtract(x=w1900, y=T1 {"Left"=80, "Top"=0} ("Position")) -> (x-y=w1928:T1)
            n1459 = Subtract(x=w1900, y=T1 {"Left"=0, "Top"=80} ("Position")) -> (x-y=w1919:T1)
            n1460 = local write "Moves Number"(w1899) -> ()
            n1461 = Equal?(x=w1907, y=w1908) -> (x = y?=w1909:cluster{"Left":bool, "Top":bool})
            n1462 = Equal?(x=w1916, y=w1915) -> (x = y?=w1914:cluster{"Left":bool, "Top":bool})
            n1463 = Equal?(x=w1928, y=w1927) -> (x = y?=w1926:cluster{"Left":bool, "Top":bool})
            n1464 = Equal?(x=w1919, y=w1920) -> (x = y?=w1921:cluster{"Left":bool, "Top":bool})
            n1465 = Unbundle By Name(w1909) -> ("Left"=w1911:bool, "Top"=w1910:bool)
            n1466 = Unbundle By Name(w1914) -> ("Left"=w1912:bool, "Top"=w1913:bool)
            n1467 = Unbundle By Name(w1926) -> ("Left"=w1924:bool, "Top"=w1925:bool)
            n1468 = Unbundle By Name(w1921) -> ("Left"=w1923:bool, "Top"=w1922:bool)
            n1469 = And(x=w1911, y=w1910) -> (x .and. y?=w1902:bool)
            n1470 = And(x=w1912, y=w1913) -> (x .and. y?=w1901:bool)
            n1471 = And(x=w1924, y=w1925) -> (x .and. y?=w1904:bool)
            n1472 = And(x=w1923, y=w1922) -> (x .and. y?=w1903:bool)
            n1473 = Compound Arithmetic op=OR(w1904, w1903, w1902, w1901) -> (w1905:bool)
            n1474 = case shown="True" w1905 {
              tunnel: w1900 -> [_ w1930]
              frame False {
              }
              frame True {
                n1475 = flat-sequence {
                  tunnel: w1930 -> [w1931]
                  frame #0 {
                    n1476 = local write "Temp Position"(w1931) -> ()
                  }
                  frame #1 {
                    n1477 = local read "Empty"() -> (w1932:cluster{"Left":dbl, "Top":dbl})
                    n1478 = property on="Key 14" class="Bool"("Position"=w1932) -> ()  [unwired: 2 in, 2 out]
                  }
                  frame #2 {
                    n1479 = local read "Temp Position"() -> (w1933:cluster{"Left":dbl, "Top":dbl})
                    n1480 = local write "Empty"(w1933) -> ()
                  }
                }
              }
            }
          }
          frame #1 {
            n1481 = property on="Key 5" class="Bool"() -> ("Position"=w2022:T1)  [unwired: 2 in, 2 out]
            n1482 = property on="Key 1" class="Bool"() -> ("Position"=w2025:T1)  [unwired: 2 in, 2 out]
            n1483 = property on="Key 9" class="Bool"() -> ("Position"=w2015:T1)  [unwired: 2 in, 2 out]
            n1484 = property on="Key 13" class="Bool"() -> ("Position"=w2012:T1)  [unwired: 2 in, 2 out]
            n1485 = Equal?(x=w2022, y=T1 {"Left"=0, "Top"=80} ("Position")) -> (x = y?=w2019:cluster{"Left":bool, "Top":bool})
            n1486 = Equal?(x=w2025, y=T1 {"Left"=0, "Top"=0} ("Position")) -> (x = y?=w2028:cluster{"Left":bool, "Top":bool})
            n1487 = Equal?(x=w2015, y=T1 {"Left"=0, "Top"=160} ("Position")) -> (x = y?=w2018:cluster{"Left":bool, "Top":bool})
            n1488 = Equal?(x=w2012, y=T1 {"Left"=0, "Top"=240} ("Position")) -> (x = y?=w2009:cluster{"Left":bool, "Top":bool})
            n1489 = Unbundle By Name(w2019) -> ("Left"=w2021:bool, "Top"=w2020:bool)
            n1490 = Unbundle By Name(w2028) -> ("Left"=w2026:bool, "Top"=w2027:bool)
            n1491 = Unbundle By Name(w2018) -> ("Left"=w2016:bool, "Top"=w2017:bool)
            n1492 = Unbundle By Name(w2009) -> ("Left"=w2011:bool, "Top"=w2010:bool)
            n1493 = And(x=w2021, y=w2020) -> (x .and. y?=w1952:bool)
            n1494 = And(x=w2026, y=w2027) -> (x .and. y?=w1953:bool)
            n1495 = And(x=w2016, y=w2017) -> (x .and. y?=w1951:bool)
            n1496 = And(x=w2011, y=w2010) -> (x .and. y?=w1950:bool)
            n1497 = Compound Arithmetic op=AND(w1953, w1952, w1951, w1950) -> (w1938:bool)
            n1498 = property on="Key 6" class="Bool"() -> ("Position"=w1995:T1)  [unwired: 2 in, 2 out]
            n1499 = property on="Key 2" class="Bool"() -> ("Position"=w1992:T1)  [unwired: 2 in, 2 out]
            n1500 = property on="Key 10" class="Bool"() -> ("Position"=w2002:T1)  [unwired: 2 in, 2 out]
            n1501 = property on="Key 14" class="Bool"() -> ("Position"=w2005:T1)  [unwired: 2 in, 2 out]
            n1502 = Equal?(x=w1995, y=T1 {"Left"=80, "Top"=80} ("Position")) -> (x = y?=w1998:cluster{"Left":bool, "Top":bool})
            n1503 = Equal?(x=w1992, y=T1 {"Left"=80, "Top"=0} ("Position")) -> (x = y?=w1989:cluster{"Left":bool, "Top":bool})
            n1504 = Equal?(x=w2002, y=T1 {"Left"=80, "Top"=160} ("Position")) -> (x = y?=w1999:cluster{"Left":bool, "Top":bool})
            n1505 = Equal?(x=w2005, y=T1 {"Left"=80, "Top"=240} ("Position")) -> (x = y?=w2008:cluster{"Left":bool, "Top":bool})
            n1506 = Unbundle By Name(w1998) -> ("Left"=w1996:bool, "Top"=w1997:bool)
            n1507 = Unbundle By Name(w1989) -> ("Left"=w1991:bool, "Top"=w1990:bool)
            n1508 = Unbundle By Name(w1999) -> ("Left"=w2001:bool, "Top"=w2000:bool)
            n1509 = Unbundle By Name(w2008) -> ("Left"=w2006:bool, "Top"=w2007:bool)
            n1510 = And(x=w1996, y=w1997) -> (x .and. y?=w1948:bool)
            n1511 = And(x=w1991, y=w1990) -> (x .and. y?=w1949:bool)
            n1512 = And(x=w2001, y=w2000) -> (x .and. y?=w1947:bool)
            n1513 = And(x=w2006, y=w2007) -> (x .and. y?=w1946:bool)
            n1514 = Compound Arithmetic op=AND(w1949, w1948, w1947, w1946) -> (w1937:bool)
            n1515 = property on="Key 7" class="Bool"() -> ("Position"=w1982:T1)  [unwired: 2 in, 2 out]
            n1516 = property on="Key 3" class="Bool"() -> ("Position"=w1985:T1)  [unwired: 2 in, 2 out]
            n1517 = property on="Key 11" class="Bool"() -> ("Position"=w1975:T1)  [unwired: 2 in, 2 out]
            n1518 = property on="Key 15" class="Bool"() -> ("Position"=w1972:T1)  [unwired: 2 in, 2 out]
            n1519 = Equal?(x=w1982, y=T1 {"Left"=160, "Top"=80} ("Position")) -> (x = y?=w1979:cluster{"Left":bool, "Top":bool})
            n1520 = Equal?(x=w1985, y=T1 {"Left"=160, "Top"=0} ("Position")) -> (x = y?=w1988:cluster{"Left":bool, "Top":bool})
            n1521 = Equal?(x=w1975, y=T1 {"Left"=160, "Top"=160} ("Position")) -> (x = y?=w1978:cluster{"Left":bool, "Top":bool})
            n1522 = Equal?(x=w1972, y=T1 {"Left"=160, "Top"=240} ("Position")) -> (x = y?=w1969:cluster{"Left":bool, "Top":bool})
            n1523 = Unbundle By Name(w1979) -> ("Left"=w1981:bool, "Top"=w1980:bool)
            n1524 = Unbundle By Name(w1988) -> ("Left"=w1986:bool, "Top"=w1987:bool)
            n1525 = Unbundle By Name(w1978) -> ("Left"=w1976:bool, "Top"=w1977:bool)
            n1526 = Unbundle By Name(w1969) -> ("Left"=w1971:bool, "Top"=w1970:bool)
            n1527 = And(x=w1981, y=w1980) -> (x .and. y?=w1944:bool)
            n1528 = And(x=w1986, y=w1987) -> (x .and. y?=w1945:bool)
            n1529 = And(x=w1976, y=w1977) -> (x .and. y?=w1943:bool)
            n1530 = And(x=w1971, y=w1970) -> (x .and. y?=w1942:bool)
            n1531 = Compound Arithmetic op=AND(w1945, w1944, w1943, w1942) -> (w1936:bool)
            n1532 = property on="Key 8" class="Bool"() -> ("Position"=w1960:T1)  [unwired: 2 in, 2 out]
            n1533 = property on="Key 4" class="Bool"() -> ("Position"=w1957:T1)  [unwired: 2 in, 2 out]
            n1534 = property on="Key 12" class="Bool"() -> ("Position"=w1967:T1)  [unwired: 2 in, 2 out]
            n1535 = Equal?(x=w1960, y=T1 {"Left"=240, "Top"=80} ("Position")) -> (x = y?=w1963:cluster{"Left":bool, "Top":bool})
            n1536 = Equal?(x=w1957, y=T1 {"Left"=240, "Top"=0} ("Position")) -> (x = y?=w1954:cluster{"Left":bool, "Top":bool})
            n1537 = Equal?(x=w1967, y=T1 {"Left"=240, "Top"=160} ("Position")) -> (x = y?=w1964:cluster{"Left":bool, "Top":bool})
            n1538 = Unbundle By Name(w1963) -> ("Left"=w1961:bool, "Top"=w1962:bool)
            n1539 = Unbundle By Name(w1954) -> ("Left"=w1956:bool, "Top"=w1955:bool)
            n1540 = Unbundle By Name(w1964) -> ("Left"=w1966:bool, "Top"=w1965:bool)
            n1541 = And(x=w1961, y=w1962) -> (x .and. y?=w1940:bool)
            n1542 = And(x=w1956, y=w1955) -> (x .and. y?=w1941:bool)
            n1543 = And(x=w1966, y=w1965) -> (x .and. y?=w1939:bool)
            n1544 = Compound Arithmetic op=AND(w1941, w1940, w1939) -> (w1935:bool)
            n1545 = Compound Arithmetic op=AND(w1938, w1937, w1936, w1935) -> (w1934:bool)
            n1546 = local write "Result"(w1934) -> ()
            n1547 = property on="Result" class="Bool (strict)"("Val(Sgnl)"=w1934) -> ()  [unwired: 2 in, 2 out]
          }
        }
      }
      event "Key 15": Value Change {
        n1548 = event-data() -> ()  [unwired: 1 in, 6 out]
        n1549 = stacked-sequence {
          frame #0 {
            n1550 = local read "Moves Number"() -> (w2029:dbl)
            n1551 = property on="Key 15" class="Bool"() -> ("Position"=w2031:T1)  [unwired: 2 in, 2 out]
            n1552 = Increment(x=w2029) -> (x+1=w2030:dbl)
            n1553 = local read "Empty"() -> (w2039:cluster{"Left":dbl, "Top":dbl})
            n1554 = local read "Empty"() -> (w2046:cluster{"Left":dbl, "Top":dbl})
            n1555 = local read "Empty"() -> (w2058:cluster{"Left":dbl, "Top":dbl})
            n1556 = local read "Empty"() -> (w2051:cluster{"Left":dbl, "Top":dbl})
            n1557 = Add(x=w2031, y=T1 {"Left"=80, "Top"=0} ("Position")) -> (x+y=w2038:T1)
            n1558 = Add(x=w2031, y=T1 {"Left"=0, "Top"=80} ("Position")) -> (x+y=w2047:T1)
            n1559 = Subtract(x=w2031, y=T1 {"Left"=80, "Top"=0} ("Position")) -> (x-y=w2059:T1)
            n1560 = Subtract(x=w2031, y=T1 {"Left"=0, "Top"=80} ("Position")) -> (x-y=w2050:T1)
            n1561 = local write "Moves Number"(w2030) -> ()
            n1562 = Equal?(x=w2038, y=w2039) -> (x = y?=w2040:cluster{"Left":bool, "Top":bool})
            n1563 = Equal?(x=w2047, y=w2046) -> (x = y?=w2045:cluster{"Left":bool, "Top":bool})
            n1564 = Equal?(x=w2059, y=w2058) -> (x = y?=w2057:cluster{"Left":bool, "Top":bool})
            n1565 = Equal?(x=w2050, y=w2051) -> (x = y?=w2052:cluster{"Left":bool, "Top":bool})
            n1566 = Unbundle By Name(w2040) -> ("Left"=w2042:bool, "Top"=w2041:bool)
            n1567 = Unbundle By Name(w2045) -> ("Left"=w2043:bool, "Top"=w2044:bool)
            n1568 = Unbundle By Name(w2057) -> ("Left"=w2055:bool, "Top"=w2056:bool)
            n1569 = Unbundle By Name(w2052) -> ("Left"=w2054:bool, "Top"=w2053:bool)
            n1570 = And(x=w2042, y=w2041) -> (x .and. y?=w2033:bool)
            n1571 = And(x=w2043, y=w2044) -> (x .and. y?=w2032:bool)
            n1572 = And(x=w2055, y=w2056) -> (x .and. y?=w2035:bool)
            n1573 = And(x=w2054, y=w2053) -> (x .and. y?=w2034:bool)
            n1574 = Compound Arithmetic op=OR(w2035, w2034, w2033, w2032) -> (w2036:bool)
            n1575 = case shown="True" w2036 {
              tunnel: w2031 -> [_ w2061]
              frame False {
              }
              frame True {
                n1576 = flat-sequence {
                  tunnel: w2061 -> [w2062]
                  frame #0 {
                    n1577 = local write "Temp Position"(w2062) -> ()
                  }
                  frame #1 {
                    n1578 = local read "Empty"() -> (w2063:cluster{"Left":dbl, "Top":dbl})
                    n1579 = property on="Key 15" class="Bool"("Position"=w2063) -> ()  [unwired: 2 in, 2 out]
                  }
                  frame #2 {
                    n1580 = local read "Temp Position"() -> (w2064:cluster{"Left":dbl, "Top":dbl})
                    n1581 = local write "Empty"(w2064) -> ()
                  }
                }
              }
            }
          }
          frame #1 {
            n1582 = property on="Key 5" class="Bool"() -> ("Position"=w2153:T1)  [unwired: 2 in, 2 out]
            n1583 = property on="Key 1" class="Bool"() -> ("Position"=w2156:T1)  [unwired: 2 in, 2 out]
            n1584 = property on="Key 9" class="Bool"() -> ("Position"=w2146:T1)  [unwired: 2 in, 2 out]
            n1585 = property on="Key 13" class="Bool"() -> ("Position"=w2143:T1)  [unwired: 2 in, 2 out]
            n1586 = Equal?(x=w2153, y=T1 {"Left"=0, "Top"=80} ("Position")) -> (x = y?=w2150:cluster{"Left":bool, "Top":bool})
            n1587 = Equal?(x=w2156, y=T1 {"Left"=0, "Top"=0} ("Position")) -> (x = y?=w2159:cluster{"Left":bool, "Top":bool})
            n1588 = Equal?(x=w2146, y=T1 {"Left"=0, "Top"=160} ("Position")) -> (x = y?=w2149:cluster{"Left":bool, "Top":bool})
            n1589 = Equal?(x=w2143, y=T1 {"Left"=0, "Top"=240} ("Position")) -> (x = y?=w2140:cluster{"Left":bool, "Top":bool})
            n1590 = Unbundle By Name(w2150) -> ("Left"=w2152:bool, "Top"=w2151:bool)
            n1591 = Unbundle By Name(w2159) -> ("Left"=w2157:bool, "Top"=w2158:bool)
            n1592 = Unbundle By Name(w2149) -> ("Left"=w2147:bool, "Top"=w2148:bool)
            n1593 = Unbundle By Name(w2140) -> ("Left"=w2142:bool, "Top"=w2141:bool)
            n1594 = And(x=w2152, y=w2151) -> (x .and. y?=w2083:bool)
            n1595 = And(x=w2157, y=w2158) -> (x .and. y?=w2084:bool)
            n1596 = And(x=w2147, y=w2148) -> (x .and. y?=w2082:bool)
            n1597 = And(x=w2142, y=w2141) -> (x .and. y?=w2081:bool)
            n1598 = Compound Arithmetic op=AND(w2084, w2083, w2082, w2081) -> (w2069:bool)
            n1599 = property on="Key 6" class="Bool"() -> ("Position"=w2126:T1)  [unwired: 2 in, 2 out]
            n1600 = property on="Key 2" class="Bool"() -> ("Position"=w2123:T1)  [unwired: 2 in, 2 out]
            n1601 = property on="Key 10" class="Bool"() -> ("Position"=w2133:T1)  [unwired: 2 in, 2 out]
            n1602 = property on="Key 14" class="Bool"() -> ("Position"=w2136:T1)  [unwired: 2 in, 2 out]
            n1603 = Equal?(x=w2126, y=T1 {"Left"=80, "Top"=80} ("Position")) -> (x = y?=w2129:cluster{"Left":bool, "Top":bool})
            n1604 = Equal?(x=w2123, y=T1 {"Left"=80, "Top"=0} ("Position")) -> (x = y?=w2120:cluster{"Left":bool, "Top":bool})
            n1605 = Equal?(x=w2133, y=T1 {"Left"=80, "Top"=160} ("Position")) -> (x = y?=w2130:cluster{"Left":bool, "Top":bool})
            n1606 = Equal?(x=w2136, y=T1 {"Left"=80, "Top"=240} ("Position")) -> (x = y?=w2139:cluster{"Left":bool, "Top":bool})
            n1607 = Unbundle By Name(w2129) -> ("Left"=w2127:bool, "Top"=w2128:bool)
            n1608 = Unbundle By Name(w2120) -> ("Left"=w2122:bool, "Top"=w2121:bool)
            n1609 = Unbundle By Name(w2130) -> ("Left"=w2132:bool, "Top"=w2131:bool)
            n1610 = Unbundle By Name(w2139) -> ("Left"=w2137:bool, "Top"=w2138:bool)
            n1611 = And(x=w2127, y=w2128) -> (x .and. y?=w2079:bool)
            n1612 = And(x=w2122, y=w2121) -> (x .and. y?=w2080:bool)
            n1613 = And(x=w2132, y=w2131) -> (x .and. y?=w2078:bool)
            n1614 = And(x=w2137, y=w2138) -> (x .and. y?=w2077:bool)
            n1615 = Compound Arithmetic op=AND(w2080, w2079, w2078, w2077) -> (w2068:bool)
            n1616 = property on="Key 7" class="Bool"() -> ("Position"=w2113:T1)  [unwired: 2 in, 2 out]
            n1617 = property on="Key 3" class="Bool"() -> ("Position"=w2116:T1)  [unwired: 2 in, 2 out]
            n1618 = property on="Key 11" class="Bool"() -> ("Position"=w2106:T1)  [unwired: 2 in, 2 out]
            n1619 = property on="Key 15" class="Bool"() -> ("Position"=w2103:T1)  [unwired: 2 in, 2 out]
            n1620 = Equal?(x=w2113, y=T1 {"Left"=160, "Top"=80} ("Position")) -> (x = y?=w2110:cluster{"Left":bool, "Top":bool})
            n1621 = Equal?(x=w2116, y=T1 {"Left"=160, "Top"=0} ("Position")) -> (x = y?=w2119:cluster{"Left":bool, "Top":bool})
            n1622 = Equal?(x=w2106, y=T1 {"Left"=160, "Top"=160} ("Position")) -> (x = y?=w2109:cluster{"Left":bool, "Top":bool})
            n1623 = Equal?(x=w2103, y=T1 {"Left"=160, "Top"=240} ("Position")) -> (x = y?=w2100:cluster{"Left":bool, "Top":bool})
            n1624 = Unbundle By Name(w2110) -> ("Left"=w2112:bool, "Top"=w2111:bool)
            n1625 = Unbundle By Name(w2119) -> ("Left"=w2117:bool, "Top"=w2118:bool)
            n1626 = Unbundle By Name(w2109) -> ("Left"=w2107:bool, "Top"=w2108:bool)
            n1627 = Unbundle By Name(w2100) -> ("Left"=w2102:bool, "Top"=w2101:bool)
            n1628 = And(x=w2112, y=w2111) -> (x .and. y?=w2075:bool)
            n1629 = And(x=w2117, y=w2118) -> (x .and. y?=w2076:bool)
            n1630 = And(x=w2107, y=w2108) -> (x .and. y?=w2074:bool)
            n1631 = And(x=w2102, y=w2101) -> (x .and. y?=w2073:bool)
            n1632 = Compound Arithmetic op=AND(w2076, w2075, w2074, w2073) -> (w2067:bool)
            n1633 = property on="Key 8" class="Bool"() -> ("Position"=w2091:T1)  [unwired: 2 in, 2 out]
            n1634 = property on="Key 4" class="Bool"() -> ("Position"=w2088:T1)  [unwired: 2 in, 2 out]
            n1635 = property on="Key 12" class="Bool"() -> ("Position"=w2098:T1)  [unwired: 2 in, 2 out]
            n1636 = Equal?(x=w2091, y=T1 {"Left"=240, "Top"=80} ("Position")) -> (x = y?=w2094:cluster{"Left":bool, "Top":bool})
            n1637 = Equal?(x=w2088, y=T1 {"Left"=240, "Top"=0} ("Position")) -> (x = y?=w2085:cluster{"Left":bool, "Top":bool})
            n1638 = Equal?(x=w2098, y=T1 {"Left"=240, "Top"=160} ("Position")) -> (x = y?=w2095:cluster{"Left":bool, "Top":bool})
            n1639 = Unbundle By Name(w2094) -> ("Left"=w2092:bool, "Top"=w2093:bool)
            n1640 = Unbundle By Name(w2085) -> ("Left"=w2087:bool, "Top"=w2086:bool)
            n1641 = Unbundle By Name(w2095) -> ("Left"=w2097:bool, "Top"=w2096:bool)
            n1642 = And(x=w2092, y=w2093) -> (x .and. y?=w2071:bool)
            n1643 = And(x=w2087, y=w2086) -> (x .and. y?=w2072:bool)
            n1644 = And(x=w2097, y=w2096) -> (x .and. y?=w2070:bool)
            n1645 = Compound Arithmetic op=AND(w2072, w2071, w2070) -> (w2066:bool)
            n1646 = Compound Arithmetic op=AND(w2069, w2068, w2067, w2066) -> (w2065:bool)
            n1647 = local write "Result"(w2065) -> ()
            n1648 = property on="Result" class="Bool (strict)"("Val(Sgnl)"=w2065) -> ()  [unwired: 2 in, 2 out]
          }
        }
      }
      event "Result": Value Change {
        n1649 = event-data() -> ("NewVal"=w2160:bool)  [unwired: 1 in, 5 out]
        n1650 = case shown="True" w2160 {
          frame False {
          }
          frame True {
            n1651 = local write "Status"(enum16{"Idle", "Start", "Stop"}."Stop" ("Status")) -> ()
            n1652 = Two Button Dialog(message="You win the game.. Wanna play again?", 1:"No" ("T button name (\"OK\")"), 2:"Yes" ("T button name (\"OK\")")) -> (T button?=w2162:bool)
            n1653 = case shown="True" w2162 {
              selector: w2162 -> [_ w2167]
              frame False {
                n1654 = Stop(stop? (T)=TRUE) -> ()
              }
              frame True {
                n1655 = property on="New Game" class="Bool"("Val(Sgnl)"=w2167) -> ()  [unwired: 2 in, 2 out]
              }
            }
          }
        }
      }
      event "Stop": Value Change {
        n1656 = event-data() -> ()  [unwired: 1 in, 6 out]
        n1657 = Stop(stop? (T)=TRUE) -> ()
      }
    }
  }
  n1658 = while {
    stop <- FALSE stop-if-true
    # "Timer Loop"
    n1659 = local read "Status"() -> (w2173:enum16{"Idle", "Start", "Stop"})
    n1660 = feedback #1(0.0 ("Elapsed Time (s)")) -> (w2171:dbl)
    n1661 = case shown="\"Start\"" w2173 {
      tunnel: [w2176 w2178 w2185] -> w2172
      tunnel: w2171 -> [w2176 _ w2185]
      frame "Idle", Default {
      }
      frame "Start" {
        n1662 = flat-sequence {
          tunnel: [w2179] -> w2177
          tunnel: [w2183] -> w2178
          tunnel: w2177 -> [w2183]
          frame #0 {
            n1663 = local read "Reset"() -> (w2180:bool)
            n1664 = call "Elapsed Time"("Time Target (s)"=1000.0, "Reset"=w2180, "Auto Reset"=FALSE) -> ("Elapsed Time (s)"=w2179:dbl)  [unwired: 9 in, 7 out]
          }
          frame #1 {
            n1665 = local write "Reset"(FALSE ("Reset")) -> ()
          }
        }
      }
      frame "Stop" {
      }
    }
    n1666 = feedback-in #1(w2172) -> ()
    n1667 = local write "Elapsed Time (s)"(w2172) -> ()
    n1668 = Wait (ms)(milliseconds to wait=u32 50) -> ()  [unwired: 1 out]
  }
  "Result" <- FALSE ("Result")
  "Temp Position" <- cluster{"Left":dbl, "Top":dbl} {"Left"=0.0, "Top"=0.0} ("Temp Position")
  "Status" <- enum16{"Idle", "Start", "Stop"}."Idle" ("Enum")
  "Reset" <- TRUE ("Reset")
  "Moves Number" <- 0.0 ("Moves Number")
